vi "TLB Native Dynamic Events ver 0.18b.vi"() -> ()   [LabVIEW 2018]
uses:
  Labview Training Phase 2/Enum Controls/States for Action Engine.ctl
  TLB Type Definitions/State Type Definitions, for 0.26g versions and later 2.ctl
  TLB Type Definitions/Intruction Type Definitions.ctl
  TLB Type Definitions/Encoder cluster.ctl
  TLB Type Definitions/PING CLUSTER.ctl
  <vilib>/Studica/Studica Toolkit/NavX/NavX.lvlib
  <vilib>/Studica/Studica Toolkit/Background/DIO Channel.ctl
  Underlying VI's/NavX VI/navX type def.ctl
  <vilib>/Studica/Studica Toolkit/Background/I2C Channel.ctl
  TLB Type Definitions/Vision cluster.ctl
  <vilib>/NI_Real-Time Target Support.lvlib
  TLB Type Definitions/Stepper cluster.ctl
  Experimental VI's/Archived VI's/MOTOR CONTROL NO PID Type Def.ctl
  Underlying VI's/I2C Master VI/I2C MASTER Type Def.ctl
  Underlying VI's/I2C Master VI/I2C_MASTER_WRITE_NEW Type Def.ctl
  <vilib>/userdefined/High Color/IMAQdx.ctl
  Underlying VI's/I2C Master VI/Arduino_Interfacing.ctl
  TLB Type Definitions/Yaw Cluster.ctl
  TLB Type Definitions/Time cluster.ctl
  TLB Type Definitions/Y Stepper cluster.ctl
  Underlying VI's/Modified webcam FGV/Webcam AE.ctl
  Underlying VI's/Elasped Timer/Elapsed timer control.ctl
  Underlying VI's/Motor Control VI with PID/MOTOR CONTROL WITH PID AE DATA MODE TYPE DEF.ctl
  Underlying VI's/Motor Control VI with PID/MOTOR CONTROL WITH PID AE DIRECTION TYPE DEF.ctl
  TLB Type Definitions/IR Sensor Type Def.ctl
  <vilib>/myRIO/Common/Instrument Driver Framework/myRIO v1.0/AI/typedefs/AI Channels Enum.ctl
  <vilib>/myRIO/Common/Instrument Driver Framework/myRIO v1.0/AI/typedefs/AI Channels List.ctl
  TLB Type Definitions/Motor Speed Cluster.ctl
  Underlying VI's/IMAQ Create Reference AE/IMAQ Reference AE.ctl
  TLB Type Definitions/Line Sensor Cluster.ctl
  Underlying VI's/Line Sensor AE/Line Sensor AE Type Def.ctl
  <vilib>/Utility/RT CPU Load.ctl
panel:
  out "Arm IR Sensor":dbl
  out "Table obstruct":bool
  out "x-y":dbl
  out "Left IR Sensor":dbl
  out "Obstacle detected":bool
  out "Speed & distance":T1
  out "Object Center Coordinates":cluster{"x":sgl, "y":sgl}
  out "Object detection cluster":T2
  out "Time up flag":bool
  out "Task selection":u8
  in  "Object recognition mode":enum16{"Ball", "Soap", "Gel", "Pipe", "None"}(ring)
  out "NavX Readings":T3
  out "Arduino Data":T4
  out "CPU loads":T5[](array[typedef]) {"ISR (%)" format="%#.2f"; "Idle (%)" format="%#.2f"; "Background (%)" format="%#.2f"; "Normal (%)" format="%#.2f"; "Above Normal (%)" format="%#.2f"; "High (%)" format="%#.2g"; "Timed Structures (%)" format="%#.2g"; "Time Critical (%)" format="%#.2g"; "Total (%)" format="%#.2g"}
  out "TASK ENABLE":bool
  out "Rising Edge":bool
  in  "Green LED":bool
  out "I2C Error":errorcluster
  out "State Logic":T6=enum."Startup"
  out "elements":T7[](array[typedef])
  in  "STOP TASK":bool
  in  "OK Button":bool
  in  "STOP":bool
  out "error out":errorcluster
  out "Action Queue Items":i32
  out "State Logic Queue Items":i32
  out "Action Queues items":string[](array[string])=["Hardware reset", "Software reset", ""]
  out "Action State":string
  # "System Health Status Update"
  # "VISION"
  # "TLB FRAMEWORK STATUS"
  # "Test Programme written by Calvin Loke    Dated: 28 Aug 2019\nTest Programme revised by Dr Alex See   Dated 30 Aug 2019\n\nRevision date: 20/03/2020\nProgramme version:   TLB Native Dynamic Events ver 0.14a"
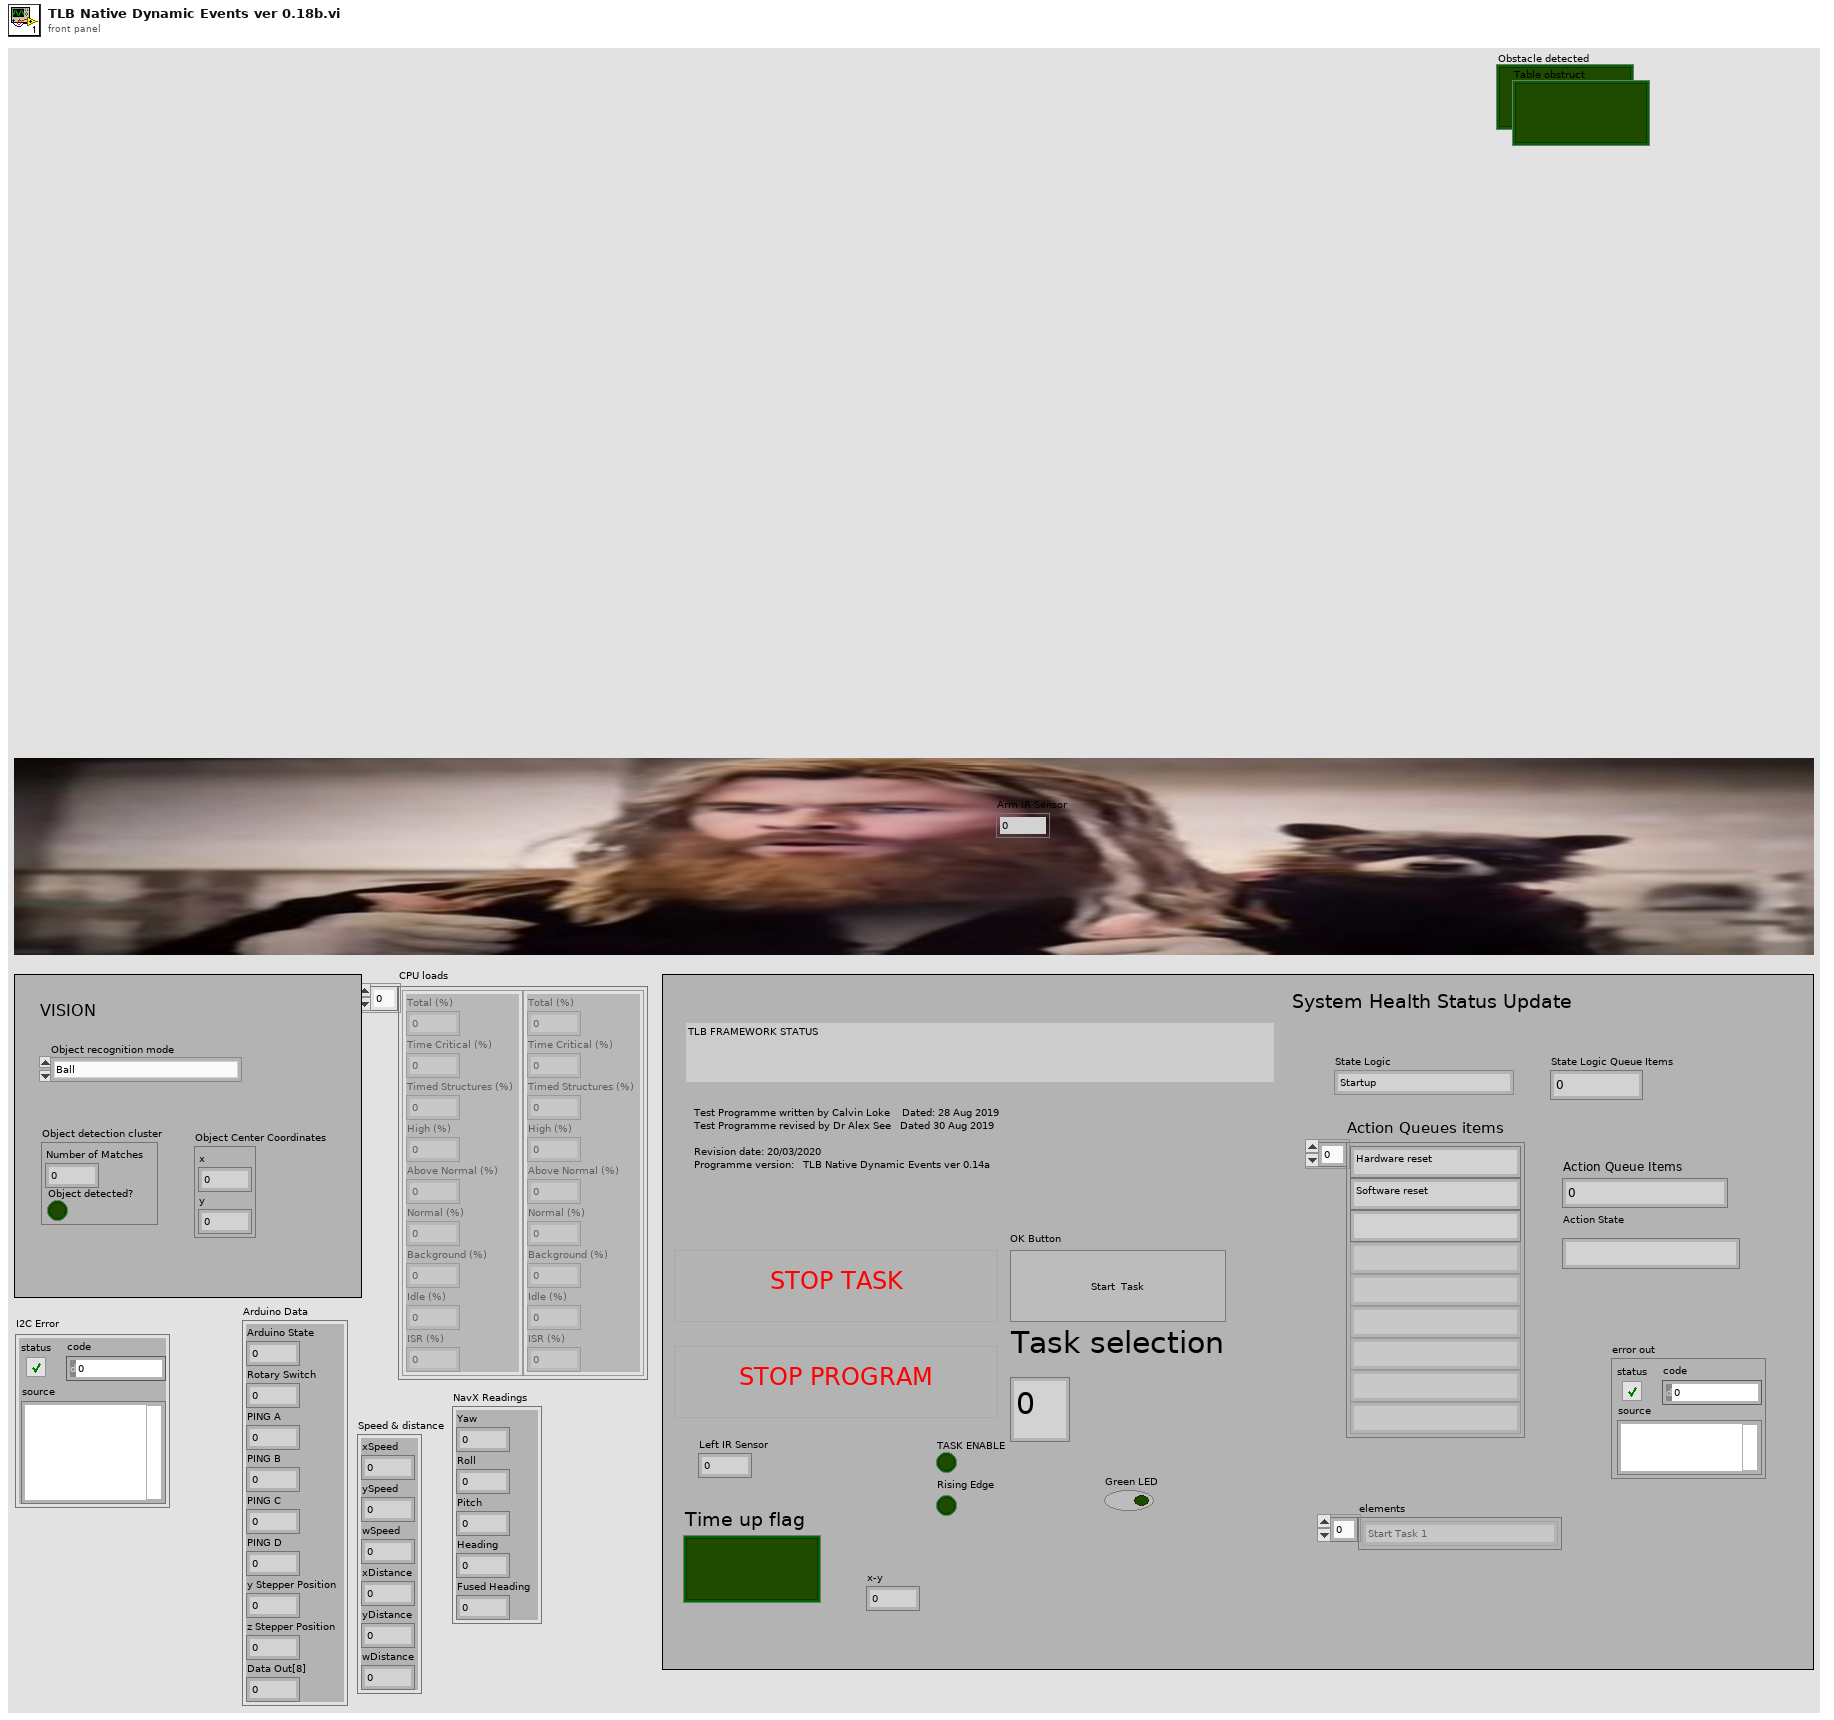
[diagram p1: front panel]
types:
  T1 = cluster{"xSpeed":dbl, "ySpeed":dbl, "wSpeed":dbl, "xDistance":dbl, "yDistance":dbl, "wDistance":dbl}
  T2 = cluster{"Number of Matches":i32, "Object detected?":bool}
  T3 = cluster{"Yaw":dbl, "Roll":dbl, "Pitch":dbl, "Heading":dbl, "Fused Heading":dbl}
  T4 = cluster{"Arduino State":u8, "Rotary Switch":u8, "PING A":u8, "PING B":u8, "PING C":u8, "PING D":u8, "y Stepper Position":u8, "z Stepper Position":u8, "Data Out[8]":u8}
  T5 = typedef "NI_Real-Time Target Support.lvlib/RT CPU Load.ctl" = cluster{"Total (%)":dbl, "Time Critical (%)":dbl, "Timed Structures (%)":dbl, "High (%)":dbl, "Above Normal (%)":dbl, "Normal (%)":dbl, "Background (%)":dbl, "Idle (%)":dbl, "ISR (%)":dbl}
  T6 = typedef "State Type Definitions, for 0.26g versions and later 2.ctl" = enum16{"None", "Startup", "Move to Angle", "True Stop", "Idle", "Shutdown", "Task 1A", "Task 1B", "Task 2:Raise Arm", "Task 2:Sensor Mode", "Task 2:Reverse Mode", "Task 3", "Task 4_A", "Task 4_B", "Task 4_C", "Task 4_D", "Task 5A", "Task 5B", "Task 5C", "Task 5D", "Task 5E: POSITION ARM", "Task 5F: ARM GRAB HEIGHT", "Task 5G: CLOSE CLAW", "Task 5H: RAISE ARM", "Task 6_A", "Task 6_B", "Task 7", "Task 8A: RAISE ARM", "Task 8B: MOVE TO BOX", "Task 8C: CAM BURST", "Task 8D: PROCESS IMAGE", "Task 8E: ROBOT ADJUST", "Task 8F: CAM BURST 2", "Task 8G: PROCESS IMAGE 2", "Task 8H: ARM ADJUST", "Task 8I: ARM GRAB HEIGHT", "Task 8J: CLOSE CLAW", "Task 8K: RAISE MY SWORD", "Task 9A: Raise Arm", "Task 9B: Rotate to Angle", "Task 9C: Detect Box", "Task 9D: MOVE FORWARD", "Task 9E: MOVE LEFT", "Task 9F: SCAN BOX", "Task 9G: MOVE RIGHT", "Task 9H: SCAN BOX 2", "Task 9I: ROTATE 90 CW", "Task 9J: FORWARD", "Task 9K: RAM WALL", "Task 9L: MOVE RIGHT", "Task 9M: SCAN BOX 3", "Task 9M: MOVE RIGHT", "Task 9N: SCAN BOX 4", "PENIS", "PENIS 2", "PENIS 3", "Task 9R: PROCESS COLOUR", "Task A1: Task 9 Open cam", "Task A2: Task 9 Move Arm", "Task A3: Task 9 Set Timer", "Task A4: Tasl 9 Capture images", "Task A5: Task 9 Close camera", "Task A6: Process Colour", "Task A7: Dispose Camera Buffer"}
  T7 = typedef "Intruction Type Definitions.ctl" = enum16{"None", "Start Task 1", "Start Task 2", "Start Task 3", "Start Task 4", "Start Task 5", "Start Task 6", "Start Task 7", "Start Task 8 - BALL", "Start Task 8 - Gel", "Start Task 8 - Pipe", "Start Task 8 - Soap", "Start Task 9", "Start Task A", "Start Task B", "Exit"}
  T8 = typedef "Line Sensor Cluster.ctl" = cluster{"Line Detected?":bool, "S1":dbl, "S2":dbl, "S3":dbl, "S4":dbl}
  T9 = typedef "Motor Speed Cluster.ctl" = cluster{"ySpeed":dbl, "xSpeed":dbl, "wSpeed":dbl}
  T10 = typedef "IR Sensor Type Def.ctl" = cluster{"Left IR Sensor":dbl, "Arm IR Sensor":dbl, "Bottom IR Sensor":dbl}
  T11 = typedef "Y Stepper cluster.ctl" = cluster{"yStepper desired":u8}
  T12 = typedef "Time cluster.ctl" = cluster{"Time up flag":bool, "SET TIME TO CHECK":dbl}
  T13 = typedef "Yaw Cluster.ctl" = cluster{"Yaw":dbl, "Compass":dbl}
  T14 = typedef "Stepper cluster.ctl" = cluster{"y Stepper Position":u8, "z Stepper Position":u8}
  T15 = typedef "DIO Channel.ctl" = enum16{"Not Connected", "A/DIO1", "A/DIO2", "A/DIO3", "A/DIO4", "A/DIO5", "A/DIO6", "A/DIO7", "A/DIO13", "B/DIO1", "B/DIO2", "B/DIO3", "B/DIO4", "B/DIO5", "B/DIO6", "B/DIO7", "B/DIO13", "C/DIO0", "C/DIO1", "C/DIO2", "C/DIO3", "C/DIO4", "C/DIO5", "C/DIO6", "C/DIO7"}
  T16 = typedef "Vision cluster.ctl" = cluster{"Recognized Object":bool, "Object X coordinate":dbl, "Object Y coordinate":dbl}
  T17 = typedef "PING CLUSTER.ctl" = cluster{"PING_A":u8, "PING_B":u8, "PING_C":u8, "PING_D":u8}
  T18 = typedef "Encoder cluster.ctl" = cluster{"xDistance":dbl, "yDistance":dbl, "wDistance":dbl}
  T19 = cluster{"DIO Channel":T15, "FPGA VI Reference Out":refnum<k20>}
  T20 = typedef "navX type def.ctl" = enum16{"Get i2C reference", "Read Values", "Zero Yaw"}
  T21 = typedef "Arduino_Interfacing.ctl" = enum16{"Initialize", "Write to Arduino", "Read From Arduino"}
  T22 = typedef "I2C Channel.ctl" = enum16{"Not Connected", "A", "B"}
  T23 = typedef "States for Action Engine.ctl" = enum16{"Initialize", "Write", "Read"}
  T24 = cluster{"I2C Ref Out":cluster{"I2C Channel":T22, "FPGA VI Reference Out":refnum<k20>}, "Connected":bool, "Slave Address (7-bit)":u8, "Registry":u8[]}
  T25 = typedef "Intruction Type Definitions.ctl" = enum16{"None", "Start Task 1", "Start Task 2", "Start Task 3", "Start Task 4", "Start Task 5", "Start Task 6", "Start Task 7", "Start Task 8", "Start Task 9", "Start Task A", "Start Task B", "Exit"}
  T26 = typedef "State Type Definitions.ctl" = enum16{"None", "Startup", "Move to Angle", "True Stop", "Idle", "Shutdown", "Task 1", "Task 2:Raise Arm", "Task 2:Sensor Mode", "Task 2:Reverse Mode", "Task 3", "Task 4_A", "Task 4_B", "Task 4_C", "Task 4_D", "Task 5A: ARM CAM HEIGHT", "Task 5B: MOVE TO BOX", "Task 5C: CAM BURST", "Task 5D: PROCESS IMAGE", "Task 5E: POSITION ARM", "Task 5F: ARM GRAB HEIGHT", "Task 5G: CLOSE CLAW", "Task 5H: RAISE ARM", "Task 6_A", "Task 6_B", "Task 7", "Task 8A: RAISE ARM", "Task 8B: MOVE TO BOX", "Task 8C: CAM BURST", "Task 8D: PROCESS IMAGE", "Task 8E: ROBOT ADJUST", "Task 8F: CAM BURST 2", "Task 8G: PROCESS IMAGE 2", "Task 8H: ARM ADJUST", "Task 8I: ARM GRAB HEIGHT", "Task 8J: CLOSE CLAW", "Task 8K: RAISE MY SWORD", "Task 9A: Raise Arm", "Task 9B: Rotate to Angle", "Task 9C: Rotation alignmnet", "Task 9D: Move Forward", "Task A: RAISE ARM TO HEIGHT", "Task A: MOVE FORWARD"}
  T27 = typedef "MOTOR CONTROL WITH PID AE DIRECTION TYPE DEF.ctl" = enum16{"y-axis movement", "x-axis movement", "rotation", "stop", "reset encoders"}
  T28 = typedef "MOTOR CONTROL WITH PID AE DATA MODE TYPE DEF.ctl" = enum16{"Init AE", "Write to AE", "Read from AE"}
  T29 = typedef "Line Sensor AE Type Def.ctl" = enum16{"INIT AE", "READ FROM LINE SENSORS"}
  T30 = typedef "IMAQ Reference AE.ctl" = enum16{"Initialize AE", "Get IMAQ Reference", "Dispose Processing Buffer"}
  T31 = typedef "Elapsed timer control.ctl" = enum16{"Start", "Pause", "Initialize"}
  T32 = typedef "I2C_MASTER_WRITE_NEW Type Def.ctl" = enum16{"Ultrasonic sensors", "Stepper origin", "zStepper 13.3k", "zStepper 13k", "zStepper 12k", "zStepper 11k", "zStepper 10k", "zStepper 9k", "zStepper 8k", "zStepper 7k", "zStepper 6k", "zStepper 5k", "zStepper 4k", "zStepper 3k", "zStepper 2k", "zStepper 1k", "zStepper 900", "zStepper 800", "zStepper 700", "zStepper 600", "zStepper 500", "zStepper 400", "zStepper 300", "zStepper 200", "zStepper 100", "zStepper 0", "yStepper control", "Open Claw", "Close Claw", "Soft Reset"}
  T33 = typedef "Webcam AE.ctl" = enum16{"Initialize Camera", "Open Camera", "Continuous Acquisition", "Close Camera", "Retrieve Image", "Dispose Camera Image Buffer"}
  T34 = typedef "IMAQdx.ctl" = refnum<k21>
  T35 = typedef "Webcam AE.ctl" = enum16{"Initialize Camera", "Open Camera", "Continuous Acquisition", "Close Camera", "Retrieve Image", "Dispose Image Buffers"}
  T36 = typedef "IMAQ Reference AE.ctl" = enum16{"Initialize AE", "Get IMAQ Reference", "Destroy ALL IMAQ"}
  T37 = typedef "MOTOR CONTROL NO PID Type Def.ctl" = enum16{"Init", "Front Back", "Left Right", "Rotate", "Stop", "Latch"}
  T38 = typedef "AI Channels List.ctl" = T39[]
  T39 = typedef "AI Channels Enum.ctl" = enum16{"Not Connected", "AudioIn/Left", "AudioIn/Right", "C/AI0", "C/AI1", "A/AI0", "A/AI1", "A/AI2", "A/AI3", "A/AI4", "A/AI5", "A/AI6", "A/AI7", "B/AI0", "B/AI1", "B/AI2", "B/AI3", "B/AI4", "B/AI5", "B/AI6", "B/AI7", "AI/AI0", "AI/AI1", "AI/AI2", "AI/AI3", "A/AI0 (DIFF)", "A/AI1 (DIFF)", "A/AI2 (DIFF)", "A/AI3 (DIFF)", "B/AI0 (DIFF)", "B/AI1 (DIFF)", "B/AI2 (DIFF)", "B/AI3 (DIFF)"}
  T40 = cluster{"S1":dbl, "S2":dbl, "S3":dbl, "S4":dbl, "Array[4]":dbl, "Array[5]":dbl, "Array[6]":dbl, "Array[7]":dbl, "Array[8]":dbl}
  T41 = typedef "I2C MASTER Type Def.ctl" = enum16{"Last State", "Mode 0", "Mode 1", "Mode 2", "Mode 3", "Mode 4", "Mode 5", "Mode 6", "Mode 7", "Mode 8", "Mode 9", "Mode 10"}
  T42 = typedef "IMAQ Image.ctl" = refnum<image>
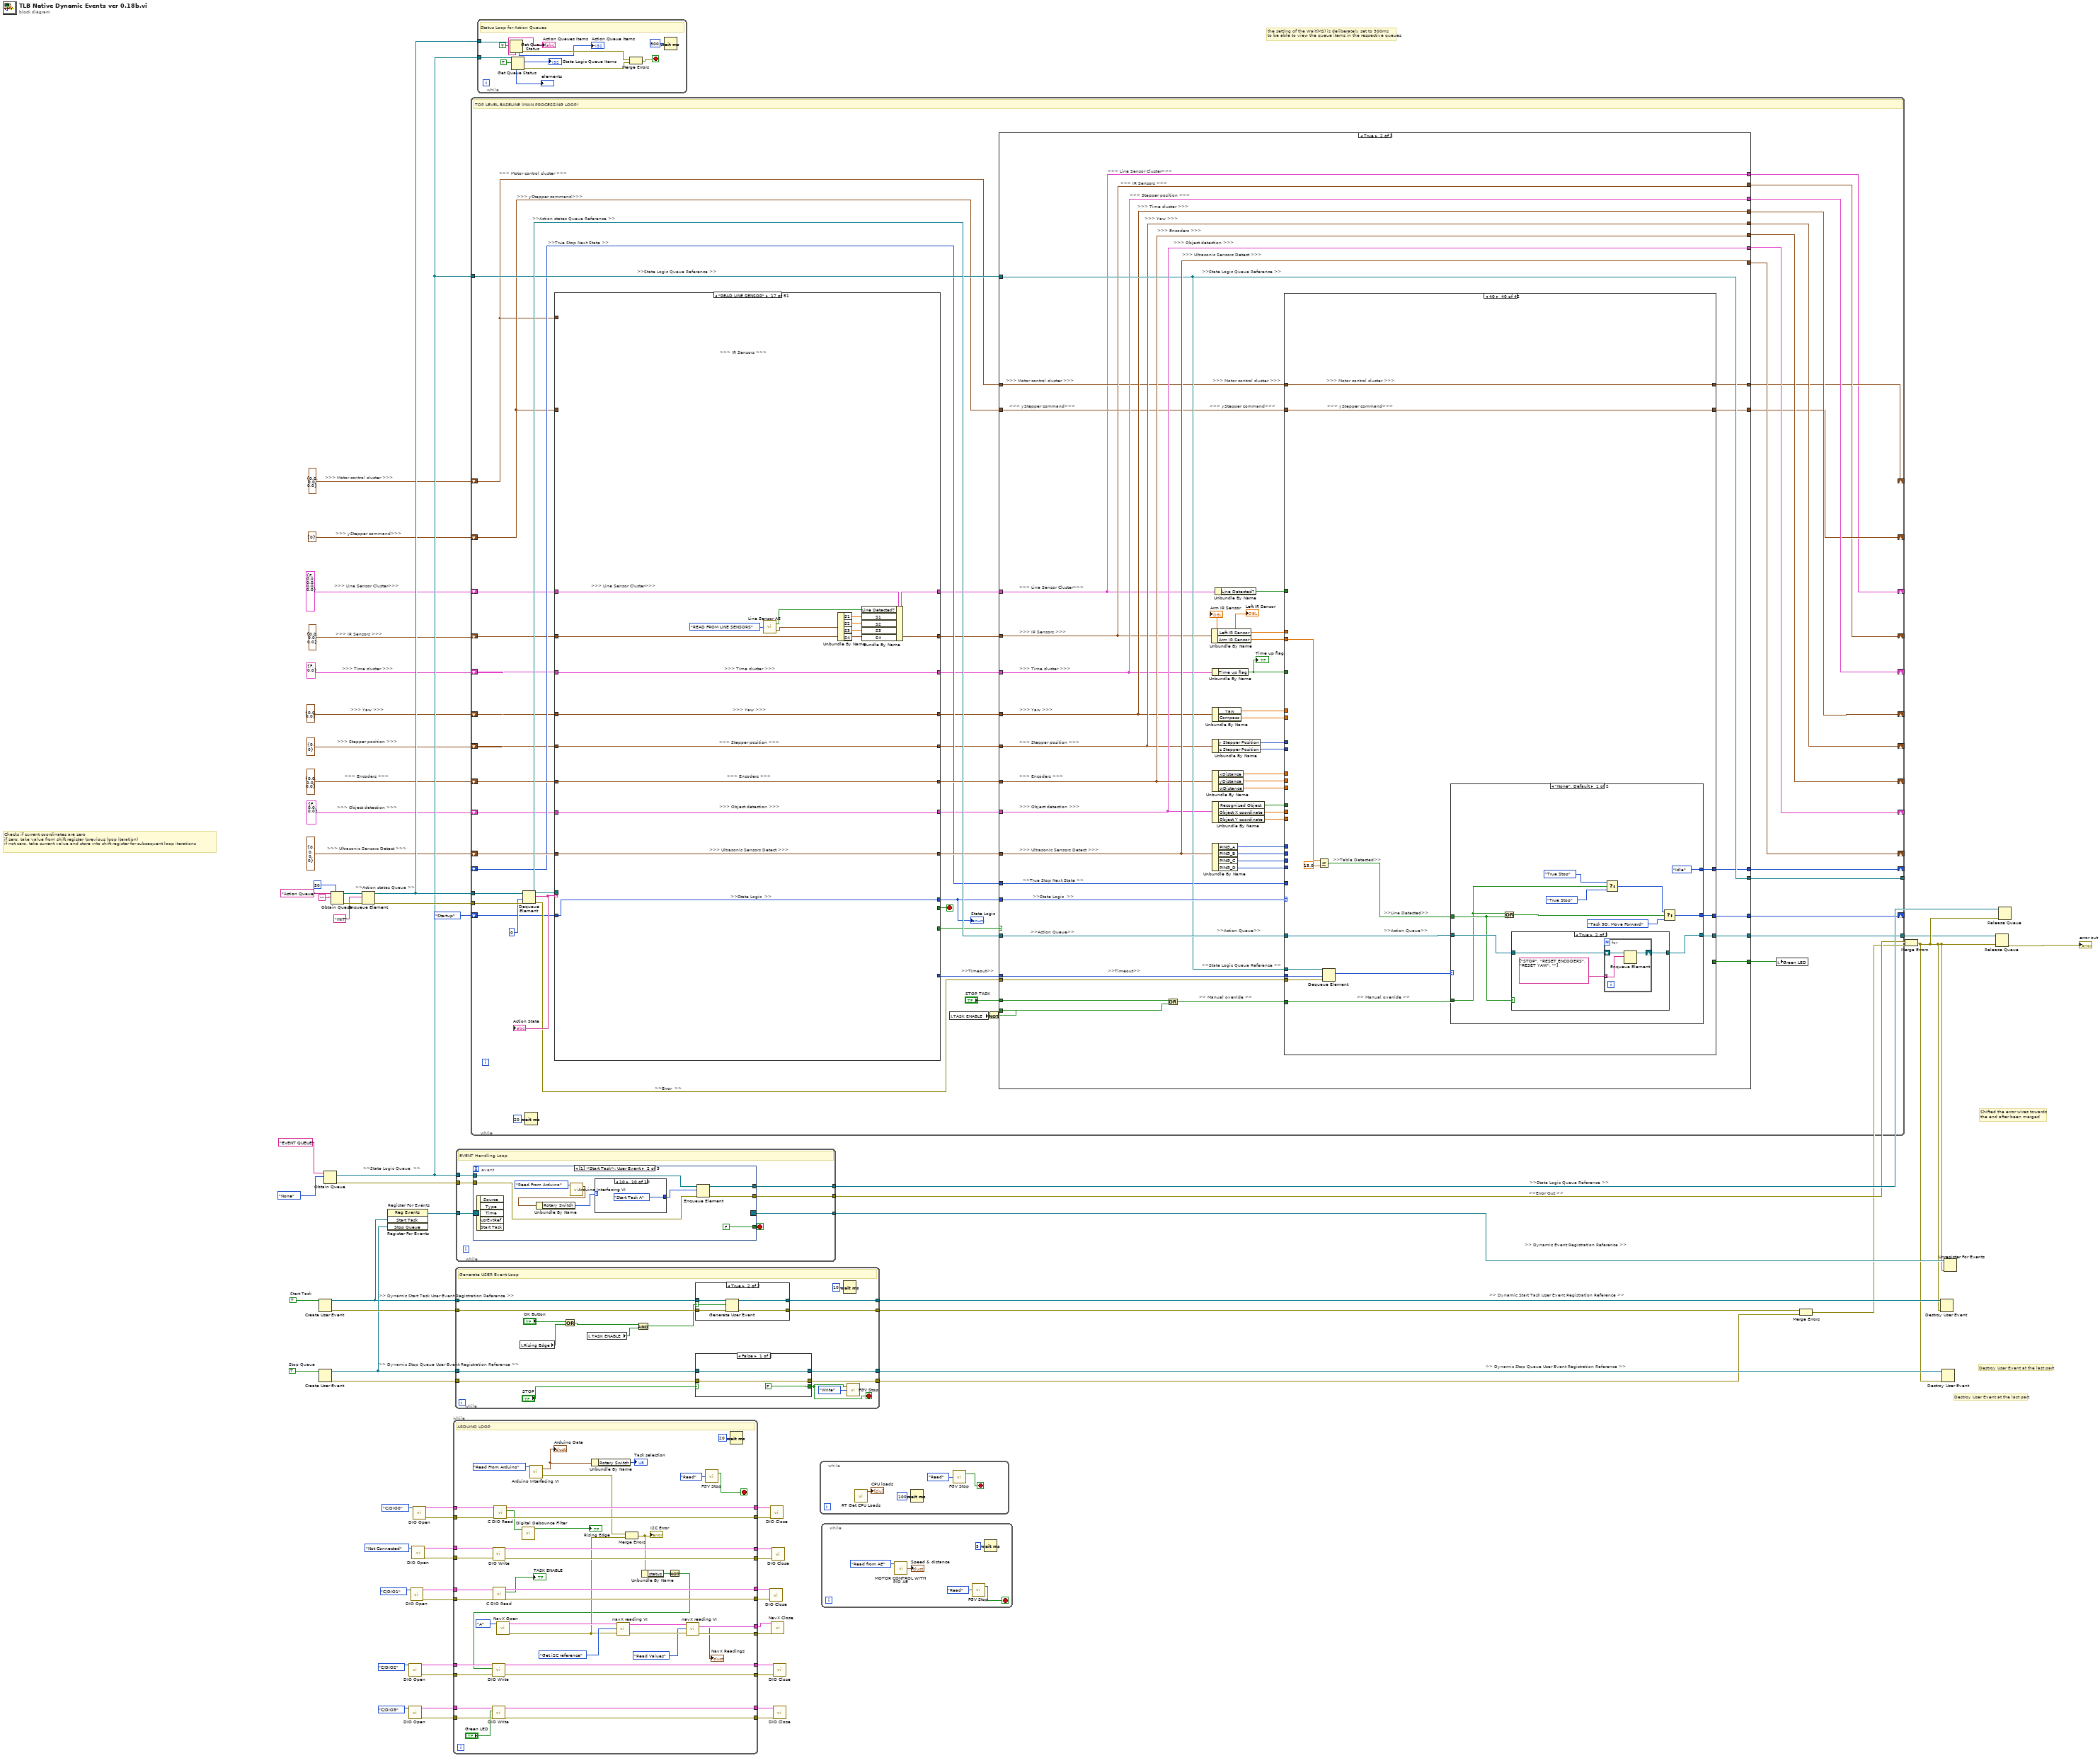
[diagram p0: block diagram]
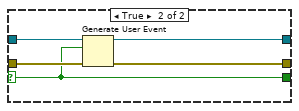
[diagram p2: hidden frame]
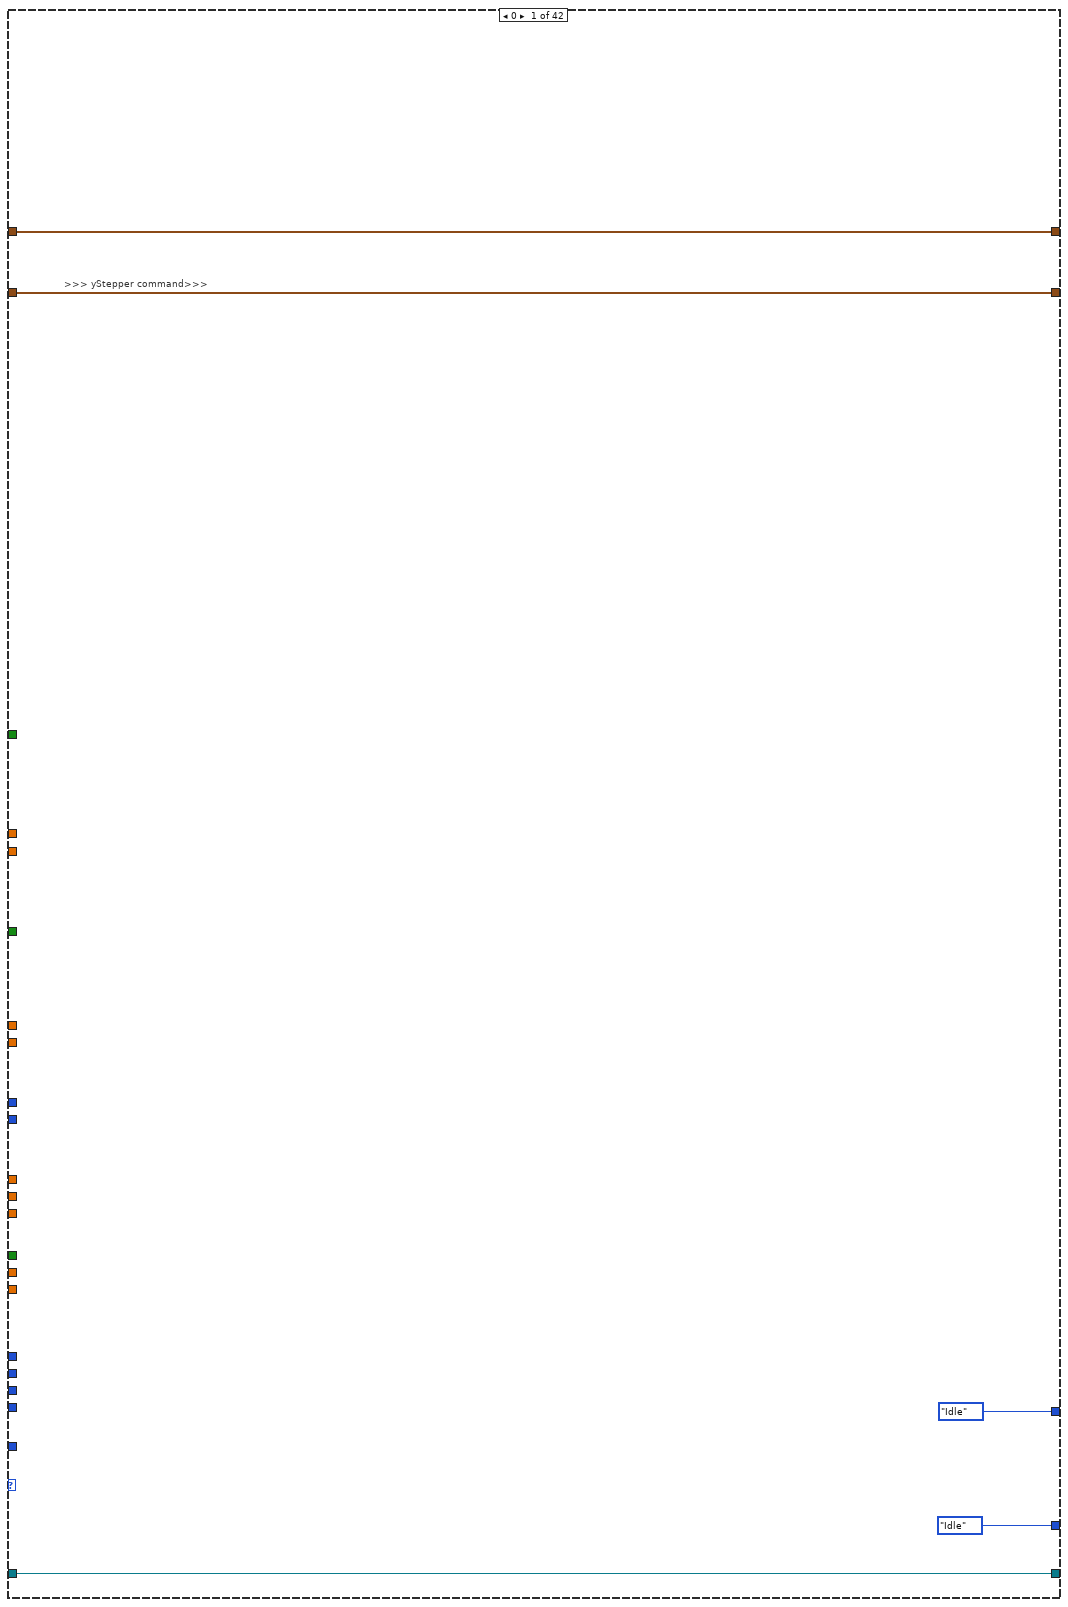
[diagram p5: hidden frame]
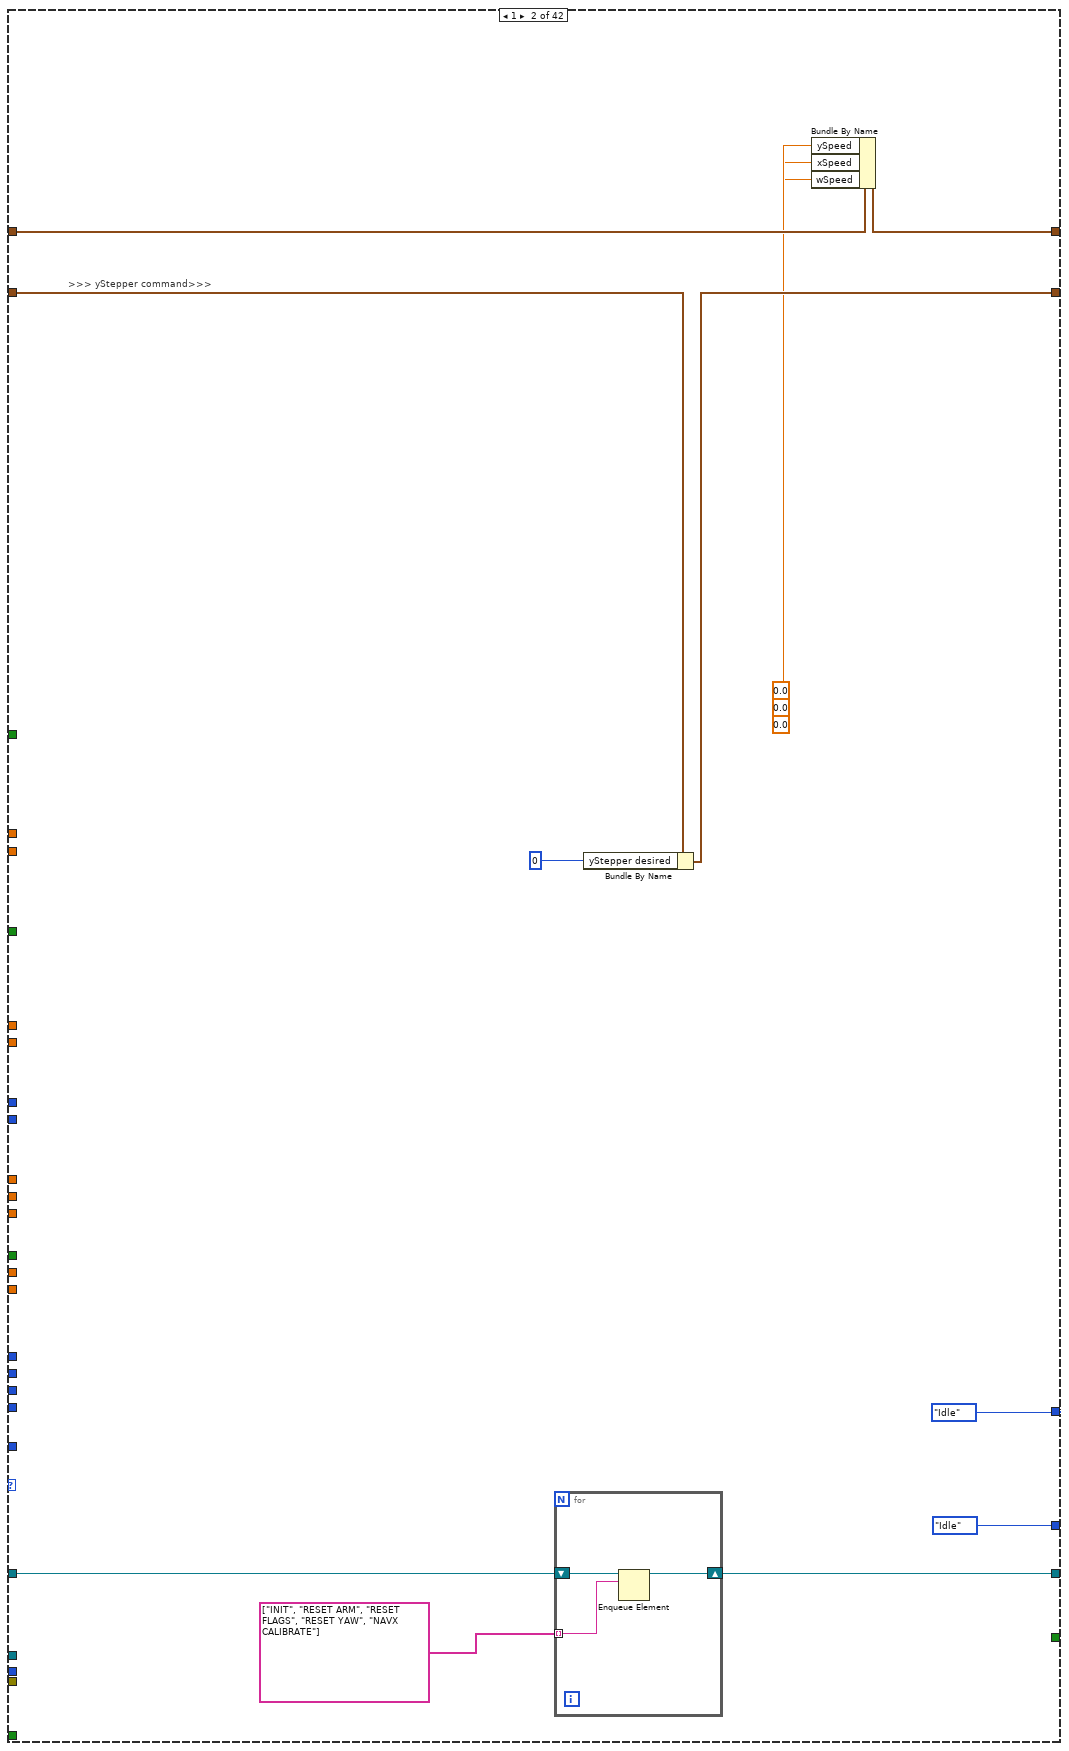
[diagram p6: hidden frame]
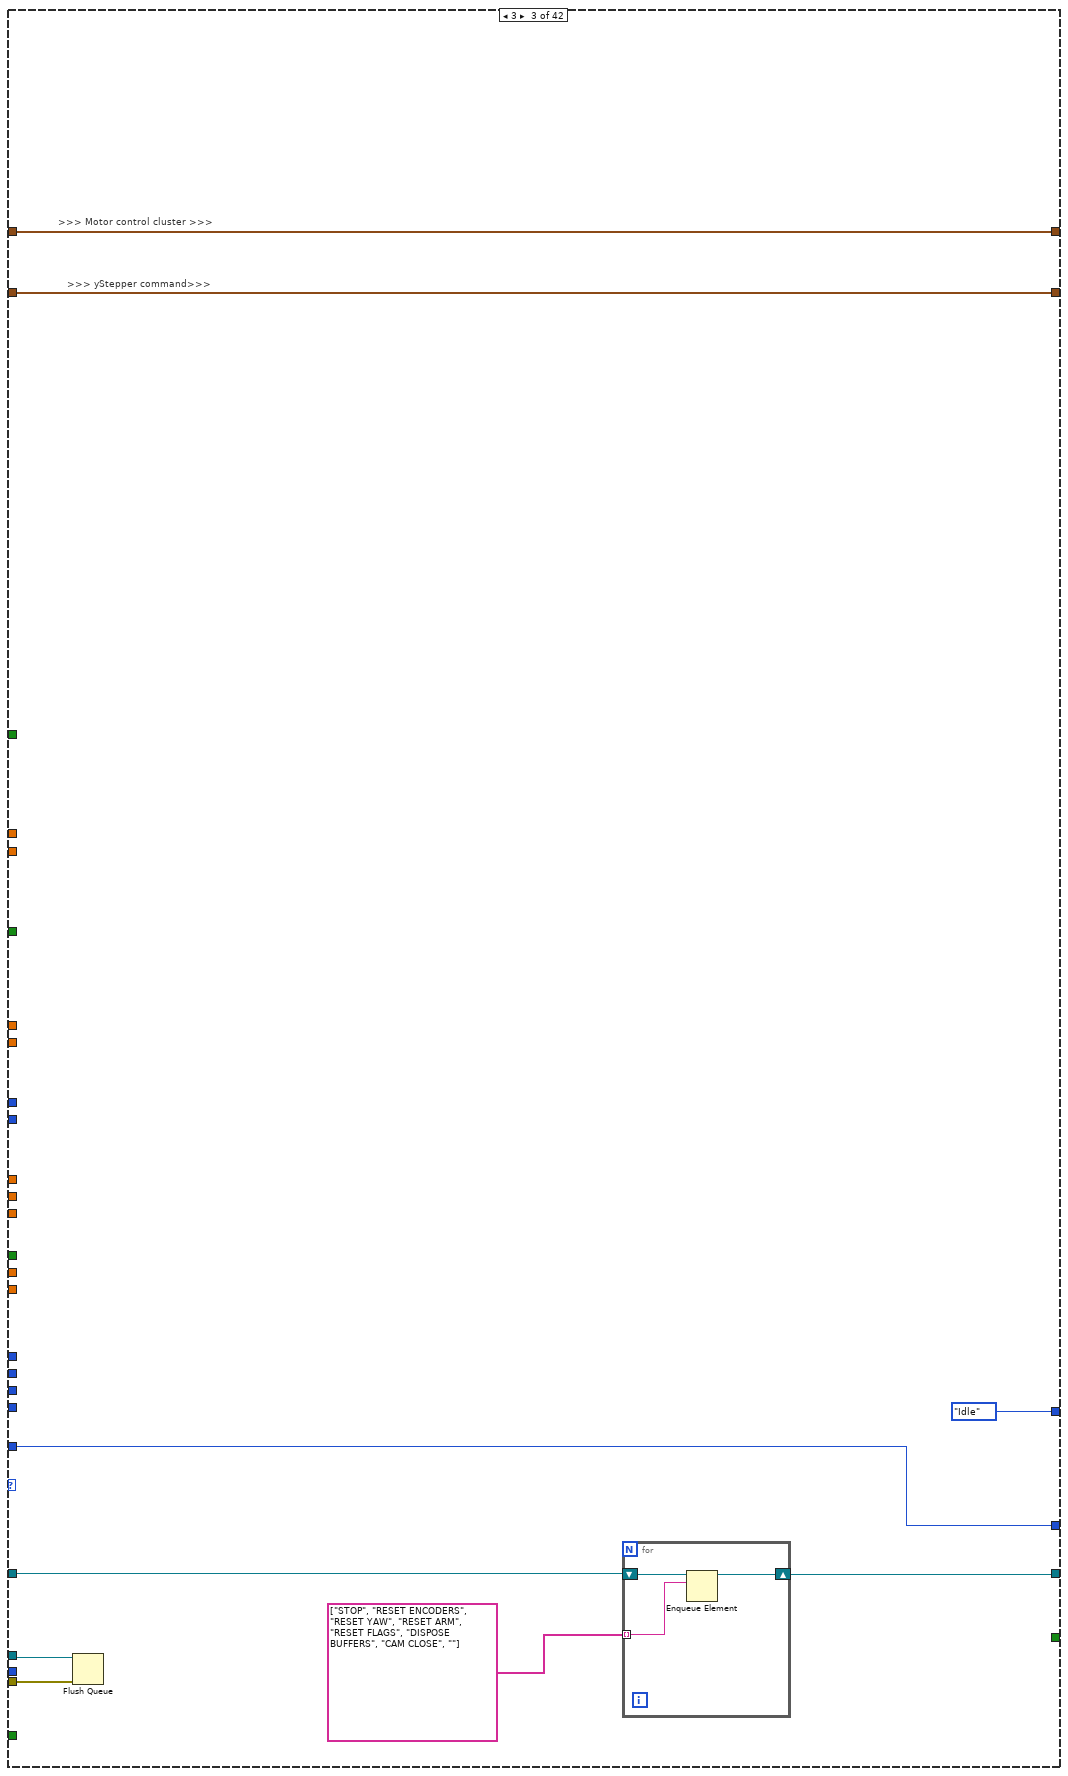
[diagram p7: hidden frame]
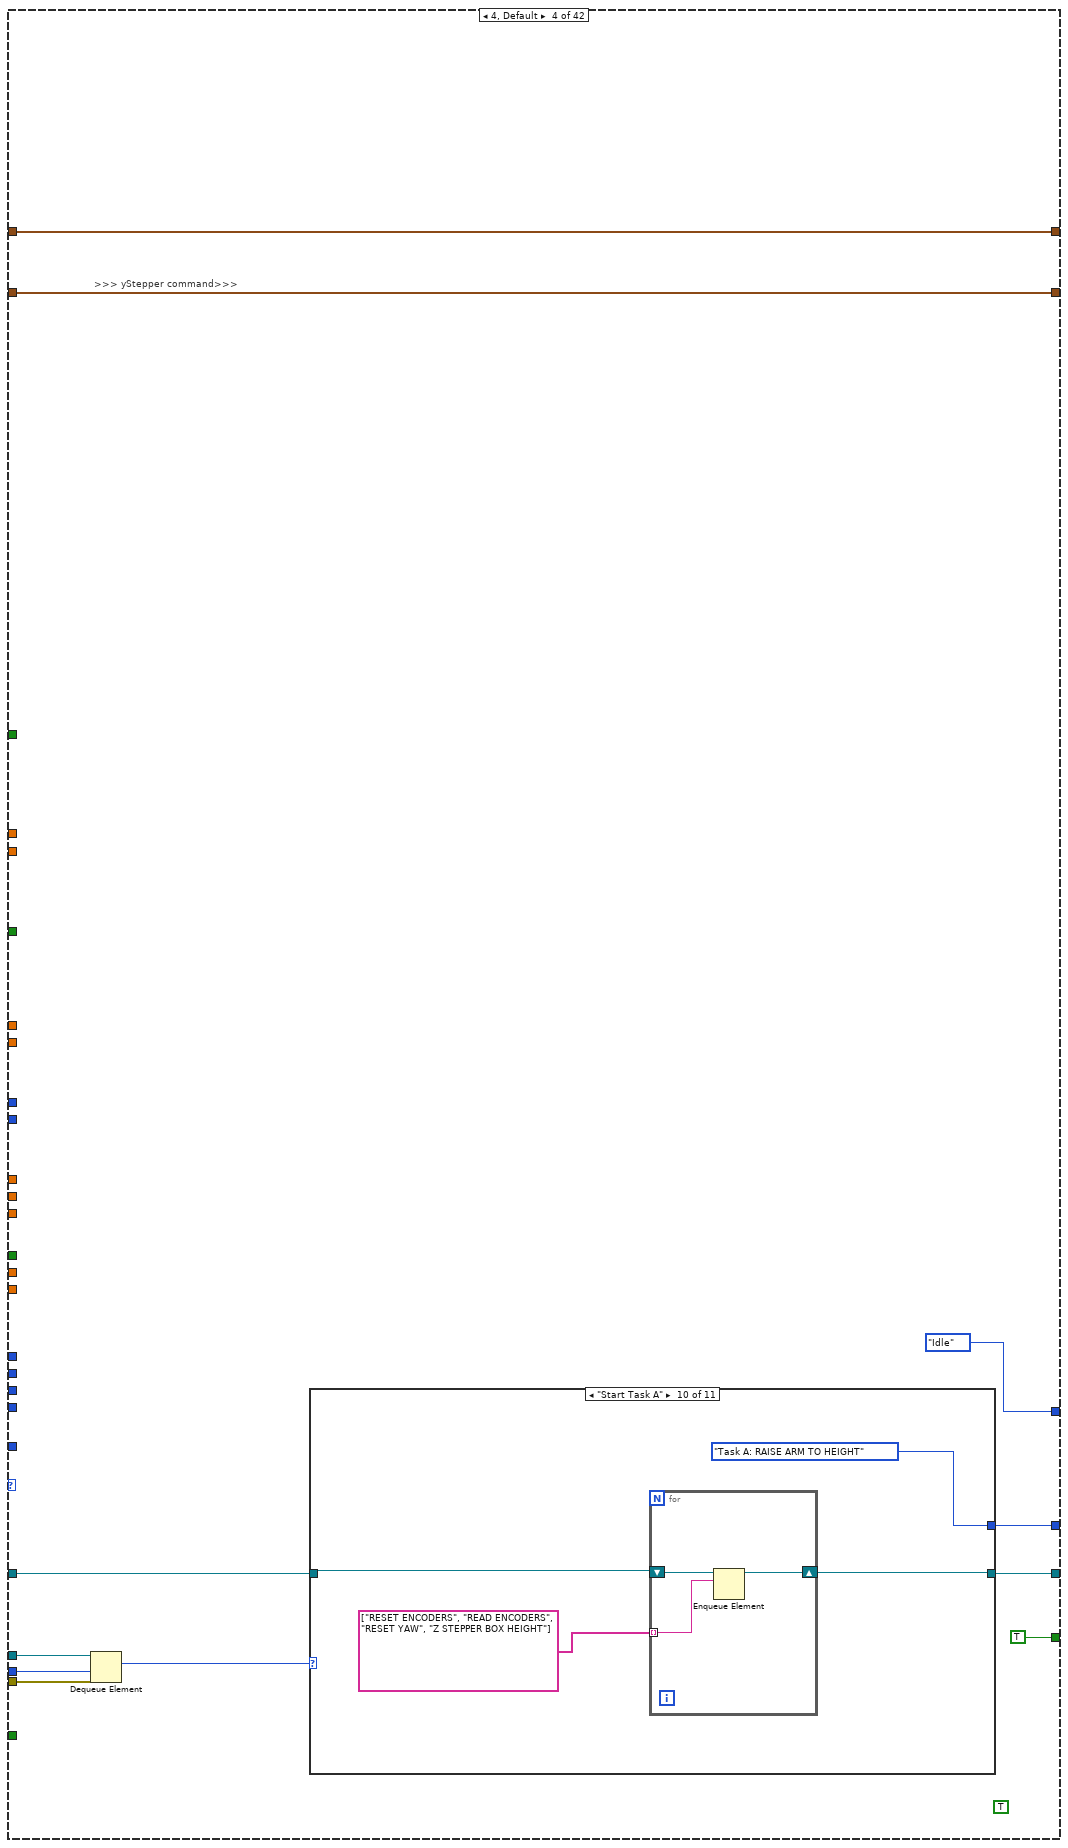
[diagram p8: hidden frame]
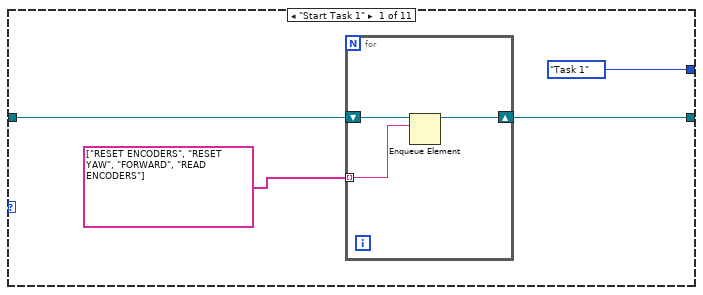
[diagram p9: hidden frame]
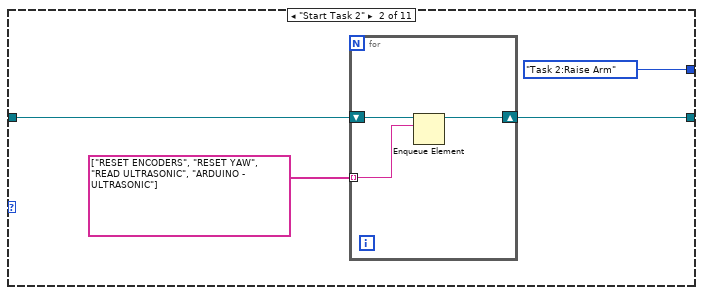
[diagram p10: hidden frame]
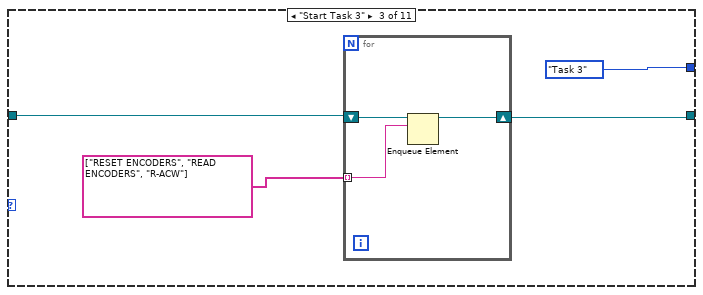
[diagram p11: hidden frame]
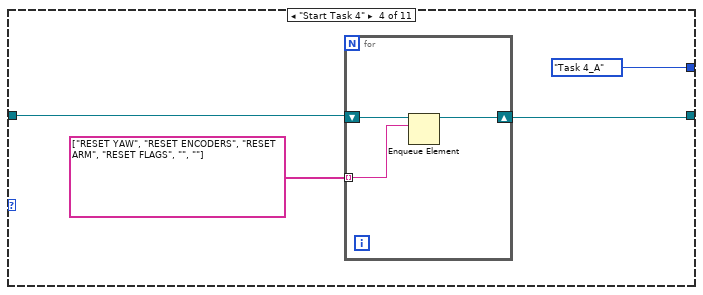
[diagram p12: hidden frame]
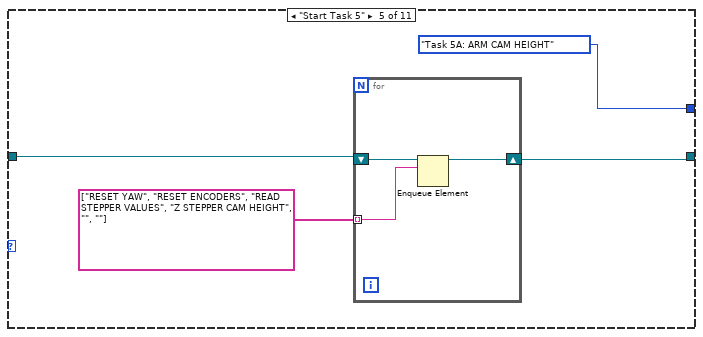
[diagram p13: hidden frame]
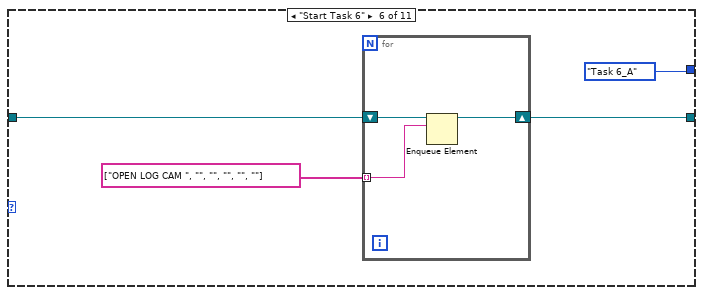
[diagram p14: hidden frame]
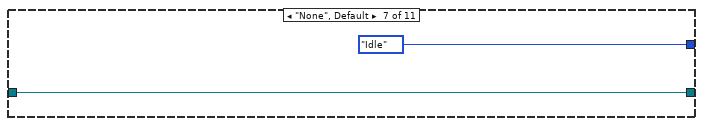
[diagram p15: hidden frame]
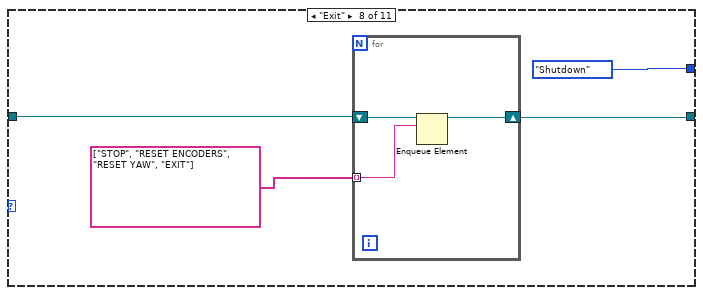
[diagram p16: hidden frame]
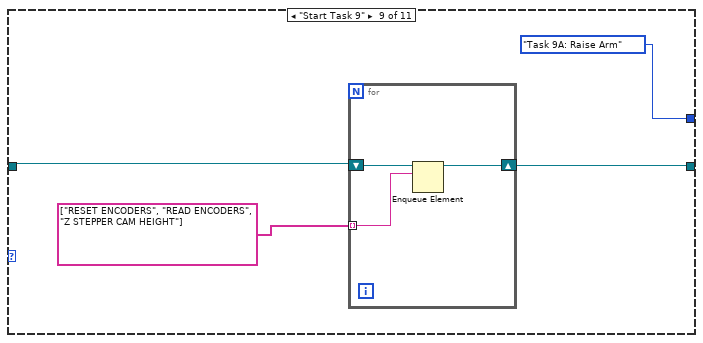
[diagram p17: hidden frame]
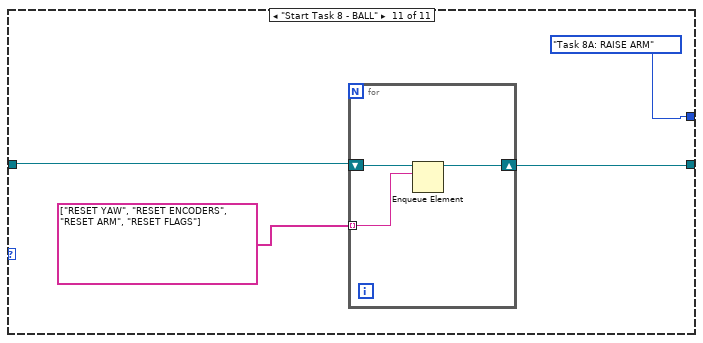
[diagram p18: hidden frame]
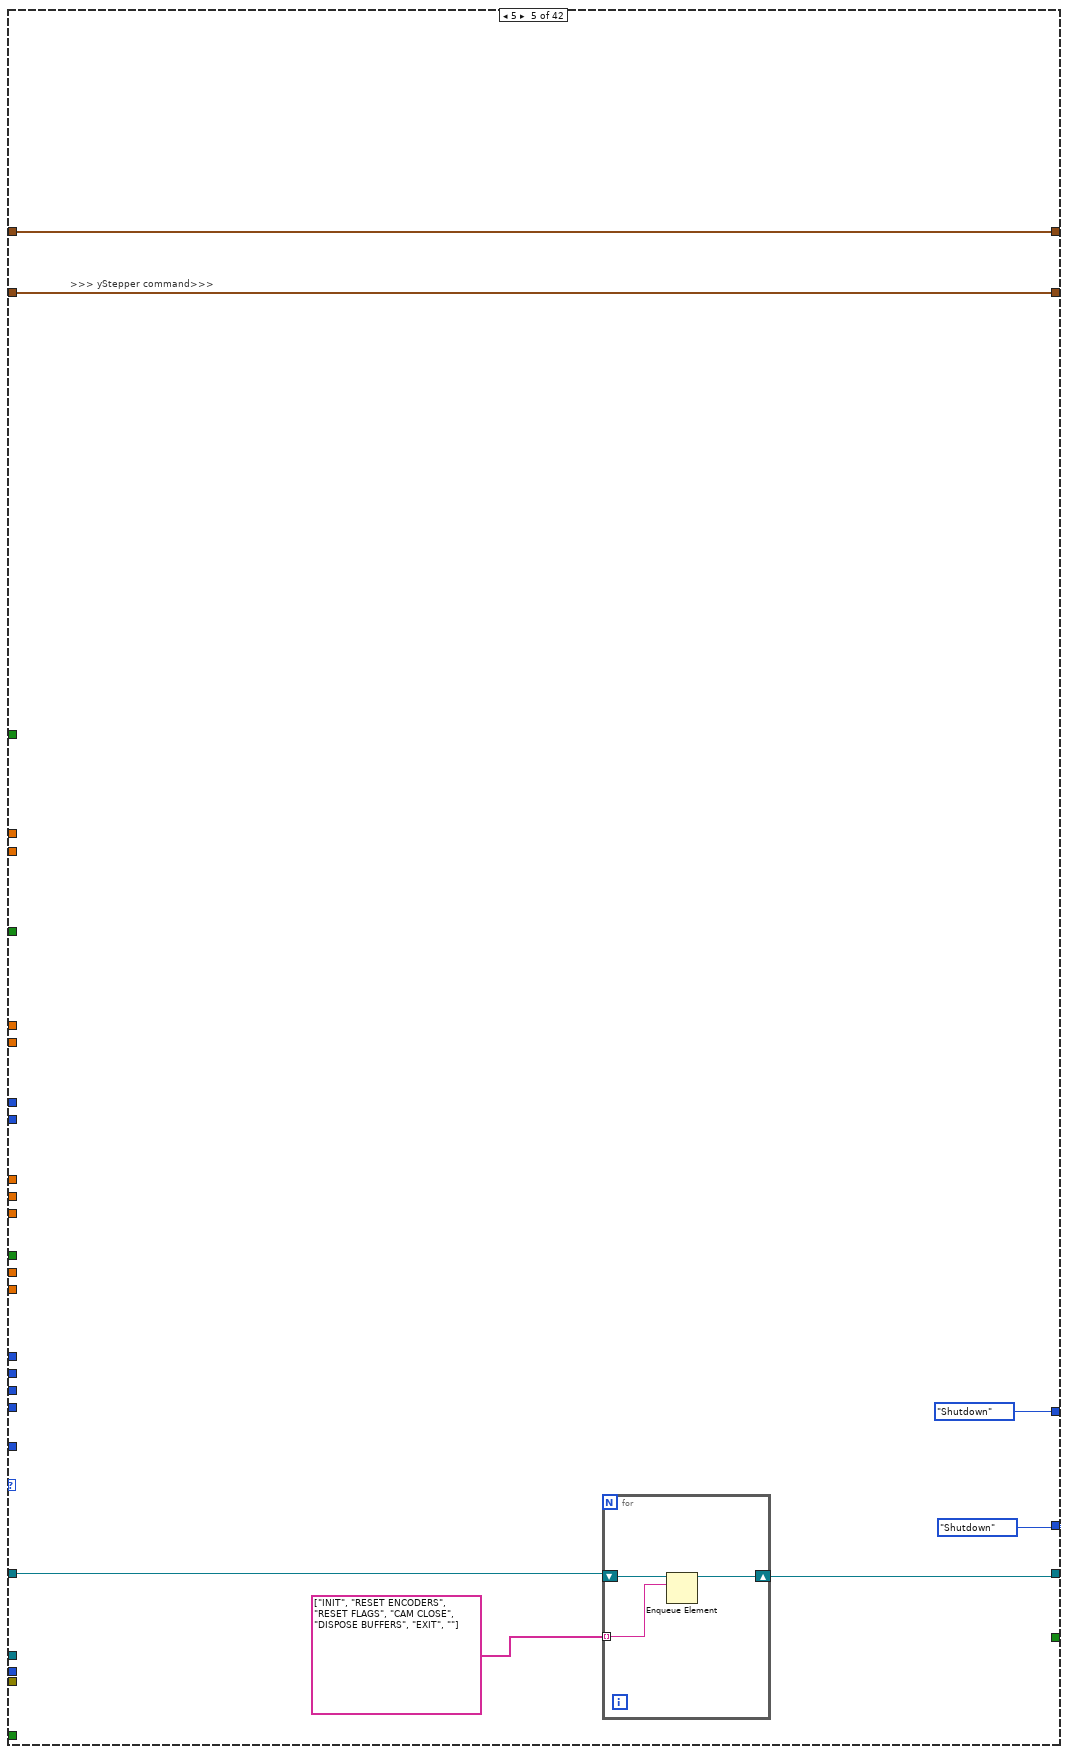
[diagram p19: hidden frame]
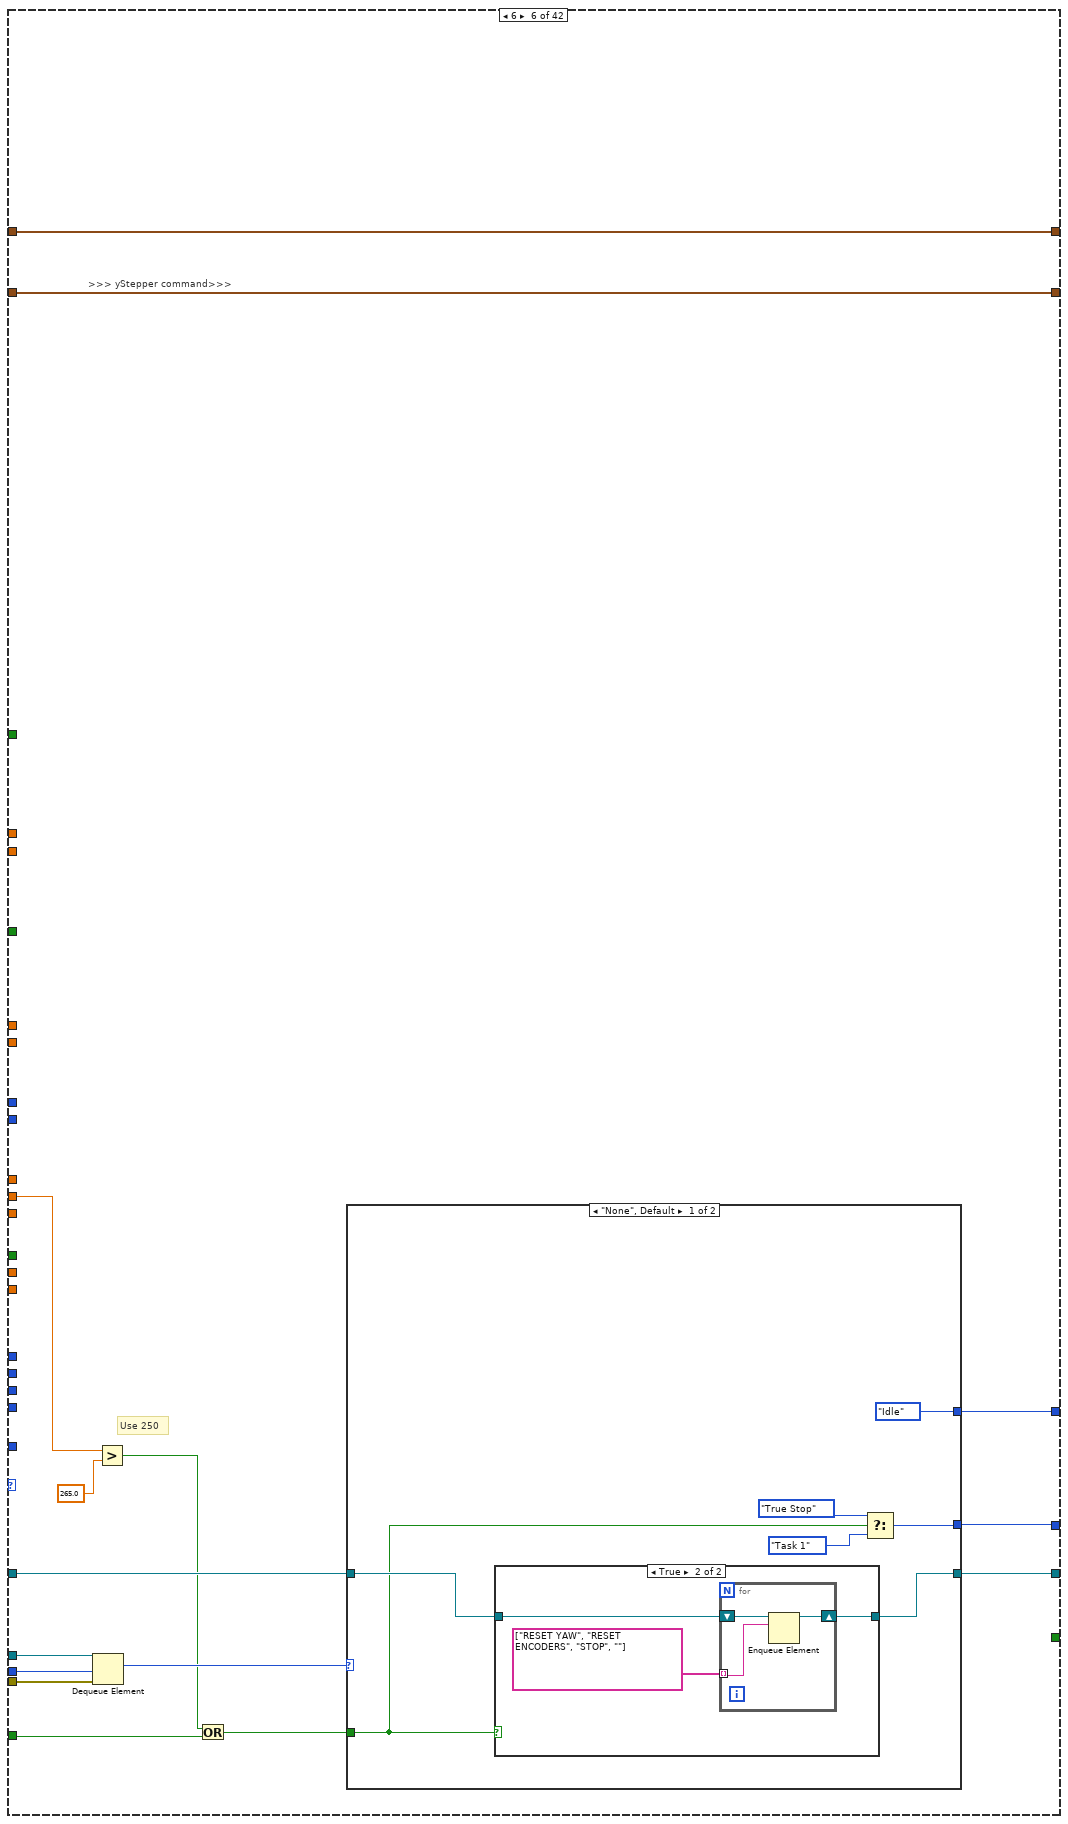
[diagram p20: hidden frame]
diagram:
  w68 = TRUE  # Stop Queue
  w67 = TRUE  # Start Task
  # ">>> Line Sensor Cluster>>>"
  # ">>> Motor control cluster >>>"
  # ">>> IR Sensors >>>"
  # "Checks if current coordinates are zero\nif zero, take value from shift register (previous loop iteration)\nif not zero, take current value and store into shift register for subsequent loop iterations"
  # ">>> yStepper command>>>"
  # ">>> Time cluster >>>"
  # ">>> Yaw >>>"
  # ">>> Stepper position >>>"
  # ">>> Encoders >>>"
  # ">>> Object detection >>>"
  # ">>> Ultrasonic Sensors Detect >>>"
  # "the setting of the Wait(MS) is deliberately set to 500ms\nto be able to view the queue items in the respective queues"
  # ">>Error Out >>"
  # ">> Dynamic Stop Queue User Event Registration Reference >>"
  # ">> Dynamic Start Task User Event Registration Reference >>"
  # ">> Dynamic Stop Queue User Event Registration Reference >>"
  # ">> Dynamic Start Task User Event Registration Reference >>"
  # ">> Dynamic Event Registration Reference >>"
  # ">>Action states Queue >>"
  # ">>State Logic Queue  >>"
  # ">>State Logic Queue Reference >>"
  # "Destroy User Event at the last part"
  # "Destroy User Event at the last part"
  # "Shifted the error wires towards\nthe end after been merged"
  n1 = Create User Event(user event datatype=w67) -> (user event=w59:refnum<user-event>, error out=w64:errorcluster)  [unwired: 1 in]
  n2 = Create User Event(user event datatype=w68) -> (user event=w60:refnum<user-event>, error out=w63:errorcluster)  [unwired: 1 in]
  n3 = Obtain Queue(name (unnamed)="EVENT QUEUE", element data type=Intruction_Type_Definitions."None" ("Enum")) -> (queue out=w45:refnum<queue>, error out=w51:errorcluster)  [unwired: 3 in, 1 out]
  n4 = Obtain Queue(max queue size (-1, unlimited)=50, name (unnamed)="Action Queue", element data type="") -> (queue out=w54:refnum<queue>, error out=w50:errorcluster)  [unwired: 2 in, 1 out]
  n5 = Enqueue Element(queue=w54, element="INIT", error in (no error)=w50) -> (queue out=w46:refnum<queue>, error out=w49:errorcluster)  [unwired: 1 in, 1 out]
  n6 = register-events "Register For Events"(w59, w60) -> (reference out=w58:refnum<event-registration>)  [unwired: 2 in, 1 out]
  n7 = call <vilib>:"DIO Open.vi"("DIO Channel"=DIO_Channel."C/DIO2") -> ("error out"=w18:errorcluster, "DIO Info Out"=w19:T19)  [unwired: 9 in]
  n8 = call <vilib>:"DIO Open.vi"("DIO Channel"=DIO_Channel."C/DIO3") -> ("error out"=w13:errorcluster, "DIO Info Out"=w14:T19)  [unwired: 9 in]
  n9 = call <vilib>:"DIO Open.vi"("DIO Channel"=DIO_Channel."C/DIO1") -> ("error out"=w23:errorcluster, "DIO Info Out"=w24:T19)  [unwired: 9 in]
  n10 = call <vilib>:"DIO Open.vi"("DIO Channel"=DIO_Channel."Not Connected") -> ("error out"=w28:errorcluster, "DIO Info Out"=w30:T19)  [unwired: 9 in]
  n11 = call <vilib>:"DIO Open.vi"("DIO Channel"=DIO_Channel."C/DIO0") -> ("error out"=w33:errorcluster, "DIO Info Out"=w36:T19)  [unwired: 9 in]
  n12 = while {
    tunnel: w36 -> [w109]
    tunnel: [w108] -> w34
    tunnel: w33 -> [w107]
    tunnel: [w106] -> w32
    tunnel: w30 -> [w103]
    tunnel: [w102] -> w29
    tunnel: w28 -> [w101]
    tunnel: [w100] -> w27
    tunnel: [w99] -> w25
    tunnel: w24 -> [w98]
    tunnel: w23 -> [w97]
    tunnel: [w96] -> w22
    tunnel: w19 -> [w90]
    tunnel: w18 -> [w89]
    tunnel: [w88] -> w17
    tunnel: [w87] -> w16
    tunnel: w14 -> [w86]
    tunnel: w13 -> [w85]
    tunnel: [w84] -> w12
    tunnel: [w83] -> w11
    tunnel: [w77] -> w8
    tunnel: [w76] -> w9
    stop <- w111 stop-if-true
    # "ARDUINO LOOP"
    n13 = call <vilib>:"DIO Write.vi"("error in (no error)"=w85, "Input"="Green LED", "DIO Info In"=w86) -> ("error out"=w83:errorcluster, "DIO Info Out"=w84:T19)  [unwired: 7 in]
    n14 = call <vilib>:"DIO Write.vi"("error in (no error)"=w101, "DIO Info In"=w103) -> ("error out"=w100:errorcluster, "DIO Info Out"=w102:T19)  [unwired: 8 in]
    n15 = call <vilib>:"C DIO Read.vi"("error in (no error)"=w97, "DIO Info In in"=w98) -> ("error out"=w96:errorcluster, "IN"=→"TASK ENABLE":bool, "DIO Info In out"=w99:T19)  [unwired: 7 in]
    n16 = call <vilib>:"C DIO Read.vi"("error in (no error)"=w107, "DIO Info In in"=w109) -> ("error out"=w106:errorcluster, "IN"=w105:bool, "DIO Info In out"=w108:T19)  [unwired: 7 in]
    n17 = call <vilib>:"NavX Open.vi"("I2C Channel"=I2C_Channel."A") -> ("error out"=w92:errorcluster, "NavX Info"=w94:T24)  [unwired: 9 in]
    n18 = call "Digital Debounce Filter.vi"("Boolean input"=w105) -> ("Rising Edge"=→"Rising Edge":bool)  [unwired: 1 in, 2 out]
    n19 = call "Arduino Interfacing VI.vi"("AE Mode"=Arduino_Interfacing."Read From Arduino") -> ("error out"=w80:errorcluster, "Arduino Data"=w73:T4)  [unwired: 3 in]
    "Arduino Data" <- w73
    n20 = Unbundle By Name(w73) -> ("Rotary Switch"=→"Task selection":u8)
    n21 = call "navX reading VI.vi"("NavX Info In"=w94, "Mode"=navX_type_def."Get i2C reference", "error in (no error)"=w92) -> ("NavX Info Out"=w79:T24, "Error Out"=w78:errorcluster)  [unwired: 2 out]
    n22 = Merge Errors(w80, w92) -> (w71:errorcluster)
    "I2C Error" <- w71
    n23 = Unbundle By Name(w71) -> ("status"=w70:bool)
    n24 = Not(x=w70) -> (.not. x?=w69:bool)
    n25 = call <vilib>:"DIO Write.vi"("error in (no error)"=w89, "Input"=w69, "DIO Info In"=w90) -> ("error out"=w87:errorcluster, "DIO Info Out"=w88:T19)  [unwired: 7 in]
    n26 = call "navX reading VI.vi"("NavX Info In"=w79, "Mode"=navX_type_def."Read Values", "error in (no error)"=w78) -> ("NavX Info Out"=w77:T24, "NavX Readings"=→"NavX Readings":T3, "Error Out"=w76:errorcluster)  [unwired: 1 out]
    n27 = call "FGV Stop.vi"("Init/Read/Write State"=States_for_Action_Engine."Read") -> ("Output node"=w111:bool)  [unwired: 2 in, 1 out]
    n28 = Wait (ms)(milliseconds to wait=u32 20) -> ()  [unwired: 1 out]
  }
  n29 = while {
    tunnel: w59 -> [w129]
    tunnel: w60 -> [w128]
    tunnel: [w127] -> w66
    tunnel: [w126] -> w65
    tunnel: w64 -> [w125]
    tunnel: [w124] -> w62
    tunnel: w63 -> [w123]
    tunnel: [w122] -> w61
    stop <- w120 stop-if-true
    # "Generate USER Event Loop"
    n30 = local read "Rising Edge"() -> (w117:bool)
    n31 = Or(x="OK Button", y=w117) -> (x .or. y?=w116:bool)
    n32 = local read "TASK ENABLE"() -> (w115:bool)
    n33 = And(x=w116, y=w115) -> (x .and. y?=w114:bool)
    n34 = case shown="True" w114 {
      selector: w114 -> [_ w140]
      tunnel: w129 -> [w139 w144]
      tunnel: [w139 w143] -> w126
      tunnel: w125 -> [w138 w142]
      tunnel: [w138 w141] -> w124
      frame False {
      }
      frame True {
        n35 = Generate User Event(user event=w144, event data cluster=w140, error in=w142) -> (user event out=w143:refnum<user-event>, error out=w141:errorcluster)  [unwired: 1 in]
      }
    }
    n36 = case shown="False" "STOP" {
      selector: "STOP" -> [_ w133]
      tunnel: w128 -> [w132 w137]
      tunnel: [w132 w136] -> w127
      tunnel: w123 -> [w131 w135]
      tunnel: [w131 w134] -> w122
      tunnel: [FALSE w133] -> w120
      frame False {
      }
      frame True {
        n37 = Generate User Event(user event=w137, event data cluster=w133, error in=w135) -> (user event out=w136:refnum<user-event>, error out=w134:errorcluster)  [unwired: 1 in]
      }
    }
    n38 = Wait (ms)(milliseconds to wait=u32 10) -> ()  [unwired: 1 out]
    n39 = call "FGV Stop.vi"("Init/Read/Write State"=States_for_Action_Engine."Write", "Input Node"=w120) -> ()  [unwired: 1 in, 2 out]
  }
  n40 = while {
    tunnel: w58 -> [w151]
    tunnel: [w150] -> w57
    tunnel: w45 -> [w148]
    tunnel: [w147] -> w56
    tunnel: w51 -> [w146]
    tunnel: [w145] -> w48
    stop <- w149 stop-if-true
    # "EVENT Handling Loop"
    n41 = event shown="[1] <Start Task>: User Event" {
      selector: w151 -> [_ _ _]
      dyn-events: [_ _ _] -> w150
      timeout: _ -> [_ _ _]
      tunnel: [FALSE FALSE w182] -> w149
      tunnel: w148 -> [w156 w165 w180]
      tunnel: [w155 w164 w181] -> w147
      tunnel: w146 -> [w154 w163 w179]
      tunnel: [w153 w162 w178] -> w145
      event Timeout {
        n42 = event-data() -> ()  [unwired: 1 in, 3 out]
        n43 = Enqueue Element(queue=w156, element=Intruction_Type_Definitions."None" ("Enum"), error in (no error)=w154) -> (queue out=w155:refnum<queue>, error out=w153:errorcluster)  [unwired: 1 in, 1 out]
      }
      event User Event {
        n44 = event-data() -> ()  [unwired: 1 in, 5 out]
        n45 = call "Arduino Interfacing VI.vi"("AE Mode"=Arduino_Interfacing."Read From Arduino") -> ("Arduino Data"=w159:T4)  [unwired: 3 in, 1 out]
        n46 = Unbundle By Name(w159) -> ("Rotary Switch"=w158:u8)
        n47 = case shown="10" w158 {
          tunnel: [Intruction_Type_Definitions."None" ("Enum") Intruction_Type_Definitions."Start Task 1" ("Enum") Intruction_Type_Definitions."Start Task 2" ("Enum") Intruction_Type_Definitions."Start Task 3" ("Enum") Intruction_Type_Definitions."Start Task 4" ("Enum") Intruction_Type_Definitions."Start Task 5" ("Enum") Intruction_Type_Definitions."Start Task 6" ("Enum") Intruction_Type_Definitions."Start Task 8" ("Enum") Intruction_Type_Definitions."Start Task 9" ("Enum") Intruction_Type_Definitions."Start Task A" ("Enum")] -> w161
          frame 0, Default {
          }
          frame 1 {
          }
          frame 2 {
          }
          frame 3 {
          }
          frame 4 {
          }
          frame 5 {
          }
          frame 6 {
          }
          frame 8 {
          }
          frame 9 {
          }
          frame 10 {
          }
        }
        n48 = Enqueue Element(queue=w165, element=w161, error in (no error)=w163) -> (queue out=w164:refnum<queue>, error out=w162:errorcluster)  [unwired: 1 in, 1 out]
      }
      event User Event {
        n49 = event-data() -> ("Stop Queue"=w182:bool)  [unwired: 1 in, 4 out]
        n50 = Enqueue Element At Opposite End(queue=w180, element=Intruction_Type_Definitions."Exit" ("Enum"), error in (no error)=w179) -> (queue out=w181:refnum<queue>, error out=w178:errorcluster)  [unwired: 1 in, 1 out]
      }
    }
  }
  n51 = while {
    tunnel: w45 -> [w220]
    tunnel: w46 -> [w232]
    tunnel: w49 -> [w230]
    tunnel: [w229] -> _
    tunnel: [w228] -> w39
    shift-right: [w221] -> _
    shift-left: T17 {"PING_A"=0, "PING_B"=0, "PING_C"=0, "PING_D"=0} -> [w223]
    shift-right: [w214] -> _
    shift-left: State_Type_Definitions,_for_0.26g_versions_and_later_2."Startup" ("Enum") -> [w217]
    shift-right: [w210] -> _
    shift-left: T18 {"xDistance"=0.0, "yDistance"=0.0, "wDistance"=0.0} -> [w212]
    shift-right: [w207] -> _
    shift-left: _ -> [w206]
    shift-right: [w203] -> _
    shift-left: T16 {"Recognized Object"=FALSE, "Object X coordinate"=0.0, "Object Y coordinate"=0.0} -> [w205]
    shift-right: [w200] -> _
    shift-left: T14 {"y Stepper Position"=0, "z Stepper Position"=0} -> [w202]
    shift-right: [w197] -> _
    shift-left: T13 {"Yaw"=0.0, "Compass"=0.0} -> [w199]
    shift-right: [w194] -> _
    shift-left: T12 {"Time up flag"=FALSE, "SET TIME TO CHECK"=0.0} -> [w196]
    shift-right: [w192] -> _
    shift-left: T11 {"yStepper desired"=0} -> [w193]
    shift-right: [w188] -> _
    shift-left: T10 {"Left IR Sensor"=0.0, "Arm IR Sensor"=0.0, "Bottom IR Sensor"=0.0} -> [w190]
    shift-right: [w186] -> _
    shift-left: T9 {"ySpeed"=0.0, "xSpeed"=0.0, "wSpeed"=0.0} -> [w187]
    shift-right: [w183] -> _
    shift-left: T8 {"Line Detected?"=FALSE, "S1"=0.0, "S2"=0.0, "S3"=0.0, "S4"=0.0} -> [w185]
    stop <- w219 stop-if-true
    # ">>> Motor control cluster >>>"
    # ">>> yStepper command>>>"
    # ">>True Stop Next State >>"
    # ">>Error  >>"
    # ">>Timeout>>"
    # ">>Action states Queue Reference >>"
    # ">>State Logic Queue Reference >>"
    # "TOP LEVEL BASELINE (MAIN PROCESSING LOOP)"
    n52 = Dequeue Element(queue=w232, timeout in ms (-1)=0, error in (no error)=w230) -> (queue out=w224:refnum<queue>, element=w231:string, error out=w225:errorcluster)  [unwired: 1 out]
    "Action State" <- w231
    n53 = Wait (ms)(milliseconds to wait=u32 20) -> ()  [unwired: 1 out]
    n54 = case shown="\"READ LINE SENSOR\"" w231 {
      tunnel: [_ _ _ _ _ _ _ _ _ _ _ _ _ _ _ _ _ _ _ _ 0 w2339 _ _ _ _ _ _ _ _ _ _ _ _ _ _ _ _ _ _ _ _ _ _ _ _ _ _ _ _ _] -> w227
      tunnel: w224 -> [_ _ _ _ _ _ _ _ _ _ _ _ _ _ _ _ _ _ _ _ _ _ _ _ _ _ _ _ _ _ _ _ _ _ _ _ _ _ _ _ _ _ _ _ _ _ _ _ _ _ _]
      tunnel: w223 -> [w2056 w2066 w2079 w2091 w2109 w2121 w2133 w2146 w2160 w2173 w2185 w2193 w2209 w2224 w2237 w2248 w2270 w2278 w2306 w2317 w2329 w2340 w2350 w2361 w2392 w2404 w2413 w2423 w2434 w2447 w2461 w2471 w2481 w2499 w2508 w2522 w2530 w2541 w2552 w2563 w2571 w2587 w2595 w2612 w2619 w2632 w2645 w2658 w2671 w2684 w2696]
      tunnel: [w2056 w2066 w2079 w2091 w2109 w2121 w2133 w2146 w2160 w2173 w2185 w2193 w2209 w2225 w2237 w2248 w2270 w2278 w2307 w2317 w2329 w2340 w2350 w2361 w2391 w2404 w2413 w2423 w2434 w2447 w2461 w2471 w2481 w2499 w2508 w2522 w2530 w2541 w2552 w2563 w2571 w2587 w2595 w2612 w2619 w2632 w2645 w2658 w2671 w2684 w2696] -> w222
      tunnel: [TRUE TRUE _ _ _ _ _ _ _ _ _ _ _ _ _ _ _ _ _ _ _ _ _ _ _ _ _ _ _ _ _ _ _ _ _ _ _ _ _ _ _ _ _ _ _ _ _ _ _ _ _] -> w219
      tunnel: w217 -> [w2054 w2064 w2078 w2090 w2108 w2120 w2132 w2145 w2159 w2172 w2184 w2192 w2208 w2223 w2236 w2246 w2263 w2277 w2305 w2316 w2326 w2337 w2349 w2360 w2390 w2403 w2412 w2422 w2426 w2446 w2460 w2470 w2480 w2498 w2507 w2516 w2529 w2540 w2551 w2562 w2570 w2578 w2594 w2611 w2618 w2631 w2644 w2657 w2670 w2683 w2695]
      tunnel: [_ _ _ _ _ _ _ _ _ _ _ _ _ _ _ _ _ _ _ _ _ TRUE _ _ _ _ _ _ _ _ _ _ _ _ _ _ _ _ _ _ _ _ _ _ _ _ _ _ _ _ _] -> w216
      tunnel: [w2054 w2064 w2078 w2090 w2108 w2120 w2132 w2145 w2159 w2172 w2184 w2192 w2208 w2223 w2236 w2246 w2263 w2277 w2305 w2316 w2326 w2337 w2349 w2360 w2390 w2403 w2412 w2422 w2426 w2446 w2460 w2470 w2480 w2498 w2507 w2516 w2529 w2540 w2551 w2562 w2570 w2578 w2594 w2611 w2618 w2631 w2644 w2657 w2670 w2683 w2695] -> w215
      tunnel: w212 -> [w2053 w2063 w2077 w2093 w2107 w2119 w2131 w2144 w2158 w2171 w2183 w2194 w2207 w2222 w2238 w2250 w2265 w2279 w2304 w2318 w2325 w2336 w2351 w2362 w2380 w2402 w2415 w2424 w2431 w2448 w2462 w2472 w2482 w2500 w2510 w2520 w2532 w2543 w2554 w2565 w2573 w2582 w2597 w2614 w2621 w2634 w2647 w2660 w2673 w2686 w2698]
      tunnel: [w2053 w2063 w2077 w2093 w2107 w2119 w2131 w2144 w2158 w2171 w2183 w2194 w2206 w2222 w2238 w2250 w2265 w2279 w2303 w2318 w2325 w2336 w2351 w2362 w2379 w2402 w2415 w2424 w2431 w2448 w2462 w2472 w2482 w2500 w2510 w2520 w2532 w2543 w2554 w2565 w2573 w2582 w2597 w2614 w2621 w2634 w2647 w2660 w2673 w2686 w2698] -> w211
      tunnel: w205 -> [w2052 w2062 w2076 w2092 w2106 w2118 w2130 w2143 w2157 w2170 w2181 w2191 w2205 w2221 w2231 w2249 w2264 w2276 w2295 w2315 w2324 w2335 w2348 w2359 w2385 w2400 w2414 w2421 w2432 w2445 w2459 w2466 w2479 w2493 w2509 w2521 w2531 w2542 w2553 w2564 w2572 w2581 w2596 w2613 w2620 w2633 w2646 w2659 w2672 w2685 w2697]
      tunnel: [w2052 w2062 w2076 w2092 w2106 w2118 w2130 w2143 w2157 w2170 w2181 w2191 w2205 w2221 w2231 w2249 w2264 w2276 w2294 w2315 w2324 w2335 w2348 w2359 w2384 w2400 w2414 w2421 w2432 w2445 w2459 w2466 w2479 w2492 w2509 w2521 w2531 w2542 w2553 w2564 w2572 w2581 w2596 w2613 w2620 w2633 w2646 w2659 w2672 w2685 w2697] -> w204
      tunnel: w202 -> [w2051 w2061 w2075 w2094 w2105 w2117 w2129 w2142 w2156 w2169 w2180 w2190 w2204 w2220 w2239 w2251 w2266 w2275 w2300 w2314 w2323 w2334 w2347 w2358 w2375 w2399 w2411 w2420 w2430 w2444 w2458 w2469 w2478 w2501 w2511 w2519 w2528 w2539 w2550 w2561 w2574 w2583 w2598 w2610 w2622 w2635 w2648 w2661 w2674 w2687 w2699]
      tunnel: [w2051 w2061 w2075 w2094 w2105 w2117 w2129 w2142 w2156 w2169 w2180 w2190 w2204 w2220 w2239 w2251 w2266 w2275 w2299 w2314 w2323 w2334 w2347 w2358 w2374 w2399 w2411 w2420 w2430 w2444 w2458 w2469 w2478 w2501 w2511 w2519 w2528 w2539 w2550 w2561 w2574 w2583 w2598 w2609 w2622 w2635 w2648 w2661 w2674 w2687 w2699] -> w201
      tunnel: w199 -> [w2050 w2060 w2073 w2095 w2103 w2115 w2128 w2140 w2154 w2167 w2179 w2189 w2203 w2213 w2234 w2252 w2267 w2274 w2290 w2313 w2322 w2333 w2346 w2357 w2371 w2398 w2408 w2419 w2429 w2443 w2457 w2468 w2477 w2502 w2512 w2518 w2527 w2536 w2547 w2558 w2575 w2584 w2599 w2604 w2623 w2636 w2649 w2662 w2675 w2688 w2700]
      tunnel: [w2050 w2060 w2073 w2095 w2103 w2115 w2128 w2140 w2154 w2167 w2179 w2189 w2203 w2213 w2233 w2252 w2267 w2274 w2289 w2313 w2322 w2333 w2346 w2357 w2370 w2398 w2408 w2419 w2429 w2443 w2457 w2468 w2477 w2502 w2512 w2518 w2527 w2536 w2547 w2558 w2575 w2584 w2599 w2604 w2623 w2636 w2649 w2662 w2675 w2688 w2700] -> w198
      tunnel: w196 -> [w2048 w2059 w2074 w2096 w2104 w2116 w2127 w2141 w2155 w2168 w2178 w2188 w2202 w2212 w2230 w2253 w2268 w2273 w2286 w2310 w2321 w2332 w2345 w2356 w2368 w2396 w2407 w2418 w2428 w2442 w2456 w2467 w2476 w2503 w2513 w2517 w2526 w2535 w2546 w2557 w2576 w2585 w2600 w2603 w2617 w2630 w2643 w2656 w2669 w2682 w2694]
      tunnel: [w2048 w2059 w2074 w2096 w2104 w2116 w2127 w2141 w2155 w2168 w2178 w2188 w2202 w2212 w2230 w2253 w2268 w2273 w2286 w2310 w2321 w2332 w2345 w2356 w2367 w2396 w2407 w2418 w2428 w2442 w2456 w2467 w2476 w2503 w2513 w2517 w2526 w2535 w2546 w2557 w2576 w2585 w2600 w2603 w2617 w2628 w2641 w2654 w2667 w2680 w2693] -> w195
      tunnel: w193 -> [_ _ _ _ _ _ _ _ _ _ _ _ _ _ _ _ _ _ _ _ _ _ _ _ _ _ _ _ _ _ _ _ _ _ _ _ _ _ _ _ _ _ w2591 _ _ _ _ _ _ _ _]
      tunnel: [w2047 w2058 w2068 w2086 w2098 w2111 w2123 w2135 w2150 w2162 w2175 w2187 w2196 w2211 w2227 w2244 w2269 w2272 w2283 w2309 w2320 w2331 w2344 w2353 w2364 w2395 w2406 w2417 w2433 w2436 w2450 w2464 w2474 w2486 w2505 w2523 w2525 w2534 w2545 w2556 w2567 w2586 w2589 w2602 w2616 w2625 w2638 w2651 w2664 w2677 w2690] -> w189
      tunnel: w190 -> [w2047 w2058 w2068 w2086 w2098 w2111 w2123 w2135 w2150 w2162 w2175 w2187 w2196 w2211 w2227 w2245 w2269 w2272 w2283 w2309 w2320 w2331 w2344 w2353 w2364 w2395 w2406 w2417 w2433 w2436 w2450 w2464 w2474 w2486 w2505 w2523 w2525 w2534 w2545 w2556 w2567 w2586 w2589 w2602 w2616 w2625 w2638 w2651 w2664 w2677 w2690]
      tunnel: w187 -> [_ _ _ _ _ _ _ _ w2149 _ _ _ _ _ _ _ _ _ _ _ _ _ _ _ _ _ _ _ _ _ _ _ _ _ _ _ _ _ _ _ _ _ _ _ _ _ _ _ _ _ _]
      tunnel: w185 -> [w2046 w2057 w2067 w2080 w2097 w2110 w2122 w2134 w2147 w2161 w2174 w2186 w2195 w2210 w2226 w2240 w2262 w2271 w2281 w2308 w2319 w2330 w2343 w2352 w2363 w2394 w2405 w2416 w2425 w2435 w2449 w2463 w2473 w2483 w2504 w2514 w2524 w2533 w2544 w2555 w2566 w2577 w2588 w2601 w2615 w2624 w2637 w2650 w2663 w2676 w2689]
      tunnel: [w2046 w2057 w2067 w2080 w2097 w2110 w2122 w2134 w2147 w2161 w2174 w2186 w2195 w2210 w2226 w2240 w2261 w2271 w2281 w2308 w2319 w2330 w2343 w2352 w2363 w2394 w2405 w2416 w2425 w2435 w2449 w2463 w2473 w2483 w2504 w2514 w2524 w2533 w2544 w2555 w2566 w2577 w2588 w2601 w2615 w2624 w2637 w2650 w2663 w2676 w2689] -> w184
      frame "Exit" {
        # ">>State Logic  >>"
        # ">>> Time cluster >>>"
        # ">>> Yaw >>>"
        # ">>> Stepper position >>>"
        # ">>> Encoders >>>"
        # ">>> Object detection >>>"
        # ">>> Ultrasonic Sensors Detect >>>"
        n55 = call "Imaq Dispose"("All Images? (No)"=TRUE) -> ()  [unwired: 5 in, 1 out]
      }
      frame "----Movement States----" {
        # ">>State Logic  >>"
        # ">>> Time cluster >>>"
        # ">>> Yaw >>>"
        # ">>> Stepper position >>>"
        # ">>> Encoders >>>"
        # ">>> Object detection >>>"
        # ">>> Ultrasonic Sensors Detect >>>"
      }
      frame "FORWARD" {
        # ">>State Logic  >>"
        # ">>> Time cluster >>>"
        # ">>> Yaw >>>"
        # ">>> Stepper position >>>"
        # ">>> Encoders >>>"
        # ">>> Object detection >>>"
        # ">>> Ultrasonic Sensors Detect >>>"
        n56 = Unbundle By Name(w2073) -> ("Yaw"=w2069:dbl)
        n57 = call "MOTOR CONTROL WITH PID AE.vi"("Yaw"=w2069, "Speed"=50.0, "Direction"=MOTOR_CONTROL_WITH_PID_AE_DIRECTION_TYPE_DEF."y-axis movement", "AE Mode"=MOTOR_CONTROL_WITH_PID_AE_DATA_MODE_TYPE_DEF."Write to AE") -> ()  [unwired: 1 out]
      }
      frame "FORWARD - IR ASSIST" {
        # ">>State Logic  >>"
        # ">>> Time cluster >>>"
        # ">>> Yaw >>>"
        # ">>> Stepper position >>>"
        # ">>> Encoders >>>"
        # ">>> Object detection >>>"
        # ">>> Ultrasonic Sensors Detect >>>"
        n58 = Unbundle By Name(w2086) -> ("Left IR Sensor"=w2085:dbl)
        n59 = Subtract(x=w2085, y=15.0) -> (x-y=w2083:dbl)
        n60 = Multiply(x=w2083, y=0.5) -> (x*y=w2081:dbl)
        n61 = call "MOTOR CONTROL WITH PID AE.vi"("Yaw"=w2081, "Speed"=30.0, "Direction"=MOTOR_CONTROL_WITH_PID_AE_DIRECTION_TYPE_DEF."y-axis movement", "AE Mode"=MOTOR_CONTROL_WITH_PID_AE_DATA_MODE_TYPE_DEF."Write to AE") -> ()  [unwired: 1 out]
      }
      frame "LEFT" {
        # ">>State Logic  >>"
        # ">>> Time cluster >>>"
        # ">>> Yaw >>>"
        # ">>> Stepper position >>>"
        # ">>> Encoders >>>"
        # ">>> Object detection >>>"
        # ">>> Ultrasonic Sensors Detect >>>"
        n62 = Unbundle By Name(w2103) -> ("Yaw"=w2100:dbl)
        n63 = call "MOTOR CONTROL WITH PID AE.vi"("Yaw"=w2100, "Speed"=-25.0, "Direction"=MOTOR_CONTROL_WITH_PID_AE_DIRECTION_TYPE_DEF."x-axis movement", "AE Mode"=MOTOR_CONTROL_WITH_PID_AE_DATA_MODE_TYPE_DEF."Write to AE") -> ()  [unwired: 1 out]
      }
      frame "R-ACW" {
        # ">>> IR Sensors >>>"
        # ">>> Time cluster >>>"
        # ">>> Yaw >>>"
        # ">>> Stepper position >>>"
        # ">>> Encoders >>>"
        # ">>> Object detection >>>"
        # ">>> Ultrasonic Sensors Detect >>>"
        n64 = call "MOTOR CONTROL WITH PID AE.vi"("Speed"=-10.0, "Direction"=MOTOR_CONTROL_WITH_PID_AE_DIRECTION_TYPE_DEF."rotation", "AE Mode"=MOTOR_CONTROL_WITH_PID_AE_DATA_MODE_TYPE_DEF."Write to AE") -> ()  [unwired: 1 in, 1 out]
      }
      frame "R-CW" {
        (unwired) -0.2 ("Speed")
        # ">>> Time cluster >>>"
        # ">>> Yaw >>>"
        # ">>> Stepper position >>>"
        # ">>> Encoders >>>"
        # ">>> Object detection >>>"
        # ">>> Ultrasonic Sensors Detect >>>"
        n65 = call "MOTOR CONTROL WITH PID AE.vi"("Speed"=10.0, "Direction"=MOTOR_CONTROL_WITH_PID_AE_DIRECTION_TYPE_DEF."rotation", "AE Mode"=MOTOR_CONTROL_WITH_PID_AE_DATA_MODE_TYPE_DEF."Write to AE") -> ()  [unwired: 1 in, 1 out]
      }
      frame "RIGHT" {
        # ">>> Time cluster >>>"
        # ">>> Yaw >>>"
        # ">>> Stepper position >>>"
        # ">>> Encoders >>>"
        # ">>> Object detection >>>"
        # ">>> Ultrasonic Sensors Detect >>>"
        n66 = Unbundle By Name(w2140) -> ("Yaw"=w2136:dbl)
        n67 = call "MOTOR CONTROL WITH PID AE.vi"("Yaw"=w2136, "Speed"=50.0, "Direction"=MOTOR_CONTROL_WITH_PID_AE_DIRECTION_TYPE_DEF."x-axis movement", "AE Mode"=MOTOR_CONTROL_WITH_PID_AE_DATA_MODE_TYPE_DEF."Write to AE") -> ()  [unwired: 1 out]
      }
      frame "X AXIS - SLOW" {
        # ">>> IR Sensors >>>"
        # ">>> Time cluster >>>"
        # ">>> Yaw >>>"
        # ">>> Stepper position >>>"
        # ">>> Encoders >>>"
        # ">>> Object detection >>>"
        # ">>> Ultrasonic Sensors Detect >>>"
        n68 = Unbundle By Name(w2149) -> ("xSpeed"=w2148:dbl)
        n69 = Unbundle By Name(w2154) -> ("Yaw"=w2151:dbl)
        n70 = call "MOTOR CONTROL WITH PID AE.vi"("Yaw"=w2151, "Speed"=w2148, "Direction"=MOTOR_CONTROL_WITH_PID_AE_DIRECTION_TYPE_DEF."x-axis movement", "AE Mode"=MOTOR_CONTROL_WITH_PID_AE_DATA_MODE_TYPE_DEF."Write to AE") -> ()  [unwired: 1 out]
      }
      frame "REVERSE" {
        # ">>> Time cluster >>>"
        # ">>> Yaw >>>"
        # ">>> Stepper position >>>"
        # ">>> Encoders >>>"
        # ">>> Object detection >>>"
        # ">>> Ultrasonic Sensors Detect >>>"
        n71 = Unbundle By Name(w2167) -> ("Yaw"=w2163:dbl)
        n72 = call "MOTOR CONTROL WITH PID AE.vi"("Yaw"=w2163, "Speed"=-50.0, "Direction"=MOTOR_CONTROL_WITH_PID_AE_DIRECTION_TYPE_DEF."y-axis movement", "AE Mode"=MOTOR_CONTROL_WITH_PID_AE_DATA_MODE_TYPE_DEF."Write to AE") -> ()  [unwired: 1 out]
      }
      frame "STOP" {
        n73 = Wait (ms)(milliseconds to wait=u32 100) -> ()  [unwired: 1 out]
        n74 = call "MOTOR CONTROL WITH PID AE.vi"("Direction"=MOTOR_CONTROL_WITH_PID_AE_DIRECTION_TYPE_DEF."stop", "AE Mode"=MOTOR_CONTROL_WITH_PID_AE_DATA_MODE_TYPE_DEF."Write to AE") -> ()  [unwired: 2 in, 1 out]
      }
      frame "----SENSOR READING---- " {
      }
      frame "READ ENCODERS" {
        # ">>> Time cluster >>>"
        # ">>> Yaw >>>"
        # ">>> Stepper position >>>"
        # ">>> Object detection >>>"
        # ">>> Current encoder distance >>>"
        # ">>> Ultrasonic Sensors Detect >>>"
        n75 = call "MOTOR CONTROL WITH PID AE.vi"("AE Mode"=MOTOR_CONTROL_WITH_PID_AE_DATA_MODE_TYPE_DEF."Read from AE") -> ("Speed & distance"=w2200:T1)  [unwired: 3 in]
        n76 = Unbundle By Name(w2200) -> ("xDistance"=w2199:dbl, "yDistance"=w2198:dbl, "wDistance"=w2197:dbl)
        n77 = Bundle By Name(cluster=w2207, "xDistance"=w2199, "yDistance"=w2198, "wDistance"=w2197) -> (w2206:T18)
      }
      frame "READ ULTRASONIC" {
        (unwired) navX_type_def."Read Values" ("Mode")
        (unwired) MOTOR_CONTROL_NO_PID_Type_Def."Latch" ("Direction")
        # ">>State Logic  >>"
        # ">>> Time cluster >>>"
        # ">>> Ultrasonic Sensors Detect >>>"
        # ">>> Object detection >>>"
        # ">>> Encoders >>>"
        # ">>> Stepper position >>>"
        # ">>> Yaw >>>"
        n78 = call "Arduino Interfacing VI.vi"("AE Mode"=Arduino_Interfacing."Read From Arduino") -> ("Arduino Data"=w2218:T4)  [unwired: 3 in, 1 out]
        n79 = Unbundle By Name(w2218) -> ("PING A"=w2217:u8, "PING B"=w2216:u8, "PING C"=w2215:u8, "PING D"=w2214:u8)
        n80 = Bundle By Name(cluster=w2224, "PING_A"=w2217, "PING_B"=w2216, "PING_C"=w2215, "PING_D"=w2214) -> (w2225:T17)
      }
      frame "READ NAVX" {
        # ">>> Time cluster >>>"
        # ">>> Yaw >>>"
        # ">>> Ultrasonic Sensors Detect >>>"
        # ">>> Object detection >>>"
        # ">>> Encoders >>>"
        # ">>> Stepper position >>>"
        n81 = call "navX reading VI.vi"("Mode"=navX_type_def."Read Values") -> ("NavX Readings"=w2229:T3)  [unwired: 2 in, 3 out]
        n82 = Unbundle By Name(w2229) -> ("Heading"=w2228:dbl)
        n83 = Unbundle By Name(w2229) -> ("Yaw"=w2232:dbl)
        n84 = Bundle By Name(cluster=w2234, "Yaw"=w2232, "Compass"=w2228) -> (w2233:T13)
      }
      frame "READ IR" {
        w2242 = T38 [enum."B/AI1"] items=["Not Connected", "AudioIn/Left", "AudioIn/Right", "C/AI0", "C/AI1", "A/AI0", "A/AI1", "A/AI2", "A/AI3", "A/AI4", "A/AI5", "A/AI6", "A/AI7", "B/AI0", "B/AI1", "B/AI2", "B/AI3", "B/AI4", "B/AI5", "B/AI6", "B/AI7", "AI/AI0", "AI/AI1", "AI/AI2", "AI/AI3", "A/AI0 (DIFF)", "A/AI1 (DIFF)", "A/AI2 (DIFF)", "A/AI3 (DIFF)", "B/AI0 (DIFF)", "B/AI1 (DIFF)", "B/AI2 (DIFF)", "B/AI3 (DIFF)"] ("AI Channel")
        w2247 = T38 [enum."B/AI0"] items=["Not Connected", "AudioIn/Left", "AudioIn/Right", "C/AI0", "C/AI1", "A/AI0", "A/AI1", "A/AI2", "A/AI3", "A/AI4", "A/AI5", "A/AI6", "A/AI7", "B/AI0", "B/AI1", "B/AI2", "B/AI3", "B/AI4", "B/AI5", "B/AI6", "B/AI7", "AI/AI0", "AI/AI1", "AI/AI2", "AI/AI3", "A/AI0 (DIFF)", "A/AI1 (DIFF)", "A/AI2 (DIFF)", "A/AI3 (DIFF)", "B/AI0 (DIFF)", "B/AI1 (DIFF)", "B/AI2 (DIFF)", "B/AI3 (DIFF)"] ("AI Channel")
        # ">>State Logic  >>"
        # ">>> Time cluster >>>"
        # ">>> Ultrasonic Sensors Detect >>>"
        # ">>> Object detection >>>"
        # ">>> Encoders >>>"
        # ">>> Stepper position >>>"
        # ">>> Yaw >>>"
        n85 = call <vilib>:"Sharp IR.vi"("AI Channel"=w2247) -> ("Sharp IR Distance"=w2243:dbl)  [unwired: 8 in, 2 out]
        n86 = call <vilib>:"Sharp IR.vi"("AI Channel"=w2242) -> ("Sharp IR Distance"=w2241:dbl)  [unwired: 8 in, 2 out]
        n87 = Bundle By Name(cluster=w2245, "Left IR Sensor"=w2243, "Arm IR Sensor"=w2241) -> (w2244:T10)
      }
      frame "READ LINE SENSOR" {
        # ">>> IR Sensors >>>"
        # ">>> Line Sensor Cluster>>>"
        # ">>State Logic  >>"
        # ">>> Time cluster >>>"
        # ">>> Object detection >>>"
        # ">>> Yaw >>>"
        # ">>> Ultrasonic Sensors Detect >>>"
        # ">>> Encoders >>>"
        # ">>> Stepper position >>>"
        n88 = call "Line Sensor AE.vi"("AE State"=Line_Sensor_AE_Type_Def."READ FROM LINE SENSORS") -> ("Line Detected?"=w2259:bool, "Line Sensor Raw Values"=w2258:T40)
        n89 = Unbundle By Name(w2258) -> ("S1"=w2257:dbl, "S2"=w2256:dbl, "S3"=w2255:dbl, "S4"=w2254:dbl)
        n90 = Bundle By Name(cluster=w2262, "Line Detected?"=w2259, "S1"=w2257, "S2"=w2256, "S3"=w2255, "S4"=w2254) -> (w2261:T8)
      }
      frame "----SYSTEM MODES----" {
        (unwired) I2C_MASTER_Type_Def."Last State" ("Arduino Mode")
        # ">>> Object detection >>>"
        # ">>> Yaw >>>"
        # ">>> Ultrasonic Sensors Detect >>>"
        # ">>> Encoders >>>"
        # ">>> Stepper position >>>"
      }
      frame "INIT" {
        w2301 = u8 0
        w2302 = 0.0
        # ">>> IR Sensors >>>"
        # ">>> IR Sensors >>>"
        # ">>> Line Sensor Cluster>>>"
        # ">>> Time cluster >>>"
        # ">>> Object detection >>>"
        # ">>> Yaw >>>"
        # ">>> Ultrasonic Sensors Detect >>>"
        # ">>> Encoders >>>"
        # ">>> Stepper position >>>"
        # ">>State Logic  >>"
        n91 = call "Arduino Interfacing VI.vi"("AE Mode"=Arduino_Interfacing."Initialize") -> ()  [unwired: 3 in, 2 out]
        n92 = call "FGV Stop.vi"("Init/Read/Write State"=States_for_Action_Engine."Initialize") -> ()  [unwired: 2 in, 2 out]
        n93 = call "Elasped Timer.vi"("Action"=Elapsed_timer_control."Initialize") -> ()  [unwired: 7 in, 4 out]
        n94 = call "MOTOR CONTROL WITH PID AE.vi"("AE Mode"=MOTOR_CONTROL_WITH_PID_AE_DATA_MODE_TYPE_DEF."Init AE") -> ()  [unwired: 3 in, 1 out]
        n95 = call "IMAQ Reference AE.vi"("IMAQ AE States"=IMAQ_Reference_AE."Initialize AE") -> ()  [unwired: 1 in, 2 out]
        n96 = call "Line Sensor AE.vi"("AE State"=Line_Sensor_AE_Type_Def."INIT AE") -> ()  [unwired: 2 out]
        n97 = Bundle By Name(cluster=w2295, "Recognized Object"=FALSE, "Object X coordinate"=0.0, "Object Y coordinate"=0.0) -> (w2294:T16)
        n98 = Bundle By Name(cluster=w2300, "y Stepper Position"=u8 0, "z Stepper Position"=u8 0) -> (w2299:T14)
        n99 = Bundle By Name(cluster=w2304, "xDistance"=w2302, "yDistance"=w2302, "wDistance"=w2302) -> (w2303:T18)
        n100 = Bundle By Name(cluster=w2306, "PING_A"=w2301, "PING_B"=w2301, "PING_C"=w2301, "PING_D"=w2301) -> (w2307:T17)
        n101 = Bundle By Name(cluster=w2290, "Yaw"=0.0) -> (w2289:T13)
      }
      frame "ARDUINO - ULTRASONIC" {
        # ">>> Time cluster >>>"
        # ">>> Line Sensor Cluster>>>"
        # ">>> Object detection >>>"
        # ">>> Yaw >>>"
        # ">>> Ultrasonic Sensors Detect >>>"
        # ">>> Encoders >>>"
        # ">>> Stepper position >>>"
        # ">>State Logic  >>"
        n102 = call "Arduino Interfacing VI.vi"("Data to Write"=I2C_MASTER_WRITE_NEW_Type_Def."Ultrasonic sensors", "AE Mode"=Arduino_Interfacing."Write to Arduino") -> ()  [unwired: 2 in, 2 out]
      }
      frame "NAVX CALIBRATE" {
        # ">>> Object detection >>>"
        # ">>> Yaw >>>"
        # ">>> Ultrasonic Sensors Detect >>>"
        # ">>> Encoders >>>"
        # ">>> Stepper position >>>"
        # ">>State Logic  >>"
        # "Adds a 15 second delay to the startup process \nfor the NavX to calibrate"
        n103 = Wait (ms)(milliseconds to wait=u32 1000) -> ()  [unwired: 1 out]
      }
      frame "NO ACTION", Default {
        (unwired) u8 0 ("y Stepper value")
        (unwired) TRUE ("Latch")
        (unwired) navX_type_def."Read Values" ("Mode")
        (unwired) MOTOR_CONTROL_NO_PID_Type_Def."Latch" ("Direction")
        # ">>> Object detection >>>"
        # ">>> Yaw >>>"
        # ">>> Ultrasonic Sensors Detect >>>"
        # ">>> Encoders >>>"
        # ">>> Stepper position >>>"
        # ">>State Logic  >>"
        n104 = case shown="4" w2337 {
          tunnel: [0 100] -> w2339
          frame 1, Default {
          }
          frame 4 {
          }
        }
      }
      frame "----RESET CASES----" {
        (unwired) I2C_MASTER_Type_Def."Last State" ("Arduino Mode")
        # ">>> Object detection >>>"
        # ">>> Yaw >>>"
        # ">>> Ultrasonic Sensors Detect >>>"
        # ">>> Encoders >>>"
        # ">>> Stepper position >>>"
        # ">>State Logic  >>"
      }
      frame "RESET ENCODERS" {
        # ">>> Object detection >>>"
        # ">>> Yaw >>>"
        # ">>> Ultrasonic Sensors Detect >>>"
        # ">>> Encoders >>>"
        # ">>> Stepper position >>>"
        # ">>State Logic  >>"
        n105 = call "MOTOR CONTROL WITH PID AE.vi"("Direction"=MOTOR_CONTROL_WITH_PID_AE_DIRECTION_TYPE_DEF."reset encoders", "AE Mode"=MOTOR_CONTROL_WITH_PID_AE_DATA_MODE_TYPE_DEF."Write to AE") -> ()  [unwired: 2 in, 1 out]
      }
      frame "RESET FLAGS" {
        (unwired) I2C_MASTER_Type_Def."Last State" ("Arduino Mode")
        # "Resets any software variables\nand/or non-critical states"
        n106 = Wait (ms)(milliseconds to wait=u32 20) -> ()  [unwired: 1 out]
        n107 = Bundle By Name(cluster=w2368, "Time up flag"=FALSE, "SET TIME TO CHECK"=0.0) -> (w2367:T12)
        n108 = Bundle By Name(cluster=w2385, "Recognized Object"=FALSE, "Object X coordinate"=0.0, "Object Y coordinate"=0.0) -> (w2384:T16)
        n109 = Bundle By Name(cluster=w2375, "y Stepper Position"=u8 0, "z Stepper Position"=u8 0) -> (w2374:T14)
        n110 = Bundle By Name(cluster=w2380, "xDistance"=0.0, "yDistance"=0.0, "wDistance"=0.0) -> (w2379:T18)
        n111 = Bundle By Name(cluster=w2392, "PING_A"=u8 0, "PING_B"=u8 0, "PING_C"=u8 0, "PING_D"=u8 0) -> (w2391:T17)
        n112 = Bundle By Name(cluster=w2371, "Yaw"=0.0) -> (w2370:T13)
      }
      frame "RESET YAW" {
        n113 = Wait (ms)(milliseconds to wait=u32 100) -> ()  [unwired: 1 out]
        n114 = call "navX reading VI.vi"("Mode"=navX_type_def."Zero Yaw") -> ()  [unwired: 2 in, 4 out]
      }
      frame "RESET ARM" {
        n115 = call "Arduino Interfacing VI.vi"("Data to Write"=I2C_MASTER_WRITE_NEW_Type_Def."Soft Reset", "AE Mode"=Arduino_Interfacing."Write to Arduino") -> ()  [unwired: 2 in, 2 out]
      }
      frame "--------CAM STATES-------" {
      }
      frame "OPEN IMAQ REF" {
        # ">>State Logic  >>"
        # ">>> Time cluster >>>"
        # ">>> Object detection >>>"
        # ">>> Yaw >>>"
        # ">>> Ultrasonic Sensors Detect >>>"
        # ">>> Encoders >>>"
        # ">>> Stepper position >>>"
        # ">>> IR Sensors >>>"
        n116 = call "IMAQ Reference AE.vi"("IMAQ AE States"=IMAQ_Reference_AE."Initialize AE") -> ()  [unwired: 1 in, 2 out]
      }
      frame "OPEN LOG CAM" {
        n117 = call "Webcam AE.vi"("Session In"=T34 "cam0", "Camera states"=Webcam_AE."Initialize Camera") -> ("error out"=w2439:errorcluster, "Session Out"=w2438:T34)  [unwired: 1 in, 1 out]
        n118 = call "Webcam AE.vi"("error in (no error)"=w2439, "Session In"=w2438, "Camera states"=Webcam_AE."Open Camera") -> ()  [unwired: 3 out]
      }
      frame "OPEN LIFE CAM" {
        n119 = call "Webcam AE.vi"("Session In"=T34 "cam1", "Camera states"=Webcam_AE."Initialize Camera") -> ("error out"=w2453:errorcluster, "Session Out"=w2452:T34)  [unwired: 1 in, 1 out]
        n120 = call "Webcam AE.vi"("error in (no error)"=w2453, "Session In"=w2452, "Camera states"=Webcam_AE."Open Camera") -> ()  [unwired: 3 out]
      }
      frame "CAM ACQ" {
        # ">>State Logic  >>"
        # ">>> Time cluster >>>"
        # ">>> Yaw >>>"
        # ">>> Stepper position >>>"
        # ">>> Encoders >>>"
        # ">>> Object detection >>>"
        # ">>> Ultrasonic Sensors Detect >>>"
        n121 = call "Webcam AE.vi"("Camera states"=Webcam_AE."Continuous Acquisition") -> ()  [unwired: 2 in, 3 out]
      }
      frame "CAM CLOSE" {
        # ">>State Logic  >>"
        # ">>> Time cluster >>>"
        # ">>> Yaw >>>"
        # ">>> Stepper position >>>"
        # ">>> Encoders >>>"
        # ">>> Object detection >>>"
        # ">>> Ultrasonic Sensors Detect >>>"
        n122 = call "Webcam AE.vi"("Camera states"=Webcam_AE."Close Camera") -> ()  [unwired: 2 in, 3 out]
      }
      frame "PROCESS IMAGE" {
        # ">>State Logic  >>"
        # ">>> Time cluster >>>"
        # ">>> Yaw >>>"
        # ">>> Stepper position >>>"
        # ">>> Encoders >>>"
        # ">>> Object detection >>>"
        # ">>> Ultrasonic Sensors Detect >>>"
        n123 = call "Webcam AE.vi"("Camera states"=Webcam_AE."Retrieve Image") -> ("error out"=w2494:errorcluster, "Image Out"=w2496:T42)  [unwired: 2 in, 1 out]
        n124 = call "IMAQ Reference AE.vi"("IMAQ AE States"=IMAQ_Reference_AE."Get IMAQ Reference") -> ("Image Out"=w2484:T42)  [unwired: 1 in, 1 out]
        n125 = call "Object Detection SubVI.vi"("Error In"=w2494, "Mode"="Object recognition mode", "Image Dest"=w2484, "Image in"=w2496) -> ("Object Center Coordinates"=w2491:cluster{"x":sgl, "y":sgl}, "Object detection cluster"=w2487:T2)  [unwired: 2 out]
        "Object detection cluster" <- w2487
        "Object Center Coordinates" <- w2491
        n126 = Unbundle By Name(w2487) -> ("Object detected?"=w2488:bool)
        n127 = Unbundle By Name(w2491) -> ("x"=w2490:sgl, "y"=w2489:sgl)
        n128 = Bundle By Name(cluster=w2493, "Recognized Object"=w2488, "Object X coordinate"=w2490, "Object Y coordinate"=w2489) -> (w2492:T16)
      }
      frame "DISPOSE BUFFERS" {
        # ">>> Line Sensor Cluster>>>"
        # ">>> IR Sensors >>>"
        # ">>State Logic  >>"
        # ">>> Time cluster >>>"
        # ">>> Yaw >>>"
        # ">>> Stepper position >>>"
        # ">>> Encoders >>>"
        # ">>> Object detection >>>"
        # ">>> Ultrasonic Sensors Detect >>>"
        n129 = call "Webcam AE.vi"("Camera states"=Webcam_AE."Dispose Image Buffers") -> ()  [unwired: 2 in, 3 out]
      }
      frame "DISPOSE ALL BUFFERS" {
        # ">>State Logic  >>"
        # ">>> IR Sensors >>>"
        # ">>> Time cluster >>>"
        # ">>> Object detection >>>"
        # ">>> Yaw >>>"
        # ">>> Ultrasonic Sensors Detect >>>"
        # ">>> Encoders >>>"
        # ">>> Stepper position >>>"
        n130 = call "IMAQ Reference AE.vi"("IMAQ AE States"=IMAQ_Reference_AE."Destroy ALL IMAQ") -> ()  [unwired: 1 in, 2 out]
      }
      frame "-----ARM ACTIONS-----" {
      }
      frame "CLOSE CLAW" {
        n131 = call "Arduino Interfacing VI.vi"("Data to Write"=I2C_MASTER_WRITE_NEW_Type_Def."Close Claw", "AE Mode"=Arduino_Interfacing."Write to Arduino") -> ()  [unwired: 2 in, 2 out]
      }
      frame "OPEN CLAW" {
        n132 = call "Arduino Interfacing VI.vi"("Data to Write"=I2C_MASTER_WRITE_NEW_Type_Def."Open Claw", "AE Mode"=Arduino_Interfacing."Write to Arduino") -> ()  [unwired: 2 in, 2 out]
      }
      frame "Z STEPPER CAM HEIGHT" {
        n133 = call "Arduino Interfacing VI.vi"("Data to Write"=I2C_MASTER_WRITE_NEW_Type_Def."zStepper 6k", "AE Mode"=Arduino_Interfacing."Write to Arduino") -> ()  [unwired: 2 in, 2 out]
      }
      frame "Z STEPPER GRAB HEIGHT" {
        # ">>State Logic  >>"
        # ">>> Time cluster >>>"
        # ">>> Yaw >>>"
        # ">>> Stepper position >>>"
        # ">>> Encoders >>>"
        # ">>> Object detection >>>"
        # ">>> Ultrasonic Sensors Detect >>>"
        n134 = call "Arduino Interfacing VI.vi"("Data to Write"=I2C_MASTER_WRITE_NEW_Type_Def."zStepper 100", "AE Mode"=Arduino_Interfacing."Write to Arduino") -> ()  [unwired: 2 in, 2 out]
      }
      frame "Z STEPPER BOX HEIGHT" {
        # ">>> IR Sensors >>>"
        # ">>> Time cluster >>>"
        # ">>> Yaw >>>"
        # ">>> Stepper position >>>"
        # ">>> Encoders >>>"
        # ">>> Object detection >>>"
        # ">>> Ultrasonic Sensors Detect >>>"
        n135 = call "Arduino Interfacing VI.vi"("Data to Write"=I2C_MASTER_WRITE_NEW_Type_Def."zStepper 4k", "AE Mode"=Arduino_Interfacing."Write to Arduino") -> ()  [unwired: 2 in, 2 out]
      }
      frame "Y STEPPER CONTROL" {
        # ">>State Logic  >>"
        # ">>> yStepper command>>>"
        # ">>> Time cluster >>>"
        # ">>> Yaw >>>"
        # ">>> Stepper position >>>"
        # ">>> Encoders >>>"
        # ">>> Object detection >>>"
        # ">>> Ultrasonic Sensors Detect >>>"
        n136 = Unbundle By Name(w2591) -> ("yStepper desired"=w2590:u8)
        n137 = call "Arduino Interfacing VI.vi"("y Stepper value"=w2590, "Data to Write"=I2C_MASTER_WRITE_NEW_Type_Def."yStepper control", "AE Mode"=Arduino_Interfacing."Write to Arduino") -> ()  [unwired: 1 in, 2 out]
      }
      frame "READ STEPPER VALUES" {
        # ">>State Logic  >>"
        # ">>> Time cluster >>>"
        # ">>> Yaw >>>"
        # ">>> Stepper position >>>"
        # ">>> Encoders >>>"
        # ">>> Object detection >>>"
        # ">>> Ultrasonic Sensors Detect >>>"
        n138 = call "Arduino Interfacing VI.vi"("AE Mode"=Arduino_Interfacing."Read From Arduino") -> ("Arduino Data"=w2607:T4)  [unwired: 3 in, 1 out]
        n139 = Unbundle By Name(w2607) -> ("y Stepper Position"=w2606:u8, "z Stepper Position"=w2605:u8)
        n140 = Bundle By Name(cluster=w2610, "y Stepper Position"=w2606, "z Stepper Position"=w2605) -> (w2609:T14)
      }
      frame " -----TIMING-----" {
        # ">>State Logic  >>"
        # ">>> Time cluster >>>"
        # ">>> Yaw >>>"
        # ">>> Stepper position >>>"
        # ">>> Encoders >>>"
        # ">>> Object detection >>>"
        # ">>> Ultrasonic Sensors Detect >>>"
      }
      frame "SET TIMER 1" {
        # ">>State Logic  >>"
        # ">>> Time cluster >>>"
        # ">>> Yaw >>>"
        # ">>> Stepper position >>>"
        # ">>> Encoders >>>"
        # ">>> Object detection >>>"
        # ">>> Ultrasonic Sensors Detect >>>"
        n141 = call "Elasped Timer.vi"("Time Setting"=1.0, "Action"=Elapsed_timer_control."Initialize") -> ()  [unwired: 6 in, 4 out]
        n142 = Bundle By Name(cluster=w2630, "Time up flag"=FALSE) -> (w2628:T12)
      }
      frame "SET TIMER 2" {
        # ">>State Logic  >>"
        # ">>> Time cluster >>>"
        # ">>> Yaw >>>"
        # ">>> Stepper position >>>"
        # ">>> Encoders >>>"
        # ">>> Object detection >>>"
        # ">>> Ultrasonic Sensors Detect >>>"
        n143 = call "Elasped Timer.vi"("Time Setting"=2.0, "Action"=Elapsed_timer_control."Initialize") -> ()  [unwired: 6 in, 4 out]
        n144 = Bundle By Name(cluster=w2643, "Time up flag"=FALSE) -> (w2641:T12)
      }
      frame "SET TIMER 3" {
        # ">>State Logic  >>"
        # ">>> Time cluster >>>"
        # ">>> Yaw >>>"
        # ">>> Stepper position >>>"
        # ">>> Encoders >>>"
        # ">>> Object detection >>>"
        # ">>> Ultrasonic Sensors Detect >>>"
        n145 = call "Elasped Timer.vi"("Time Setting"=3.0, "Action"=Elapsed_timer_control."Initialize") -> ()  [unwired: 6 in, 4 out]
        n146 = Bundle By Name(cluster=w2656, "Time up flag"=FALSE) -> (w2654:T12)
      }
      frame "SET TIMER 4" {
        # ">>State Logic  >>"
        # ">>> Time cluster >>>"
        # ">>> Yaw >>>"
        # ">>> Stepper position >>>"
        # ">>> Encoders >>>"
        # ">>> Object detection >>>"
        # ">>> Ultrasonic Sensors Detect >>>"
        n147 = call "Elasped Timer.vi"("Time Setting"=4.0, "Action"=Elapsed_timer_control."Initialize") -> ()  [unwired: 6 in, 4 out]
        n148 = Bundle By Name(cluster=w2669, "Time up flag"=FALSE) -> (w2667:T12)
      }
      frame "SET TIMER 5" {
        # ">>State Logic  >>"
        # ">>> Time cluster >>>"
        # ">>> Yaw >>>"
        # ">>> Stepper position >>>"
        # ">>> Encoders >>>"
        # ">>> Object detection >>>"
        # ">>> Ultrasonic Sensors Detect >>>"
        n149 = call "Elasped Timer.vi"("Time Setting"=5.0, "Action"=Elapsed_timer_control."Initialize") -> ()  [unwired: 6 in, 4 out]
        n150 = Bundle By Name(cluster=w2682, "Time up flag"=FALSE) -> (w2680:T12)
      }
      frame "START TIMER" {
        # ">>State Logic  >>"
        # ">>> Time cluster >>>"
        # ">>> Yaw >>>"
        # ">>> Stepper position >>>"
        # ">>> Encoders >>>"
        # ">>> Object detection >>>"
        # ">>> Ultrasonic Sensors Detect >>>"
        n151 = call "Elasped Timer.vi"("Action"=Elapsed_timer_control."Start") -> ("Time Out?!"=w2691:bool)  [unwired: 7 in, 3 out]
        n152 = Bundle By Name(cluster=w2694, "Time up flag"=w2691) -> (w2693:T12)
      }
    }
    "State Logic" <- w215
    n153 = local read "TASK ENABLE"() -> (w209:bool)
    n154 = Not(x=w209) -> (.not. x?=w208:bool)
    n155 = case shown="True" w216 {
      tunnel: w220 -> [w246 w284]
      tunnel: w224 -> [w242 w286]
      tunnel: [w246 w284] -> w229
      tunnel: [w242 w287] -> w228
      tunnel: w225 -> [_ w282]
      tunnel: w227 -> [_ w283]
      tunnel: w222 -> [w245 w289]
      tunnel: [w245 w289] -> w221
      tunnel: "STOP TASK" -> [_ w272]
      tunnel: w215 -> [w244 w288]
      tunnel: [w244 w285] -> w214
      tunnel: w211 -> [w243 w278]
      tunnel: [w243 w278] -> w210
      tunnel: w208 -> [_ w273]
      tunnel: [w241 w270] -> w207
      tunnel: w206 -> [w241 w269]
      tunnel: w204 -> [w240 w266]
      tunnel: [w240 w266] -> w203
      tunnel: w201 -> [w239 w262]
      tunnel: [w239 w262] -> w200
      tunnel: w198 -> [w238 w260]
      tunnel: [w238 w260] -> w197
      tunnel: w195 -> [w237 w258]
      tunnel: [w237 w258] -> w194
      tunnel: w193 -> [w236 w257]
      tunnel: [w236 w256] -> w192
      tunnel: [_ w254] -> w191
      tunnel: w189 -> [w235 w252]
      tunnel: [w235 w252] -> w188
      tunnel: w187 -> [w234 w251]
      tunnel: [w234 w250] -> w186
      tunnel: w184 -> [w233 w247]
      tunnel: [w233 w247] -> w183
      frame False {
        # ">>> Line Sensor Cluster>>>"
        # ">>> Line Sensor Cluster>>>"
        # ">>> Motor control cluster >>>"
        # ">>> yStepper command>>>"
        # ">>> Motor control cluster >>>"
        # ">>> yStepper command>>>"
        # ">>> Motor control cluster >>>"
        # ">>> IR Sensors >>>"
        # ">>> IR Sensors >>>"
        # ">>> yStepper command>>>"
        # ">>> Time cluster >>>"
        # ">>> Yaw >>>"
        # ">>> Stepper position >>>"
        # ">>> Encoders >>>"
        # ">>> Object detection >>>"
        # ">>> Ultrasonic Sensors Detect >>>"
        # ">>> Time cluster >>>"
        # ">>> Yaw >>>"
        # ">>> Stepper position >>>"
        # ">>> Encoders >>>"
        # ">>> Object detection >>>"
        # ">>> Ultrasonic Sensors Detect >>>"
      }
      frame True {
        # ">>> IR Sensors >>>"
        # ">>> Line Sensor Cluster>>>"
        # ">>> Line Sensor Cluster>>>"
        # ">>> Motor control cluster >>>"
        # ">>> yStepper command>>>"
        # ">>> IR Sensors >>>"
        # ">>> Motor control cluster >>>"
        # ">>State Logic Queue Reference >>"
        # ">>Timeout>>"
        # ">>> yStepper command>>>"
        # ">>> Time cluster >>>"
        # ">>> Object detection >>>"
        # ">>> Yaw >>>"
        # ">>> Ultrasonic Sensors Detect >>>"
        # ">>> Encoders >>>"
        # ">>> Stepper position >>>"
        # ">>State Logic  >>"
        # ">>True Stop Next State >>"
        # ">>Action Queue>>"
        # ">> Manual override >>"
        # ">>> Time cluster >>>"
        # ">>> Yaw >>>"
        # ">>> Stepper position >>>"
        # ">>> Encoders >>>"
        # ">>> Object detection >>>"
        # ">>> Ultrasonic Sensors Detect >>>"
        # ">>Action Queue>>"
        # ">>State Logic Queue Reference >>"
        n156 = Or(x=w272, y=w273) -> (x .or. y?=w271:bool)
        n157 = Unbundle By Name(w252) -> ("Left IR Sensor"=w253:dbl, "Arm IR Sensor"=w249:dbl)
        "Left IR Sensor" <- w253
        "Arm IR Sensor" <- w249
        n158 = Unbundle By Name(w258) -> ("Time up flag"=w259:bool)
        "Time up flag" <- w259
        n159 = Unbundle By Name(w260) -> ("Yaw"=w261:dbl, "Compass"=w255:dbl)
        n160 = Unbundle By Name(w262) -> ("y Stepper Position"=w264:u8, "z Stepper Position"=w263:u8)
        n161 = Unbundle By Name(w278) -> ("xDistance"=w275:dbl, "yDistance"=w276:dbl, "wDistance"=w277:dbl)
        n162 = Unbundle By Name(w266) -> ("Recognized Object"=w265:bool, "Object X coordinate"=w268:dbl, "Object Y coordinate"=w267:dbl)
        n163 = Unbundle By Name(w289) -> ("PING_A"=w281:u8, "PING_B"=w280:u8, "PING_C"=w279:u8, "PING_D"=w274:u8)
        n164 = Unbundle By Name(w247) -> ("Line Detected?"=w248:bool)
        n165 = case shown="40" w288 {
          tunnel: [w293 w304 w317 w327 w409 w423 w459 w512 w554 w601 w644 w698 w745 w785 w845 w890 w930 w978 w1020 w1072 w1109 w1160 w1203 w1246 w1275 w1292 w1337 w1377 w1425 w1477 w1515 w1563 w1605 w1657 w1694 w1745 w1780 w1828 w1870 w1915 w1958 w2012] -> w287
          tunnel: w286 -> [w293 w307 w318 w330 w411 w424 w468 w510 w558 w602 w650 w691 w748 w792 w835 w893 w936 w977 w1023 w1062 w1115 w1150 w1198 w1237 w1275 w1282 w1340 w1383 w1424 w1476 w1521 w1562 w1608 w1647 w1700 w1735 w1784 w1835 w1875 w1920 w1962 w2010]
          tunnel: [State_Type_Definitions,_for_0.26g_versions_and_later_2."Idle" ("Enum") State_Type_Definitions,_for_0.26g_versions_and_later_2."Idle" ("Enum") w313 w329 State_Type_Definitions,_for_0.26g_versions_and_later_2."Shutdown" ("Enum") w425 w466 w513 w555 w600 w645 w697 w746 w787 w844 w891 w937 w979 w1022 w1071 w1116 w1159 w1204 w1238 State_Type_Definitions,_for_0.26g_versions_and_later_2."Idle" ("Enum") w1291 w1338 w1384 w1426 w1478 w1522 w1564 w1607 w1656 w1701 w1744 w1781 w1829 w1871 w1916 w1959 w2013] -> w285
          tunnel: w284 -> [_ _ w316 w333 _ w430 w462 w509 w559 w609 w649 w695 w749 w791 w842 w888 w935 w975 w1024 w1069 w1114 w1157 w1201 w1245 _ w1289 w1335 w1382 w1422 w1474 w1520 w1560 w1609 w1654 w1699 w1742 w1788 w1834 w1878 w1923 w1966 w2009]
          tunnel: w283 -> [_ _ _ w332 _ w429 w461 w508 w560 w608 w648 w694 w742 w790 w841 w887 w934 w974 w1025 w1068 w1113 w1156 w1200 w1243 _ w1288 w1334 w1381 w1421 w1473 w1519 w1559 w1610 w1653 w1698 w1741 w1783 w1833 w1877 w1922 w1961 w2008]
          tunnel: w282 -> [_ _ w315 w328 _ w428 w460 w507 w561 w607 w647 w693 w741 w789 w843 w889 w933 w973 w1026 w1070 w1112 w1158 w1199 w1244 _ w1290 w1336 w1380 w1420 w1472 w1518 w1558 w1611 w1655 w1697 w1743 w1787 w1832 w1876 w1921 w1965 w2007]
          tunnel: w271 -> [_ _ _ _ _ w422 w467 w506 w562 w604 w643 w696 w747 w793 w836 w894 w931 w976 w1027 w1063 w1110 w1151 w1202 w1241 _ w1283 w1341 w1378 w1423 w1475 w1516 w1561 w1612 w1648 w1695 w1736 w1786 w1827 w1874 w1919 w1964 w2006]
          tunnel: w281 -> [_ _ _ _ _ _ _ _ _ _ _ _ _ _ _ _ _ _ _ _ _ _ _ _ _ _ _ _ _ _ _ _ _ _ _ _ _ _ _ _ _ _]
          tunnel: w280 -> [_ _ _ _ _ _ _ w505 _ _ _ w687 w730 w783 _ w880 _ _ _ _ _ _ _ _ _ _ w1327 _ _ _ _ _ _ _ _ _ _ _ _ _ _ _]
          tunnel: w279 -> [_ _ _ _ _ _ _ w504 _ _ _ w688 w731 w784 _ w881 _ _ _ _ _ _ _ _ _ _ w1328 _ _ _ _ _ _ _ _ _ _ _ _ _ _ _]
          tunnel: w277 -> [_ _ _ _ _ _ _ _ _ w606 _ _ _ _ _ _ _ _ _ _ _ _ _ _ _ _ _ _ _ _ _ _ _ _ _ _ _ _ _ _ _ _]
          tunnel: w276 -> [_ _ _ _ _ w421 _ _ w553 _ _ _ _ w788 _ _ _ _ _ _ _ _ _ _ _ _ _ _ _ _ _ _ _ _ _ _ _ _ _ _ _ _]
          tunnel: w275 -> [_ _ _ _ _ _ _ _ _ _ _ _ w736 _ _ _ _ _ _ _ _ _ _ _ _ _ _ _ _ w1463 _ _ _ _ _ _ _ _ _ _ _ _]
          tunnel: w274 -> [_ _ _ _ _ _ _ _ _ _ _ _ _ _ _ _ _ _ _ _ _ _ _ _ _ _ _ _ _ _ _ _ _ _ _ _ _ _ _ _ _ _]
          tunnel: [State_Type_Definitions,_for_0.26g_versions_and_later_2."Idle" ("Enum") State_Type_Definitions,_for_0.26g_versions_and_later_2."Idle" ("Enum") State_Type_Definitions,_for_0.26g_versions_and_later_2."Idle" ("Enum") State_Type_Definitions,_for_0.26g_versions_and_later_2."Idle" ("Enum") State_Type_Definitions,_for_0.26g_versions_and_later_2."Shutdown" ("Enum") w418 w465 w511 w556 w597 w642 w690 w744 w786 w846 w892 w929 w980 w1021 w1073 w1108 w1161 w1205 w1239 w1277 w1293 w1339 w1376 w1427 w1479 w1514 w1565 w1606 w1658 w1693 w1746 w1782 w1830 w1873 w1918 w1960 w2011] -> w270
          tunnel: w269 -> [_ _ w313 _ _ _ _ _ _ _ _ _ _ _ _ _ _ _ _ _ _ _ _ _ w1277 _ _ _ _ _ _ _ _ _ _ _ _ _ _ _ _ _]
          tunnel: w265 -> [_ _ _ _ _ _ _ _ _ _ _ _ _ _ _ _ _ _ _ _ _ _ _ w1240 _ _ _ _ _ _ _ _ _ _ _ _ _ _ _ _ _ _]
          tunnel: w268 -> [_ _ _ _ _ _ _ _ _ _ _ _ _ _ _ _ _ _ _ _ _ _ _ _ _ _ _ _ _ w1469 _ _ _ _ _ _ _ _ _ _ _ _]
          tunnel: w267 -> [_ _ _ _ _ _ _ _ _ _ _ _ _ _ _ _ _ _ w1016 _ _ _ _ _ _ _ _ _ _ _ _ _ w1601 _ _ _ _ _ _ _ _ _]
          tunnel: w264 -> [_ _ _ _ _ _ _ _ _ _ _ _ _ _ _ _ _ _ w1015 _ _ _ _ _ _ _ _ _ _ _ _ _ w1600 _ _ _ _ _ _ _ _ _]
          tunnel: w263 -> [_ _ _ _ _ _ w464 _ _ _ w640 _ _ _ w839 _ _ _ _ w1066 _ w1154 w1197 _ _ w1286 _ _ _ _ _ _ _ w1651 _ w1739 w1785 _ _ _ w1963 _]
          tunnel: w261 -> [_ _ _ _ _ _ _ _ _ _ _ _ _ _ _ _ _ _ _ _ _ _ _ _ _ _ _ _ _ _ _ _ _ _ _ _ _ _ _ _ _ _]
          tunnel: w259 -> [_ _ _ _ _ _ _ _ _ _ _ _ _ _ _ _ w927 w970 _ _ w1106 _ _ _ _ _ _ w1374 w1417 _ w1512 w1555 _ _ w1691 _ _ _ _ _ _ _]
          tunnel: w257 -> [w291 w302 w312 w325 w407 w417 w463 w503 w557 w596 w641 w689 w740 w782 w834 w885 w928 w971 w1018 w1061 w1107 w1149 w1194 w1236 w1278 w1281 w1332 w1375 w1418 w1470 w1513 w1556 w1603 w1646 w1692 w1734 w1779 w1831 w1872 w1917 w1957 w2005]
          tunnel: [w291 w301 w312 w325 w407 w417 w463 w503 w557 w596 w641 w689 w740 w782 w834 w885 w928 w971 w1017 w1061 w1107 w1149 w1194 w1236 w1278 w1281 w1332 w1375 w1418 w1470 w1513 w1556 w1602 w1646 w1692 w1734 w1779 w1831 w1872 w1917 w1957 w2005] -> w256
          tunnel: w255 -> [_ _ _ _ _ _ _ _ _ _ _ _ _ _ _ _ _ _ _ _ _ _ _ _ _ _ _ _ _ _ _ _ _ _ _ _ _ w1826 _ _ _ _]
          tunnel: [_ _ _ TRUE _ _ _ _ _ _ _ _ _ _ _ _ _ _ _ _ _ _ _ _ _ _ _ _ _ _ _ _ _ _ _ _ _ _ _ _ _ _] -> w254
          tunnel: w253 -> [_ _ _ _ _ _ _ _ _ _ _ _ _ _ _ _ _ _ _ _ _ _ _ _ _ _ _ _ _ _ _ _ _ _ _ _ _ _ _ _ _ _]
          tunnel: w251 -> [w290 w299 w311 w323 w406 w416 w458 w502 w550 w595 w637 w682 w729 w781 w833 w878 w926 w969 w1012 w1060 w1105 w1148 w1193 w1235 w1279 w1280 w1325 w1373 w1416 w1466 w1511 w1554 w1597 w1645 w1690 w1733 w1778 w1822 w1869 w1914 w1956 w2004]
          tunnel: [w290 w298 w311 w323 w406 w416 w458 w502 w550 w595 w637 w682 w729 w781 w833 w878 w926 w969 w1012 w1060 w1105 w1148 w1193 w1235 w1279 w1280 w1325 w1373 w1416 w1465 w1511 w1554 w1597 w1645 w1690 w1733 w1778 w1822 w1869 w1914 w1956 w2004] -> w250
          tunnel: w249 -> [_ _ _ _ _ _ _ _ _ _ _ _ _ _ _ _ _ _ _ _ _ _ _ _ _ _ _ _ _ _ _ _ _ _ _ _ _ _ _ w1912 _ w2003]
          tunnel: w248 -> [_ _ _ _ _ _ _ _ _ _ _ _ _ _ _ _ _ _ _ _ _ _ _ _ _ _ _ _ _ _ _ _ _ _ _ _ _ _ w1868 _ _ _]
          frame 0 {
            # ">>> yStepper command>>>"
          }
          frame 1 {
            # ">>> yStepper command>>>"
            n166 = for {
              shift-right: [w310] -> w304
              shift-left: w307 -> [w309]
              tunnel: string[] ["INIT", "RESET ARM", "RESET FLAGS", "RESET YAW", "NAVX CALIBRATE"] -> [w308] mode=indexing
              n167 = Enqueue Element(queue=w309, element=w308) -> (queue out=w310:refnum<queue>)  [unwired: 2 in, 2 out]
            }
            n168 = Bundle By Name(cluster=w302, "yStepper desired"=u8 0) -> (w301:T11)
            n169 = Bundle By Name(cluster=w299, "ySpeed"=0.0, "xSpeed"=0.0, "wSpeed"=0.0) -> (w298:T9)
          }
          frame 3 {
            # ">>> Motor control cluster >>>"
            # ">>> yStepper command>>>"
            n170 = Flush Queue(queue=w316, error in (no error)=w315) -> ()  [unwired: 3 out]
            n171 = for {
              shift-right: [w322] -> w317
              shift-left: w318 -> [w321]
              tunnel: string[] ["STOP", "RESET ENCODERS", "RESET YAW", "RESET ARM", "RESET FLAGS", "DISPOSE BUFFERS", "CAM CLOSE", ""] -> [w320] mode=indexing
              n172 = Enqueue Element(queue=w321, element=w320) -> (queue out=w322:refnum<queue>)  [unwired: 2 in, 2 out]
            }
          }
          frame 4, Default {
            (unwired) TRUE ("Green LED")
            # ">>> yStepper command>>>"
            n173 = Dequeue Element(queue=w333, timeout in ms (-1)=w332, error in (no error)=w328) -> (element=w331:T7)  [unwired: 3 out]
            n174 = case shown="\"Start Task A\"" w331 {
              tunnel: [w335 w342 w349 w356 w363 w370 w377 w379 w387 w394 w400] -> w327
              tunnel: w330 -> [w336 w343 w350 w357 w364 w371 w377 w380 w386 w393 w401]
              tunnel: [State_Type_Definitions."Task 1" ("Enum") State_Type_Definitions,_for_0.26g_versions_and_later_2."Task 2:Raise Arm" ("Enum") State_Type_Definitions,_for_0.26g_versions_and_later_2."Task 3" ("Enum") State_Type_Definitions,_for_0.26g_versions_and_later_2."Task 4_A" ("Enum") State_Type_Definitions."Task 5A: ARM CAM HEIGHT" ("Enum") State_Type_Definitions,_for_0.26g_versions_and_later_2."Task 6_A" ("Enum") State_Type_Definitions,_for_0.26g_versions_and_later_2."Idle" ("Enum") State_Type_Definitions,_for_0.26g_versions_and_later_2."Shutdown" ("Enum") State_Type_Definitions,_for_0.26g_versions_and_later_2."Task 9A: Raise Arm" ("Enum") State_Type_Definitions."Task A: RAISE ARM TO HEIGHT" ("Enum") State_Type_Definitions,_for_0.26g_versions_and_later_2."Task 8A: RAISE ARM" ("Enum")] -> w329
              frame "Start Task 1" {
                n175 = for {
                  shift-right: [w340] -> w335
                  shift-left: w336 -> [w339]
                  tunnel: string[] ["RESET ENCODERS", "RESET YAW", "FORWARD", "READ ENCODERS"] -> [w338] mode=indexing
                  n176 = Enqueue Element(queue=w339, element=w338) -> (queue out=w340:refnum<queue>)  [unwired: 2 in, 2 out]
                }
              }
              frame "Start Task 2" {
                n177 = for {
                  shift-right: [w347] -> w342
                  shift-left: w343 -> [w346]
                  tunnel: string[] ["RESET ENCODERS", "RESET YAW", "READ ULTRASONIC", "ARDUINO - ULTRASONIC"] -> [w345] mode=indexing
                  n178 = Enqueue Element(queue=w346, element=w345) -> (queue out=w347:refnum<queue>)  [unwired: 2 in, 2 out]
                }
              }
              frame "Start Task 3" {
                n179 = for {
                  shift-right: [w354] -> w349
                  shift-left: w350 -> [w353]
                  tunnel: string[] ["RESET ENCODERS", "READ ENCODERS", "R-ACW"] -> [w352] mode=indexing
                  n180 = Enqueue Element(queue=w353, element=w352) -> (queue out=w354:refnum<queue>)  [unwired: 2 in, 2 out]
                }
              }
              frame "Start Task 4" {
                n181 = for {
                  shift-right: [w361] -> w356
                  shift-left: w357 -> [w360]
                  tunnel: string[] ["RESET YAW", "RESET ENCODERS", "RESET ARM", "RESET FLAGS", "", ""] -> [w359] mode=indexing
                  n182 = Enqueue Element(queue=w360, element=w359) -> (queue out=w361:refnum<queue>)  [unwired: 2 in, 2 out]
                }
              }
              frame "Start Task 5" {
                n183 = for {
                  shift-right: [w368] -> w363
                  shift-left: w364 -> [w367]
                  tunnel: string[] ["RESET YAW", "RESET ENCODERS", "READ STEPPER VALUES", "Z STEPPER CAM HEIGHT", "", ""] -> [w366] mode=indexing
                  n184 = Enqueue Element(queue=w367, element=w366) -> (queue out=w368:refnum<queue>)  [unwired: 2 in, 2 out]
                }
              }
              frame "Start Task 6" {
                n185 = for {
                  shift-right: [w375] -> w370
                  shift-left: w371 -> [w374]
                  tunnel: string[] ["OPEN LOG CAM ", "", "", "", "", ""] -> [w373] mode=indexing
                  n186 = Enqueue Element(queue=w374, element=w373) -> (queue out=w375:refnum<queue>)  [unwired: 2 in, 2 out]
                }
              }
              frame "None", Default {
              }
              frame "Exit" {
                n187 = for {
                  shift-right: [w384] -> w379
                  shift-left: w380 -> [w383]
                  tunnel: string[] ["STOP", "RESET ENCODERS", "RESET YAW", "EXIT"] -> [w382] mode=indexing
                  n188 = Enqueue Element(queue=w383, element=w382) -> (queue out=w384:refnum<queue>)  [unwired: 2 in, 2 out]
                }
              }
              frame "Start Task 9" {
                n189 = for {
                  shift-right: [w391] -> w387
                  shift-left: w386 -> [w390]
                  tunnel: string[] ["RESET ENCODERS", "READ ENCODERS", "Z STEPPER CAM HEIGHT"] -> [w389] mode=indexing
                  n190 = Enqueue Element(queue=w390, element=w389) -> (queue out=w391:refnum<queue>)  [unwired: 2 in, 2 out]
                }
              }
              frame "Start Task A" {
                n191 = for {
                  shift-right: [w398] -> w394
                  shift-left: w393 -> [w397]
                  tunnel: string[] ["RESET ENCODERS", "READ ENCODERS", "RESET YAW", "Z STEPPER BOX HEIGHT"] -> [w396] mode=indexing
                  n192 = Enqueue Element(queue=w397, element=w396) -> (queue out=w398:refnum<queue>)  [unwired: 2 in, 2 out]
                }
              }
              frame "Start Task 8 - BALL" {
                n193 = for {
                  shift-right: [w405] -> w400
                  shift-left: w401 -> [w404]
                  tunnel: string[] ["RESET YAW", "RESET ENCODERS", "RESET ARM", "RESET FLAGS"] -> [w403] mode=indexing
                  n194 = Enqueue Element(queue=w404, element=w403) -> (queue out=w405:refnum<queue>)  [unwired: 2 in, 2 out]
                }
              }
            }
          }
          frame 5 {
            # ">>> yStepper command>>>"
            n195 = for {
              shift-right: [w415] -> w409
              shift-left: w411 -> [w414]
              tunnel: string[] ["INIT", "RESET ENCODERS", "RESET FLAGS", "CAM CLOSE", "DISPOSE BUFFERS", "EXIT", ""] -> [w413] mode=indexing
              n196 = Enqueue Element(queue=w414, element=w413) -> (queue out=w415:refnum<queue>)  [unwired: 2 in, 2 out]
            }
          }
          frame 6 {
            # ">>> yStepper command>>>"
            # "Use 250"
            n197 = Dequeue Element(queue=w430, timeout in ms (-1)=w429, error in (no error)=w428) -> (element=w427:T7)  [unwired: 3 out]
            n198 = Greater?(x=w421, y=265.0) -> (0:w419:bool)
            n199 = Or(x=w419, y=w422) -> (x .or. y?=w426:bool)
            n200 = case shown="\"None\", Default" w427 {
              tunnel: w426 -> [w433 _]
              tunnel: [w437 State_Type_Definitions,_for_0.26g_versions_and_later_2."True Stop" ("Enum")] -> w425
              tunnel: w424 -> [w434 w452]
              tunnel: [w432 w451] -> w423
              tunnel: [State_Type_Definitions,_for_0.26g_versions_and_later_2."Idle" ("Enum") State_Type_Definitions,_for_0.26g_versions_and_later_2."Shutdown" ("Enum")] -> w418
              frame "None", Default {
                n201 = case shown="True" w433 {
                  tunnel: w434 -> [w440 w446]
                  tunnel: [w439 w444] -> w432
                  frame False {
                    n202 = for {
                      shift-right: [w442] -> w439
                      shift-left: w440 -> [w443]
                      tunnel: string[] ["READ ENCODERS", "READ NAVX", "FORWARD"] ("element") -> [w441] mode=indexing
                      n203 = Enqueue Element(queue=w443, element=w441) -> (queue out=w442:refnum<queue>)  [unwired: 2 in, 2 out]
                    }
                  }
                  frame True {
                    n204 = for {
                      shift-right: [w448] -> w444
                      shift-left: w446 -> [w449]
                      tunnel: string[] ["RESET YAW", "RESET ENCODERS", "STOP", ""] -> [w447] mode=indexing
                      n205 = Enqueue Element(queue=w449, element=w447) -> (queue out=w448:refnum<queue>)  [unwired: 2 in, 2 out]
                    }
                  }
                }
                n206 = Select(t=State_Type_Definitions,_for_0.26g_versions_and_later_2."True Stop" ("Enum"), s=w433, f=State_Type_Definitions."Task 1" ("Enum")) -> (s? t:f=w437:u16)
              }
              frame "Exit" {
                n207 = for {
                  shift-right: [w456] -> w451
                  shift-left: w452 -> [w457]
                  tunnel: string[] ["STOP", "RESET ENCODERS", "RESET YAW", ""] -> [w455] mode=indexing
                  n208 = Enqueue Element(queue=w457, element=w455) -> (queue out=w456:refnum<queue>)  [unwired: 2 in, 2 out]
                }
              }
            }
          }
          frame 8 {
            # ">> Stepper height reeached >>"
            # ">>> yStepper command>>>"
            # ">> Manual override >>"
            n209 = Dequeue Element(queue=w462, timeout in ms (-1)=w461, error in (no error)=w460) -> (element=w471:T7)  [unwired: 3 out]
            n210 = Equal?(x=w464, y=u8 60) -> (x = y?=w469:bool)
            n211 = case shown="\"None\", Default" w471 {
              tunnel: [w482 State_Type_Definitions,_for_0.26g_versions_and_later_2."True Stop" ("Enum")] -> w466
              tunnel: [w480 w497] -> w459
              tunnel: w468 -> [w479 _]
              tunnel: w467 -> [w473 _]
              tunnel: [State_Type_Definitions,_for_0.26g_versions_and_later_2."Idle" ("Enum") State_Type_Definitions,_for_0.26g_versions_and_later_2."Shutdown" ("Enum")] -> w465
              tunnel: w469 -> [w472 _]
              frame "None", Default {
                # ">> WIill proceed to part ii if not manual override >>"
                # ">>If ENABLE or Trigger is set to true>>"
                n212 = Or(x=w472, y=w473) -> (x .or. y?=w474:bool)
                n213 = case shown="True" w472 {
                  tunnel: [w485 w491] -> w480
                  tunnel: w479 -> [w484 w490]
                  frame False {
                    n214 = for {
                      shift-right: [w487] -> w485
                      shift-left: w484 -> [w488]
                      tunnel: string[] ["Z STEPPER CAM HEIGHT", "READ STEPPER VALUES"] ("element") -> [w486] mode=indexing
                      n215 = Enqueue Element(queue=w488, element=w486) -> (queue out=w487:refnum<queue>)  [unwired: 2 in, 2 out]
                    }
                  }
                  frame True {
                    n216 = for {
                      shift-right: [w493] -> w491
                      shift-left: w490 -> [w494]
                      tunnel: string[] ["ARDUINO - ULTRASONIC", "READ ULTRASONIC", "", "", "", ""] -> [w492] mode=indexing
                      n217 = Enqueue Element(queue=w494, element=w492) -> (queue out=w493:refnum<queue>)  [unwired: 2 in, 2 out]
                    }
                  }
                }
                n218 = Select(t=State_Type_Definitions,_for_0.26g_versions_and_later_2."True Stop" ("Enum"), s=w473, f=State_Type_Definitions,_for_0.26g_versions_and_later_2."Task 2:Sensor Mode" ("Enum")) -> (s? t:f=w476:T6)
                n219 = Select(t=w476, s=w474, f=State_Type_Definitions,_for_0.26g_versions_and_later_2."Task 2:Raise Arm" ("Enum")) -> (s? t:f=w482:T6)
              }
              frame "Exit" {
                n220 = for {
                  shift-right: [w500] -> w497
                  shift-left: _ -> [w501]
                  tunnel: string[] ["STOP", "RESET ENCODERS", "RESET YAW", ""] -> [w499] mode=indexing
                  n221 = Enqueue Element(queue=w501, element=w499) -> (queue out=w500:refnum<queue>)  [unwired: 2 in, 2 out]
                }
              }
            }
          }
          frame 9 {
            w517 = u8 20 ("y")
            # ">>> yStepper command>>>"
            # ">>Object detected>>"
            n222 = Dequeue Element(queue=w509, timeout in ms (-1)=w508, error in (no error)=w507) -> (element=w518:T7)  [unwired: 3 out]
            n223 = Less?(x=w505, y=w517) -> (x < y?=w516:bool)
            n224 = Less?(x=w504, y=w517) -> (x < y?=w515:bool)
            n225 = Or(x=w516, y=w515) -> (x .or. y?=w514:bool)
            "Obstacle detected" <- w514
            n226 = case shown="\"None\", Default" w518 {
              tunnel: w514 -> [w521 _]
              tunnel: [w528 State_Type_Definitions,_for_0.26g_versions_and_later_2."True Stop" ("Enum")] -> w513
              tunnel: w506 -> [w520 _]
              tunnel: w510 -> [w527 w544]
              tunnel: [w526 w545] -> w512
              tunnel: [State_Type_Definitions,_for_0.26g_versions_and_later_2."Idle" ("Enum") State_Type_Definitions,_for_0.26g_versions_and_later_2."Shutdown" ("Enum")] -> w511
              frame "None", Default {
                n227 = case shown="True" w521 {
                  tunnel: w527 -> [w531 w538]
                  tunnel: [w532 w537] -> w526
                  frame False {
                    n228 = for {
                      tunnel: string[] ["READ ULTRASONIC", "STOP"] ("element") -> [w533] mode=indexing
                      shift-right: [w535] -> w532
                      shift-left: w531 -> [w534]
                      n229 = Enqueue Element(queue=w534, element=w533) -> (queue out=w535:refnum<queue>)  [unwired: 2 in, 2 out]
                    }
                  }
                  frame True {
                    n230 = for {
                      shift-right: [w540] -> w537
                      shift-left: w538 -> [w541]
                      tunnel: string[] ["RESET ENCODERS", "READ NAVX", "READ ENCODERS"] -> [w539] mode=indexing
                      n231 = Enqueue Element(queue=w541, element=w539) -> (queue out=w540:refnum<queue>)  [unwired: 2 in, 2 out]
                    }
                  }
                }
                n232 = Or(x=w521, y=w520) -> (x .or. y?=w519:bool)
                n233 = Select(t=State_Type_Definitions,_for_0.26g_versions_and_later_2."True Stop" ("Enum"), s=w520, f=State_Type_Definitions,_for_0.26g_versions_and_later_2."Task 2:Reverse Mode" ("Enum")) -> (s? t:f=w522:T6)
                n234 = Select(t=w522, s=w519, f=State_Type_Definitions,_for_0.26g_versions_and_later_2."Task 2:Sensor Mode" ("Enum")) -> (s? t:f=w528:T6)
              }
              frame "Exit" {
                n235 = for {
                  shift-right: [w548] -> w545
                  shift-left: w544 -> [w549]
                  tunnel: string[] ["STOP", "RESET ENCODERS", "RESET YAW", "ARDUINO MODE 0"] -> [w547] mode=indexing
                  n236 = Enqueue Element(queue=w549, element=w547) -> (queue out=w548:refnum<queue>)  [unwired: 2 in, 2 out]
                }
              }
            }
          }
          frame 10 {
            # ">>> yStepper command>>>"
            n237 = Dequeue Element(queue=w559, timeout in ms (-1)=w560, error in (no error)=w561) -> (element=w563:T7)  [unwired: 3 out]
            n238 = Less?(x=w553, y=-50.0) -> (x < y?=w551:bool)
            n239 = case shown="\"None\", Default" w563 {
              tunnel: [w573 State_Type_Definitions,_for_0.26g_versions_and_later_2."True Stop" ("Enum")] -> w555
              tunnel: w562 -> [w566 _]
              tunnel: w558 -> [w572 w589]
              tunnel: [w571 w590] -> w554
              tunnel: [State_Type_Definitions,_for_0.26g_versions_and_later_2."Idle" ("Enum") State_Type_Definitions,_for_0.26g_versions_and_later_2."Shutdown" ("Enum")] -> w556
              tunnel: w551 -> [w564 _]
              frame "None", Default {
                n240 = case shown="False" w564 {
                  tunnel: w572 -> [w576 w583]
                  tunnel: [w577 w582] -> w571
                  frame False {
                    n241 = for {
                      tunnel: string[] ["READ ENCODERS", "REVERSE", "READ NAVX"] ("element") -> [w578] mode=indexing
                      shift-right: [w580] -> w577
                      shift-left: w576 -> [w579]
                      n242 = Enqueue Element(queue=w579, element=w578) -> (queue out=w580:refnum<queue>)  [unwired: 2 in, 2 out]
                    }
                  }
                  frame True {
                    n243 = for {
                      shift-right: [w585] -> w582
                      shift-left: w583 -> [w586]
                      tunnel: string[] ["STOP", "ARDUINO - ULTRASONIC", "READ ULTRASONIC", "RESET ENCODERS"] -> [w584] mode=indexing
                      n244 = Enqueue Element(queue=w586, element=w584) -> (queue out=w585:refnum<queue>)  [unwired: 2 in, 2 out]
                    }
                  }
                }
                n245 = Or(x=w564, y=w566) -> (x .or. y?=w565:bool)
                n246 = Select(t=State_Type_Definitions,_for_0.26g_versions_and_later_2."True Stop" ("Enum"), s=w566, f=State_Type_Definitions,_for_0.26g_versions_and_later_2."Task 2:Sensor Mode" ("Enum")) -> (s? t:f=w567:T6)
                n247 = Select(t=w567, s=w565, f=State_Type_Definitions,_for_0.26g_versions_and_later_2."Task 2:Reverse Mode" ("Enum")) -> (s? t:f=w573:T6)
              }
              frame "Exit" {
                n248 = for {
                  shift-right: [w593] -> w590
                  shift-left: w589 -> [w594]
                  tunnel: string[] ["STOP", "RESET ENCODERS", "RESET YAW", "ARDUINO MODE 0"] -> [w592] mode=indexing
                  n249 = Enqueue Element(queue=w594, element=w592) -> (queue out=w593:refnum<queue>)  [unwired: 2 in, 2 out]
                }
              }
            }
          }
          frame 11 {
            # ">>> yStepper command>>>"
            n250 = Dequeue Element(queue=w609, timeout in ms (-1)=w608, error in (no error)=w607) -> (element=w598:T7)  [unwired: 3 out]
            n251 = Greater?(x=w606, y=160.0) -> (0:w603:bool)
            n252 = Or(x=w603, y=w604) -> (x .or. y?=w599:bool)
            n253 = case shown="\"None\", Default" w598 {
              tunnel: w599 -> [w612 _]
              tunnel: [w616 State_Type_Definitions,_for_0.26g_versions_and_later_2."True Stop" ("Enum")] -> w600
              tunnel: w602 -> [w613 w632]
              tunnel: [w611 w631] -> w601
              tunnel: [State_Type_Definitions,_for_0.26g_versions_and_later_2."Idle" ("Enum") State_Type_Definitions,_for_0.26g_versions_and_later_2."Shutdown" ("Enum")] -> w597
              frame "None", Default {
                n254 = case shown="False" w612 {
                  tunnel: w613 -> [w619 w625]
                  tunnel: [w618 w623] -> w611
                  frame False {
                    n255 = for {
                      shift-right: [w621] -> w618
                      shift-left: w619 -> [w622]
                      tunnel: string[] ["READ ENCODERS", "R-CW"] ("element") -> [w620] mode=indexing
                      n256 = Enqueue Element(queue=w622, element=w620) -> (queue out=w621:refnum<queue>)  [unwired: 2 in, 2 out]
                    }
                  }
                  frame True {
                    n257 = for {
                      shift-right: [w627] -> w623
                      shift-left: w625 -> [w628]
                      tunnel: string[] ["RESET YAW", "RESET ENCODERS", "STOP", "ARDUINO MODE 0"] -> [w626] mode=indexing
                      n258 = Enqueue Element(queue=w628, element=w626) -> (queue out=w627:refnum<queue>)  [unwired: 2 in, 2 out]
                    }
                  }
                }
                n259 = Select(t=State_Type_Definitions,_for_0.26g_versions_and_later_2."True Stop" ("Enum"), s=w612, f=State_Type_Definitions,_for_0.26g_versions_and_later_2."Task 3" ("Enum")) -> (s? t:f=w616:T6)
              }
              frame "Exit" {
                n260 = for {
                  shift-right: [w635] -> w631
                  shift-left: w632 -> [w636]
                  tunnel: string[] ["STOP", "RESET ENCODERS", "RESET YAW", ""] -> [w634] mode=indexing
                  n261 = Enqueue Element(queue=w636, element=w634) -> (queue out=w635:refnum<queue>)  [unwired: 2 in, 2 out]
                }
              }
            }
          }
          frame 12 {
            # ">> Stepper height reeached >>"
            # ">>> yStepper command>>>"
            # ">> Manual override >>"
            n262 = Dequeue Element(queue=w649, timeout in ms (-1)=w648, error in (no error)=w647) -> (element=w646:T7)  [unwired: 3 out]
            n263 = Equal?(x=w640, y=u8 60) -> (x = y?=w638:bool)
            n264 = case shown="\"Exit\"" w646 {
              tunnel: [w661 State_Type_Definitions,_for_0.26g_versions_and_later_2."True Stop" ("Enum")] -> w645
              tunnel: [w659 w677] -> w644
              tunnel: w650 -> [w658 w674]
              tunnel: w643 -> [w652 _]
              tunnel: [State_Type_Definitions,_for_0.26g_versions_and_later_2."Idle" ("Enum") State_Type_Definitions,_for_0.26g_versions_and_later_2."Shutdown" ("Enum")] -> w642
              tunnel: w638 -> [w651 _]
              frame "None", Default {
                # ">> WIill proceed to part ii if not manual override >>"
                # ">>If ENABLE or Trigger is set to true>>"
                n265 = Or(x=w651, y=w652) -> (x .or. y?=w653:bool)
                n266 = case shown="False" w651 {
                  tunnel: [w664 w670] -> w659
                  tunnel: w658 -> [w663 w669]
                  frame False {
                    n267 = for {
                      shift-right: [w666] -> w664
                      shift-left: w663 -> [w667]
                      tunnel: string[] ["Z STEPPER CAM HEIGHT", "READ STEPPER VALUES"] ("element") -> [w665] mode=indexing
                      n268 = Enqueue Element(queue=w667, element=w665) -> (queue out=w666:refnum<queue>)  [unwired: 2 in, 2 out]
                    }
                  }
                  frame True {
                    n269 = for {
                      shift-right: [w672] -> w670
                      shift-left: w669 -> [w673]
                      tunnel: string[] ["ARDUINO - ULTRASONIC", "READ ULTRASONIC", "FORWARD", "", "", ""] -> [w671] mode=indexing
                      n270 = Enqueue Element(queue=w673, element=w671) -> (queue out=w672:refnum<queue>)  [unwired: 2 in, 2 out]
                    }
                  }
                }
                n271 = Select(t=State_Type_Definitions,_for_0.26g_versions_and_later_2."True Stop" ("Enum"), s=w652, f=State_Type_Definitions,_for_0.26g_versions_and_later_2."Task 4_B" ("Enum")) -> (s? t:f=w655:T6)
                n272 = Select(t=w655, s=w653, f=State_Type_Definitions,_for_0.26g_versions_and_later_2."Task 4_A" ("Enum")) -> (s? t:f=w661:T6)
              }
              frame "Exit" {
                n273 = for {
                  shift-right: [w680] -> w677
                  shift-left: w674 -> [w681]
                  tunnel: string[] ["STOP", "RESET ENCODERS", "RESET YAW", ""] -> [w679] mode=indexing
                  n274 = Enqueue Element(queue=w681, element=w679) -> (queue out=w680:refnum<queue>)  [unwired: 2 in, 2 out]
                }
              }
            }
          }
          frame 13 {
            w686 = u8 20
            # ">> Path blocked >>"
            # ">>> yStepper command>>>"
            # ">> Manual override >>"
            n275 = Dequeue Element(queue=w695, timeout in ms (-1)=w694, error in (no error)=w693) -> (element=w692:T7)  [unwired: 3 out]
            n276 = Less?(x=w688, y=w686) -> (x < y?=w683:bool)
            n277 = Less?(x=w687, y=w686) -> (x < y?=w684:bool)
            n278 = And(x=w684, y=w683) -> (x .and. y?=w685:bool)
            n279 = case shown="\"None\", Default" w692 {
              tunnel: [w709 State_Type_Definitions,_for_0.26g_versions_and_later_2."True Stop" ("Enum")] -> w697
              tunnel: [w707 w724] -> w698
              tunnel: w691 -> [w706 _]
              tunnel: w696 -> [w700 _]
              tunnel: [State_Type_Definitions,_for_0.26g_versions_and_later_2."Idle" ("Enum") State_Type_Definitions,_for_0.26g_versions_and_later_2."Shutdown" ("Enum")] -> w690
              tunnel: w685 -> [w699 _]
              frame "None", Default {
                # ">> Manual override forces program to true stop >>"
                # ">>If ENABLE or Trigger is set to true>>"
                n280 = Or(x=w699, y=w700) -> (x .or. y?=w705:bool)
                n281 = case shown="True" w699 {
                  tunnel: [w712 w717] -> w707
                  tunnel: w706 -> [w711 w716]
                  frame False {
                    n282 = for {
                      shift-right: [w714] -> w712
                      shift-left: w711 -> [w715]
                      tunnel: string[] ["FORWARD", "READ ULTRASONIC", "READ NAVX"] ("element") -> [w713] mode=indexing
                      n283 = Enqueue Element(queue=w715, element=w713) -> (queue out=w714:refnum<queue>)  [unwired: 2 in, 2 out]
                    }
                  }
                  frame True {
                    n284 = for {
                      shift-right: [w720] -> w717
                      shift-left: w716 -> [w721]
                      tunnel: string[] ["STOP", "RESET YAW", "RESET ENCODERS", "RESET FLAGS"] -> [w719] mode=indexing
                      n285 = Enqueue Element(queue=w721, element=w719) -> (queue out=w720:refnum<queue>)  [unwired: 2 in, 2 out]
                    }
                  }
                }
                n286 = Select(t=State_Type_Definitions,_for_0.26g_versions_and_later_2."True Stop" ("Enum"), s=w700, f=State_Type_Definitions,_for_0.26g_versions_and_later_2."Task 4_C" ("Enum")) -> (s? t:f=w702:T6)
                n287 = Select(t=w702, s=w705, f=State_Type_Definitions,_for_0.26g_versions_and_later_2."Task 4_B" ("Enum")) -> (s? t:f=w709:T6)
              }
              frame "Exit" {
                n288 = for {
                  shift-right: [w727] -> w724
                  shift-left: _ -> [w728]
                  tunnel: string[] ["STOP", "RESET ENCODERS", "RESET YAW", ""] -> [w726] mode=indexing
                  n289 = Enqueue Element(queue=w728, element=w726) -> (queue out=w727:refnum<queue>)  [unwired: 2 in, 2 out]
                }
              }
            }
          }
          frame 14 {
            w739 = u8 20
            # ">> xDistance travelled>>"
            # ">> Path NOT blocked >>"
            # ">>> yStepper command>>>"
            # ">> Manual override >>"
            n290 = Dequeue Element(queue=w749, timeout in ms (-1)=w742, error in (no error)=w741) -> (element=w743:T7)  [unwired: 3 out]
            n291 = Greater?(x=w731, y=w739) -> (0:w737:bool)
            n292 = Greater?(x=w736, y=80.0) -> (0:w734:bool)
            n293 = Greater?(x=w730, y=w739) -> (0:w738:bool)
            n294 = And(x=w738, y=w737) -> (x .and. y?=w733:bool)
            n295 = And(x=w734, y=w733) -> (x .and. y?=w732:bool)
            n296 = case shown="\"Exit\"" w743 {
              tunnel: [w760 State_Type_Definitions,_for_0.26g_versions_and_later_2."True Stop" ("Enum")] -> w746
              tunnel: [w758 w776] -> w745
              tunnel: w748 -> [w757 w773]
              tunnel: w747 -> [w751 _]
              tunnel: [State_Type_Definitions,_for_0.26g_versions_and_later_2."Idle" ("t") State_Type_Definitions,_for_0.26g_versions_and_later_2."Shutdown" ("Enum")] -> w744
              tunnel: w732 -> [w750 _]
              frame "None", Default {
                # ">> Manual override forces program to true stop >>"
                # ">>If ENABLE or Trigger is set to true>>"
                n297 = Or(x=w750, y=w751) -> (x .or. y?=w756:bool)
                n298 = case shown="False" w750 {
                  tunnel: [w763 w768] -> w758
                  tunnel: w757 -> [w761 w767]
                  frame False {
                    n299 = for {
                      shift-right: [w765] -> w763
                      shift-left: w761 -> [w766]
                      tunnel: string[] ["RIGHT", "READ NAVX", "READ ENCODERS", "READ ULTRASONIC"] ("element") -> [w764] mode=indexing
                      n300 = Enqueue Element(queue=w766, element=w764) -> (queue out=w765:refnum<queue>)  [unwired: 2 in, 2 out]
                    }
                  }
                  frame True {
                    n301 = for {
                      shift-right: [w771] -> w768
                      shift-left: w767 -> [w772]
                      tunnel: string[] ["STOP", "RESET YAW", "RESET ENCODERS", "ARDUINO - ULTRASONIC"] -> [w770] mode=indexing
                      n302 = Enqueue Element(queue=w772, element=w770) -> (queue out=w771:refnum<queue>)  [unwired: 2 in, 2 out]
                    }
                  }
                }
                n303 = Select(t=State_Type_Definitions,_for_0.26g_versions_and_later_2."True Stop" ("Enum"), s=w751, f=State_Type_Definitions,_for_0.26g_versions_and_later_2."Task 4_D" ("Enum")) -> (s? t:f=w752:T6)
                n304 = Select(t=w752, s=w756, f=State_Type_Definitions,_for_0.26g_versions_and_later_2."Task 4_C" ("Enum")) -> (s? t:f=w760:T6)
              }
              frame "Exit" {
                n305 = for {
                  shift-right: [w779] -> w776
                  shift-left: w773 -> [w780]
                  tunnel: string[] ["STOP", "RESET ENCODERS", "RESET YAW", ""] -> [w778] mode=indexing
                  n306 = Enqueue Element(queue=w780, element=w778) -> (queue out=w779:refnum<queue>)  [unwired: 2 in, 2 out]
                }
              }
            }
          }
          frame 15 {
            w800 = u8 20
            # ">> yDistance travelled>>"
            # ">> Path blocked >>"
            # ">>> yStepper command>>>"
            # ">> Manual override >>"
            n307 = Dequeue Element(queue=w791, timeout in ms (-1)=w790, error in (no error)=w789) -> (element=w801:T7)  [unwired: 3 out]
            n308 = Less?(x=w784, y=w800) -> (x < y?=w798:bool)
            n309 = Greater?(x=w788, y=200.0) -> (0:w796:bool)
            n310 = Less?(x=w783, y=w800) -> (x < y?=w799:bool)
            n311 = And(x=w799, y=w798) -> (x .and. y?=w795:bool)
            n312 = Or(x=w796, y=w795) -> (x .or. y?=w794:bool)
            n313 = case shown="\"None\", Default" w801 {
              tunnel: [w812 State_Type_Definitions,_for_0.26g_versions_and_later_2."True Stop" ("Enum")] -> w787
              tunnel: [w810 w828] -> w785
              tunnel: w792 -> [w809 w825]
              tunnel: w793 -> [w803 _]
              tunnel: [State_Type_Definitions,_for_0.26g_versions_and_later_2."Idle" ("t") State_Type_Definitions,_for_0.26g_versions_and_later_2."Shutdown" ("Enum")] -> w786
              tunnel: w794 -> [w802 _]
              frame "None", Default {
                # ">> Manual override forces program to true stop >>"
                # ">>If ENABLE or Trigger is set to true>>"
                n314 = Or(x=w802, y=w803) -> (x .or. y?=w808:bool)
                n315 = case shown="True" w802 {
                  tunnel: [w815 w820] -> w810
                  tunnel: w809 -> [w813 w819]
                  frame False {
                    n316 = for {
                      shift-right: [w817] -> w815
                      shift-left: w813 -> [w818]
                      tunnel: string[] ["FORWARD", "READ NAVX", "READ ENCODERS", "READ ULTRASONIC"] ("element") -> [w816] mode=indexing
                      n317 = Enqueue Element(queue=w818, element=w816) -> (queue out=w817:refnum<queue>)  [unwired: 2 in, 2 out]
                    }
                  }
                  frame True {
                    n318 = for {
                      shift-right: [w823] -> w820
                      shift-left: w819 -> [w824]
                      tunnel: string[] ["STOP", "RESET YAW", "RESET ENCODERS", "RESET FLAGS"] -> [w822] mode=indexing
                      n319 = Enqueue Element(queue=w824, element=w822) -> (queue out=w823:refnum<queue>)  [unwired: 2 in, 2 out]
                    }
                  }
                }
                n320 = Select(t=State_Type_Definitions,_for_0.26g_versions_and_later_2."True Stop" ("Enum"), s=w803, f=State_Type_Definitions,_for_0.26g_versions_and_later_2."True Stop" ("Enum")) -> (s? t:f=w804:T6)
                n321 = Select(t=w804, s=w808, f=State_Type_Definitions,_for_0.26g_versions_and_later_2."Task 4_D" ("Enum")) -> (s? t:f=w812:T6)
              }
              frame "Exit" {
                n322 = for {
                  shift-right: [w831] -> w828
                  shift-left: w825 -> [w832]
                  tunnel: string[] ["STOP", "RESET ENCODERS", "RESET YAW", ""] -> [w830] mode=indexing
                  n323 = Enqueue Element(queue=w832, element=w830) -> (queue out=w831:refnum<queue>)  [unwired: 2 in, 2 out]
                }
              }
            }
          }
          frame 15 {
            # ">>> yStepper command>>>"
            # ">> Manual override >>"
            n324 = Dequeue Element(queue=w842, timeout in ms (-1)=w841, error in (no error)=w843) -> (element=w840:T7)  [unwired: 3 out]
            n325 = Equal?(x=w839, y=u8 60) -> (x = y?=w837:bool)
            n326 = case shown="\"None\", Default" w840 {
              tunnel: [w853 State_Type_Definitions,_for_0.26g_versions_and_later_2."True Stop" ("Enum")] -> w844
              tunnel: [w856 w873] -> w845
              tunnel: [State_Type_Definitions,_for_0.26g_versions_and_later_2."Idle" ("Enum") State_Type_Definitions,_for_0.26g_versions_and_later_2."Shutdown" ("Enum")] -> w846
              tunnel: w837 -> [w852 _]
              tunnel: w836 -> [w851 _]
              tunnel: w835 -> [w847 w870]
              frame "None", Default {
                # "Stays in Task 5_A until stepper reaches desired \nheight"
                # "T: Go back to idle, F: Continue with task\""
                # ">> Manual override >>"
                n327 = case shown="True" w852 {
                  tunnel: [w860 w866] -> w856
                  tunnel: w847 -> [w858 w864]
                  frame False {
                    n328 = for {
                      tunnel: string[] ["Z STEPPER CAM HEIGHT", "READ STEPPER VALUES"] ("element") -> [w861] mode=indexing
                      shift-right: [w863] -> w860
                      shift-left: w858 -> [w862]
                      n329 = Enqueue Element(queue=w862, element=w861) -> (queue out=w863:refnum<queue>)  [unwired: 2 in, 2 out]
                    }
                  }
                  frame True {
                    n330 = for {
                      shift-right: [w868] -> w866
                      shift-left: w864 -> [w869]
                      tunnel: string[] ["ARDUINO - ULTRASONIC", "READ ULTRASONIC", ""] -> [w867] mode=indexing
                      n331 = Enqueue Element(queue=w869, element=w867) -> (queue out=w868:refnum<queue>)  [unwired: 2 in, 2 out]
                    }
                  }
                }
                n332 = Or(x=w852, y=w851) -> (x .or. y?=w854:bool)
                n333 = Select(t=State_Type_Definitions,_for_0.26g_versions_and_later_2."True Stop" ("Enum"), s=w851, f=State_Type_Definitions."Task 5B: MOVE TO BOX" ("Enum")) -> (s? t:f=w848:u16)
                n334 = Select(t=w848, s=w854, f=State_Type_Definitions."Task 5A: ARM CAM HEIGHT" ("Enum")) -> (s? t:f=w853:u16)
              }
              frame "Exit" {
                n335 = for {
                  shift-right: [w876] -> w873
                  shift-left: w870 -> [w877]
                  tunnel: string[] ["STOP", "RESET ENCODERS", "RESET YAW", "ARDUINO MODE 0"] -> [w875] mode=indexing
                  n336 = Enqueue Element(queue=w877, element=w875) -> (queue out=w876:refnum<queue>)  [unwired: 2 in, 2 out]
                }
              }
            }
          }
          frame 16 {
            w884 = u8 20 ("y")
            # ">>> yStepper command>>>"
            n337 = Less?(x=w881, y=w884) -> (x < y?=w882:bool)
            n338 = Dequeue Element(queue=w888, timeout in ms (-1)=w887, error in (no error)=w889) -> (element=w886:T7)  [unwired: 3 out]
            n339 = Less?(x=w880, y=w884) -> (x < y?=w883:bool)
            n340 = And(x=w883, y=w882) -> (x .and. y?=w879:bool)
            n341 = case shown="\"None\", Default" w886 {
              tunnel: [w901 State_Type_Definitions,_for_0.26g_versions_and_later_2."True Stop" ("Enum")] -> w891
              tunnel: [w904 w921] -> w890
              tunnel: [State_Type_Definitions,_for_0.26g_versions_and_later_2."Idle" ("Enum") State_Type_Definitions,_for_0.26g_versions_and_later_2."Shutdown" ("Enum")] -> w892
              tunnel: w894 -> [w900 _]
              tunnel: w893 -> [w896 w918]
              tunnel: w879 -> [w895 _]
              frame "None", Default {
                # "Stays in Task 5_B to capture image over 5 seconds"
                # "T: Go back to idle, F: Continue with task\""
                # ">> Manual override >>"
                n342 = case shown="True" w895 {
                  tunnel: [w908 w914] -> w904
                  tunnel: w896 -> [w906 w912]
                  frame False {
                    n343 = for {
                      tunnel: string[] ["FORWARD", "READ ULTRASONIC", "READ NAVX"] ("element") -> [w909] mode=indexing
                      shift-right: [w911] -> w908
                      shift-left: w906 -> [w910]
                      n344 = Enqueue Element(queue=w910, element=w909) -> (queue out=w911:refnum<queue>)  [unwired: 2 in, 2 out]
                    }
                  }
                  frame True {
                    n345 = for {
                      shift-right: [w916] -> w914
                      shift-left: w912 -> [w917]
                      tunnel: string[] ["STOP", "RESET ENCODERS", "OPEN LOG CAM", "SET TIMER 5"] -> [w915] mode=indexing
                      n346 = Enqueue Element(queue=w917, element=w915) -> (queue out=w916:refnum<queue>)  [unwired: 2 in, 2 out]
                    }
                  }
                }
                n347 = Or(x=w895, y=w900) -> (x .or. y?=w902:bool)
                n348 = Select(t=State_Type_Definitions,_for_0.26g_versions_and_later_2."True Stop" ("Enum"), s=w900, f=State_Type_Definitions."Task 5C: CAM BURST" ("Enum")) -> (s? t:f=w897:u16)
                n349 = Select(t=w897, s=w902, f=State_Type_Definitions."Task 5B: MOVE TO BOX" ("Enum")) -> (s? t:f=w901:u16)
              }
              frame "Exit" {
                n350 = for {
                  shift-right: [w924] -> w921
                  shift-left: w918 -> [w925]
                  tunnel: string[] ["STOP", "RESET ENCODERS", "RESET YAW", "ARDUINO MODE 0"] -> [w923] mode=indexing
                  n351 = Enqueue Element(queue=w925, element=w923) -> (queue out=w924:refnum<queue>)  [unwired: 2 in, 2 out]
                }
              }
            }
          }
          frame 17 {
            # ">>> Motor control cluster >>>"
            # ">>> yStepper command>>>"
            # ">> Manual override >>"
            n352 = Dequeue Element(queue=w935, timeout in ms (-1)=w934, error in (no error)=w933) -> (element=w932:T7)  [unwired: 3 out]
            n353 = case shown="\"None\", Default" w932 {
              tunnel: [w944 State_Type_Definitions,_for_0.26g_versions_and_later_2."True Stop" ("Enum")] -> w937
              tunnel: [w947 w964] -> w930
              tunnel: [State_Type_Definitions,_for_0.26g_versions_and_later_2."Idle" ("Enum") State_Type_Definitions,_for_0.26g_versions_and_later_2."Shutdown" ("Enum")] -> w929
              tunnel: w931 -> [w938 _]
              tunnel: w936 -> [w943 w961]
              tunnel: w927 -> [w942 _]
              frame "None", Default {
                # ">> Is time up? >>"
                # "Determines if object is in range to pick up"
                # ">> Manual override >>"
                n354 = case shown="False" w942 {
                  tunnel: [w951 w957] -> w947
                  tunnel: w943 -> [w949 w955]
                  frame False {
                    n355 = for {
                      tunnel: string[] ["CAM ACQ", "START TIMER"] ("element") -> [w952] mode=indexing
                      shift-right: [w954] -> w951
                      shift-left: w949 -> [w953]
                      n356 = Enqueue Element(queue=w953, element=w952) -> (queue out=w954:refnum<queue>)  [unwired: 2 in, 2 out]
                    }
                  }
                  frame True {
                    n357 = for {
                      shift-right: [w959] -> w957
                      shift-left: w955 -> [w960]
                      tunnel: string[] ["CAM CLOSE", "PROCESS IMAGE", "SET TIMER 5"] -> [w958] mode=indexing
                      n358 = Enqueue Element(queue=w960, element=w958) -> (queue out=w959:refnum<queue>)  [unwired: 2 in, 2 out]
                    }
                  }
                }
                n359 = Or(x=w942, y=w938) -> (x .or. y?=w945:bool)
                n360 = Select(t=State_Type_Definitions,_for_0.26g_versions_and_later_2."True Stop" ("Enum"), s=w938, f=State_Type_Definitions."Task 5D: PROCESS IMAGE" ("Enum")) -> (s? t:f=w940:u16)
                n361 = Select(t=w940, s=w945, f=State_Type_Definitions."Task 5C: CAM BURST" ("Enum")) -> (s? t:f=w944:u16)
              }
              frame "Exit" {
                n362 = for {
                  shift-right: [w967] -> w964
                  shift-left: w961 -> [w968]
                  tunnel: string[] ["STOP", "RESET ENCODERS", "RESET YAW", "ARDUINO MODE 0"] -> [w966] mode=indexing
                  n363 = Enqueue Element(queue=w968, element=w966) -> (queue out=w967:refnum<queue>)  [unwired: 2 in, 2 out]
                }
              }
            }
          }
          frame 18 {
            # ">>> yStepper command>>>"
            n364 = Dequeue Element(queue=w975, timeout in ms (-1)=w974, error in (no error)=w973) -> (element=w972:T7)  [unwired: 3 out]
            n365 = case shown="\"None\", Default" w972 {
              tunnel: [w987 State_Type_Definitions,_for_0.26g_versions_and_later_2."True Stop" ("Enum")] -> w979
              tunnel: [w990 w1007] -> w978
              tunnel: [State_Type_Definitions,_for_0.26g_versions_and_later_2."Idle" ("Enum") State_Type_Definitions,_for_0.26g_versions_and_later_2."Shutdown" ("Enum")] -> w980
              tunnel: w976 -> [w986 _]
              tunnel: w977 -> [w982 w1004]
              tunnel: w970 -> [w981 _]
              frame "None", Default {
                # ">> T: Breaks out of state loop; F: Stays in loop>>"
                # ">> Manual override >>"
                # ">> Checks if time is up>>"
                # "Stays in Task 5D until the object is detected"
                # "T: Go back to idle, F: Continue with task\""
                # ">> Manual override >>"
                n366 = case shown="True" w981 {
                  tunnel: [w994 w1000] -> w990
                  tunnel: w982 -> [w992 w998]
                  frame False {
                    n367 = for {
                      tunnel: string[] ["START TIMER", "PROCESS IMAGE", ""] ("element") -> [w995] mode=indexing
                      shift-right: [w997] -> w994
                      shift-left: w992 -> [w996]
                      n368 = Enqueue Element(queue=w996, element=w995) -> (queue out=w997:refnum<queue>)  [unwired: 2 in, 2 out]
                    }
                  }
                  frame True {
                    n369 = for {
                      shift-right: [w1002] -> w1000
                      shift-left: w998 -> [w1003]
                      tunnel: string[] ["CAM CLOSE", "", ""] -> [w1001] mode=indexing
                      n370 = Enqueue Element(queue=w1003, element=w1001) -> (queue out=w1002:refnum<queue>)  [unwired: 2 in, 2 out]
                    }
                  }
                }
                n371 = Or(x=w981, y=w986) -> (x .or. y?=w988:bool)
                n372 = Select(t=State_Type_Definitions,_for_0.26g_versions_and_later_2."True Stop" ("Enum"), s=w986, f=State_Type_Definitions,_for_0.26g_versions_and_later_2."Task 5E: POSITION ARM" ("Enum")) -> (s? t:f=w983:T6)
                n373 = Select(t=w983, s=w988, f=State_Type_Definitions."Task 5D: PROCESS IMAGE" ("Enum")) -> (s? t:f=w987:u16)
              }
              frame "Exit" {
                n374 = for {
                  shift-right: [w1010] -> w1007
                  shift-left: w1004 -> [w1011]
                  tunnel: string[] ["STOP", "RESET ENCODERS", "RESET YAW", "ARDUINO MODE 0"] -> [w1009] mode=indexing
                  n375 = Enqueue Element(queue=w1011, element=w1009) -> (queue out=w1010:refnum<queue>)  [unwired: 2 in, 2 out]
                }
              }
            }
          }
          frame 20 {
            # ">>> yStepper command>>>"
            n376 = Dequeue Element(queue=w1024, timeout in ms (-1)=w1025, error in (no error)=w1026) -> (element=w1028:T7)  [unwired: 3 out]
            n377 = formula code="if (pos < 100)\ny = 41;\n\nelse if (pos >= 100 && pos <= 140)\ny = 30;\n\nelse if (pos >= 141 && pos <= 170)\ny = 25;\n\nelse if (pos >= 171 &&pos <= 180) \ny = 20;\n\nelse if (pos >= 181&& pos <= 200)\ny = 15;\n\nelse if (pos >= 201 && pos <= 230)\ny = 10;\n\nelse if (pos >= 231 && pos <= 320)\ny = 8;\n\nelse if (pos > 320)\ny = 0;"("pos"=w1016) -> ("y"=w1019:dbl)
            n378 = To Unsigned Byte Integer(number=w1019) -> (unsigned 8bit integer=w1014:u8)
            n379 = Equal?(x=w1015, y=w1014) -> (x = y?=w1013:bool)
            n380 = case shown="\"None\", Default" w1028 {
              tunnel: [w1035 State_Type_Definitions,_for_0.26g_versions_and_later_2."True Stop" ("Enum")] -> w1022
              tunnel: [w1038 w1055] -> w1020
              tunnel: [State_Type_Definitions,_for_0.26g_versions_and_later_2."Idle" ("Enum") State_Type_Definitions,_for_0.26g_versions_and_later_2."Shutdown" ("Enum")] -> w1021
              tunnel: w1027 -> [w1034 _]
              tunnel: w1023 -> [w1030 w1052]
              tunnel: w1013 -> [w1029 _]
              frame "None", Default {
                # ">> T: Breaks out of state loop; F: Stays in loop>>"
                # ">> Manual override >>"
                # ">> Checks if time is up>>"
                # "Stays in Task 5D until the object is detected"
                # "T: Go back to idle, F: Continue with task\""
                # ">> Manual override >>"
                n381 = case shown="False" w1029 {
                  tunnel: [w1042 w1048] -> w1038
                  tunnel: w1030 -> [w1040 w1046]
                  frame False {
                    n382 = for {
                      tunnel: string[] ["READ STEPPER VALUES", "Y STEPPER CONTROL", ""] ("element") -> [w1043] mode=indexing
                      shift-right: [w1045] -> w1042
                      shift-left: w1040 -> [w1044]
                      n383 = Enqueue Element(queue=w1044, element=w1043) -> (queue out=w1045:refnum<queue>)  [unwired: 2 in, 2 out]
                    }
                  }
                  frame True {
                    n384 = for {
                      shift-right: [w1050] -> w1048
                      shift-left: w1046 -> [w1051]
                      tunnel: string[] ["CAM CLOSE", "DISPOSE BUFFERS", ""] -> [w1049] mode=indexing
                      n385 = Enqueue Element(queue=w1051, element=w1049) -> (queue out=w1050:refnum<queue>)  [unwired: 2 in, 2 out]
                    }
                  }
                }
                n386 = Or(x=w1029, y=w1034) -> (x .or. y?=w1036:bool)
                n387 = Select(t=State_Type_Definitions,_for_0.26g_versions_and_later_2."True Stop" ("Enum"), s=w1034, f=State_Type_Definitions,_for_0.26g_versions_and_later_2."Task 5F: ARM GRAB HEIGHT" ("Enum")) -> (s? t:f=w1031:T6)
                n388 = Select(t=w1031, s=w1036, f=State_Type_Definitions,_for_0.26g_versions_and_later_2."Task 5E: POSITION ARM" ("Enum")) -> (s? t:f=w1035:T6)
              }
              frame "Exit" {
                n389 = for {
                  shift-right: [w1058] -> w1055
                  shift-left: w1052 -> [w1059]
                  tunnel: string[] ["STOP", "RESET ENCODERS", "RESET YAW", "ARDUINO MODE 0"] -> [w1057] mode=indexing
                  n390 = Enqueue Element(queue=w1059, element=w1057) -> (queue out=w1058:refnum<queue>)  [unwired: 2 in, 2 out]
                }
              }
            }
            n391 = Bundle By Name(cluster=w1018, "yStepper desired"=w1014) -> (w1017:T11)
          }
          frame 21 {
            # ">>> Motor control cluster >>>"
            # ">>> yStepper command>>>"
            # ">> Manual override >>"
            n392 = Dequeue Element(queue=w1069, timeout in ms (-1)=w1068, error in (no error)=w1070) -> (element=w1067:T7)  [unwired: 3 out]
            n393 = Equal?(x=w1066, y=u8 1) -> (x = y?=w1064:bool)
            n394 = case shown="\"None\", Default" w1067 {
              tunnel: [w1080 State_Type_Definitions,_for_0.26g_versions_and_later_2."True Stop" ("Enum")] -> w1071
              tunnel: [w1083 w1100] -> w1072
              tunnel: [State_Type_Definitions,_for_0.26g_versions_and_later_2."Idle" ("Enum") State_Type_Definitions,_for_0.26g_versions_and_later_2."Shutdown" ("Enum")] -> w1073
              tunnel: w1064 -> [w1079 _]
              tunnel: w1063 -> [w1078 _]
              tunnel: w1062 -> [w1074 w1097]
              frame "None", Default {
                # "Stays in Task 5F until stepper reaches desired \nheight"
                # "T: Go back to idle, F: Continue with task\""
                # ">> Manual override >>"
                n395 = case shown="True" w1079 {
                  tunnel: [w1087 w1093] -> w1083
                  tunnel: w1074 -> [w1085 w1091]
                  frame False {
                    n396 = for {
                      tunnel: string[] ["Z STEPPER GRAB HEIGHT", "READ STEPPER VALUES"] ("element") -> [w1088] mode=indexing
                      shift-right: [w1090] -> w1087
                      shift-left: w1085 -> [w1089]
                      n397 = Enqueue Element(queue=w1089, element=w1088) -> (queue out=w1090:refnum<queue>)  [unwired: 2 in, 2 out]
                    }
                  }
                  frame True {
                    n398 = for {
                      shift-right: [w1095] -> w1093
                      shift-left: w1091 -> [w1096]
                      tunnel: string[] ["SET TIMER 5", "CLOSE CLAW", ""] -> [w1094] mode=indexing
                      n399 = Enqueue Element(queue=w1096, element=w1094) -> (queue out=w1095:refnum<queue>)  [unwired: 2 in, 2 out]
                    }
                  }
                }
                n400 = Or(x=w1079, y=w1078) -> (x .or. y?=w1081:bool)
                n401 = Select(t=State_Type_Definitions,_for_0.26g_versions_and_later_2."True Stop" ("Enum"), s=w1078, f=State_Type_Definitions,_for_0.26g_versions_and_later_2."Task 5G: CLOSE CLAW" ("Enum")) -> (s? t:f=w1075:T6)
                n402 = Select(t=w1075, s=w1081, f=State_Type_Definitions,_for_0.26g_versions_and_later_2."Task 5F: ARM GRAB HEIGHT" ("Enum")) -> (s? t:f=w1080:T6)
              }
              frame "Exit" {
                n403 = for {
                  shift-right: [w1103] -> w1100
                  shift-left: w1097 -> [w1104]
                  tunnel: string[] ["STOP", "RESET ENCODERS", "RESET YAW", "ARDUINO MODE 0"] -> [w1102] mode=indexing
                  n404 = Enqueue Element(queue=w1104, element=w1102) -> (queue out=w1103:refnum<queue>)  [unwired: 2 in, 2 out]
                }
              }
            }
          }
          frame 22 {
            # ">>> yStepper command>>>"
            # ">> Manual override >>"
            n405 = Dequeue Element(queue=w1114, timeout in ms (-1)=w1113, error in (no error)=w1112) -> (element=w1111:T7)  [unwired: 3 out]
            n406 = case shown="\"None\", Default" w1111 {
              tunnel: [w1123 State_Type_Definitions,_for_0.26g_versions_and_later_2."True Stop" ("Enum")] -> w1116
              tunnel: [w1126 w1143] -> w1109
              tunnel: [State_Type_Definitions,_for_0.26g_versions_and_later_2."Idle" ("Enum") State_Type_Definitions,_for_0.26g_versions_and_later_2."Shutdown" ("Enum")] -> w1108
              tunnel: w1110 -> [w1117 _]
              tunnel: w1115 -> [w1122 w1140]
              tunnel: w1106 -> [w1121 _]
              frame "None", Default {
                # ">> Is time up? >>"
                # "Determines if object is in range to pick up"
                # ">> Manual override >>"
                n407 = case shown="True" w1121 {
                  tunnel: [w1130 w1136] -> w1126
                  tunnel: w1122 -> [w1128 w1134]
                  frame False {
                    n408 = for {
                      tunnel: string[] ["CLOSE CLAW", "START TIMER"] ("element") -> [w1131] mode=indexing
                      shift-right: [w1133] -> w1130
                      shift-left: w1128 -> [w1132]
                      n409 = Enqueue Element(queue=w1132, element=w1131) -> (queue out=w1133:refnum<queue>)  [unwired: 2 in, 2 out]
                    }
                  }
                  frame True {
                    n410 = for {
                      shift-right: [w1138] -> w1136
                      shift-left: w1134 -> [w1139]
                      tunnel: string[] ["READ STEPPER VALUES", "", ""] -> [w1137] mode=indexing
                      n411 = Enqueue Element(queue=w1139, element=w1137) -> (queue out=w1138:refnum<queue>)  [unwired: 2 in, 2 out]
                    }
                  }
                }
                n412 = Or(x=w1121, y=w1117) -> (x .or. y?=w1124:bool)
                n413 = Select(t=State_Type_Definitions,_for_0.26g_versions_and_later_2."True Stop" ("Enum"), s=w1117, f=State_Type_Definitions,_for_0.26g_versions_and_later_2."Task 5H: RAISE ARM" ("Enum")) -> (s? t:f=w1119:T6)
                n414 = Select(t=w1119, s=w1124, f=State_Type_Definitions,_for_0.26g_versions_and_later_2."Task 5G: CLOSE CLAW" ("Enum")) -> (s? t:f=w1123:T6)
              }
              frame "Exit" {
                n415 = for {
                  shift-right: [w1146] -> w1143
                  shift-left: w1140 -> [w1147]
                  tunnel: string[] ["STOP", "RESET ENCODERS", "RESET YAW", "ARDUINO MODE 0"] -> [w1145] mode=indexing
                  n416 = Enqueue Element(queue=w1147, element=w1145) -> (queue out=w1146:refnum<queue>)  [unwired: 2 in, 2 out]
                }
              }
            }
          }
          frame 23 {
            # ">>> yStepper command>>>"
            # ">> Manual override >>"
            n417 = Dequeue Element(queue=w1157, timeout in ms (-1)=w1156, error in (no error)=w1158) -> (element=w1155:T7)  [unwired: 3 out]
            n418 = Equal?(x=w1154, y=u8 60) -> (x = y?=w1152:bool)
            n419 = case shown="\"None\", Default" w1155 {
              tunnel: [w1168 State_Type_Definitions,_for_0.26g_versions_and_later_2."True Stop" ("Enum")] -> w1159
              tunnel: [w1171 w1188] -> w1160
              tunnel: [State_Type_Definitions,_for_0.26g_versions_and_later_2."Idle" ("Enum") State_Type_Definitions,_for_0.26g_versions_and_later_2."Shutdown" ("Enum")] -> w1161
              tunnel: w1152 -> [w1167 _]
              tunnel: w1151 -> [w1166 _]
              tunnel: w1150 -> [w1162 w1185]
              frame "None", Default {
                # "Stays in Task 5_A until stepper reaches desired \nheight"
                # "T: Go back to idle, F: Continue with task\""
                # ">> Manual override >>"
                n420 = case shown="False" w1167 {
                  tunnel: [w1175 w1181] -> w1171
                  tunnel: w1162 -> [w1173 w1179]
                  frame False {
                    n421 = for {
                      tunnel: string[] ["Z STEPPER CAM HEIGHT", "READ STEPPER VALUES"] ("element") -> [w1176] mode=indexing
                      shift-right: [w1178] -> w1175
                      shift-left: w1173 -> [w1177]
                      n422 = Enqueue Element(queue=w1177, element=w1176) -> (queue out=w1178:refnum<queue>)  [unwired: 2 in, 2 out]
                    }
                  }
                  frame True {
                    n423 = for {
                      shift-right: [w1183] -> w1181
                      shift-left: w1179 -> [w1184]
                      tunnel: string[] ["ARDUINO - ULTRASONIC", "READ ULTRASONIC", ""] -> [w1182] mode=indexing
                      n424 = Enqueue Element(queue=w1184, element=w1182) -> (queue out=w1183:refnum<queue>)  [unwired: 2 in, 2 out]
                    }
                  }
                }
                n425 = Or(x=w1167, y=w1166) -> (x .or. y?=w1169:bool)
                n426 = Select(t=State_Type_Definitions,_for_0.26g_versions_and_later_2."True Stop" ("Enum"), s=w1166, f=State_Type_Definitions,_for_0.26g_versions_and_later_2."True Stop" ("Enum")) -> (s? t:f=w1163:T6)
                n427 = Select(t=w1163, s=w1169, f=State_Type_Definitions,_for_0.26g_versions_and_later_2."Task 5H: RAISE ARM" ("Enum")) -> (s? t:f=w1168:T6)
              }
              frame "Exit" {
                n428 = for {
                  shift-right: [w1191] -> w1188
                  shift-left: w1185 -> [w1192]
                  tunnel: string[] ["STOP", "RESET ENCODERS", "RESET YAW", "ARDUINO MODE 0"] -> [w1190] mode=indexing
                  n429 = Enqueue Element(queue=w1192, element=w1190) -> (queue out=w1191:refnum<queue>)  [unwired: 2 in, 2 out]
                }
              }
            }
          }
          frame 24 {
            # ">>> yStepper command>>>"
            n430 = Dequeue Element(queue=w1201, timeout in ms (-1)=w1200, error in (no error)=w1199) -> (element=w1206:T7)  [unwired: 3 out]
            n431 = Equal?(x=w1197, y=u8 60) -> (x = y?=w1196:bool)
            n432 = case shown="\"None\", Default" w1206 {
              tunnel: [w1213 State_Type_Definitions,_for_0.26g_versions_and_later_2."True Stop" ("Enum")] -> w1204
              tunnel: [w1212 w1230] -> w1203
              tunnel: [State_Type_Definitions,_for_0.26g_versions_and_later_2."Idle" ("Enum") State_Type_Definitions,_for_0.26g_versions_and_later_2."Shutdown" ("Enum")] -> w1205
              tunnel: w1202 -> [w1208 _]
              tunnel: w1198 -> [w1210 _]
              tunnel: w1196 -> [w1207 _]
              frame "None", Default {
                n433 = case shown="False" w1207 {
                  tunnel: [w1218 w1224] -> w1212
                  tunnel: w1210 -> [w1216 w1222]
                  frame False {
                    n434 = for {
                      tunnel: string[] ["Z STEPPER CAM HEIGHT", "READ STEPPER VALUES"] ("element") -> [w1219] mode=indexing
                      shift-right: [w1221] -> w1218
                      shift-left: w1216 -> [w1220]
                      n435 = Enqueue Element(queue=w1220, element=w1219) -> (queue out=w1221:refnum<queue>)  [unwired: 2 in, 2 out]
                    }
                  }
                  frame True {
                    n436 = for {
                      shift-right: [w1226] -> w1224
                      shift-left: w1222 -> [w1227]
                      tunnel: string[] ["CAM ACQ", "OPEN LOG CAM"] -> [w1225] mode=indexing
                      n437 = Enqueue Element(queue=w1227, element=w1225) -> (queue out=w1226:refnum<queue>)  [unwired: 2 in, 2 out]
                    }
                  }
                }
                n438 = Or(x=w1207, y=w1208) -> (x .or. y?=w1209:bool)
                n439 = Select(t=State_Type_Definitions,_for_0.26g_versions_and_later_2."Task 6_B" ("Enum"), s=w1209, f=State_Type_Definitions,_for_0.26g_versions_and_later_2."Task 6_A" ("Enum")) -> (s? t:f=w1213:T6)
              }
              frame "Exit" {
                n440 = for {
                  shift-right: [w1233] -> w1230
                  shift-left: _ -> [w1234]
                  tunnel: string[] ["STOP", "RESET ENCODERS", "RESET YAW", "ARDUINO MODE 0"] -> [w1232] mode=indexing
                  n441 = Enqueue Element(queue=w1234, element=w1232) -> (queue out=w1233:refnum<queue>)  [unwired: 2 in, 2 out]
                }
              }
            }
          }
          frame 25 {
            # ">>> yStepper command>>>"
            n442 = Dequeue Element(queue=w1245, timeout in ms (-1)=w1243, error in (no error)=w1244) -> (element=w1242:T7)  [unwired: 3 out]
            n443 = case shown="\"None\", Default" w1242 {
              tunnel: [w1252 State_Type_Definitions,_for_0.26g_versions_and_later_2."True Stop" ("Enum")] -> w1238
              tunnel: [w1251 w1270] -> w1246
              tunnel: [State_Type_Definitions,_for_0.26g_versions_and_later_2."Idle" ("Enum") State_Type_Definitions,_for_0.26g_versions_and_later_2."Shutdown" ("Enum")] -> w1239
              tunnel: w1241 -> [w1247 _]
              tunnel: w1240 -> [w1249 _]
              tunnel: w1237 -> [w1248 w1267]
              frame "None", Default {
                # ">> Manual override >>"
                n444 = case shown="True" w1249 {
                  tunnel: [w1257 w1263] -> w1251
                  tunnel: w1248 -> [w1256 w1261]
                  frame False {
                    n445 = for {
                      shift-right: [w1260] -> w1257
                      shift-left: w1256 -> [w1259]
                      tunnel: string[] ["CAM ACQ", "PROCESS IMAGE", "OPEN CLAW"] -> [w1258] mode=indexing
                      n446 = Enqueue Element(queue=w1259, element=w1258) -> (queue out=w1260:refnum<queue>)  [unwired: 2 in, 2 out]
                    }
                  }
                  frame True {
                    n447 = for {
                      shift-right: [w1265] -> w1263
                      shift-left: w1261 -> [w1266]
                      tunnel: string[] ["CAM ACQ", "PROCESS IMAGE", "CLOSE CLAW"] -> [w1264] mode=indexing
                      n448 = Enqueue Element(queue=w1266, element=w1264) -> (queue out=w1265:refnum<queue>)  [unwired: 2 in, 2 out]
                    }
                  }
                }
                n449 = Select(t=State_Type_Definitions,_for_0.26g_versions_and_later_2."True Stop" ("Enum"), s=w1247, f=State_Type_Definitions,_for_0.26g_versions_and_later_2."Task 6_B" ("Enum")) -> (s? t:f=w1252:T6)
              }
              frame "Exit" {
                # ">> State after true stop >>"
                # ">> Goes to true stop >>"
                n450 = for {
                  shift-right: [w1273] -> w1270
                  shift-left: w1267 -> [w1274]
                  tunnel: string[] ["STOP", "RESET ENCODERS", "RESET YAW", ""] -> [w1272] mode=indexing
                  n451 = Enqueue Element(queue=w1274, element=w1272) -> (queue out=w1273:refnum<queue>)  [unwired: 2 in, 2 out]
                }
              }
            }
          }
          frame 26 {
          }
          frame 27 {
            # ">>> yStepper command>>>"
            # ">> Manual override >>"
            n452 = Dequeue Element(queue=w1289, timeout in ms (-1)=w1288, error in (no error)=w1290) -> (element=w1287:T7)  [unwired: 3 out]
            n453 = Equal?(x=w1286, y=u8 60) -> (x = y?=w1284:bool)
            n454 = case shown="\"None\", Default" w1287 {
              tunnel: [w1300 State_Type_Definitions,_for_0.26g_versions_and_later_2."True Stop" ("Enum")] -> w1291
              tunnel: [w1303 w1320] -> w1292
              tunnel: [State_Type_Definitions,_for_0.26g_versions_and_later_2."Idle" ("Enum") State_Type_Definitions,_for_0.26g_versions_and_later_2."Shutdown" ("Enum")] -> w1293
              tunnel: w1284 -> [w1299 _]
              tunnel: w1283 -> [w1298 _]
              tunnel: w1282 -> [w1294 w1317]
              frame "None", Default {
                # "Stays in Task 5_A until stepper reaches desired \nheight"
                # "T: Go back to idle, F: Continue with task\""
                # ">> Manual override >>"
                n455 = case shown="True" w1299 {
                  tunnel: [w1307 w1313] -> w1303
                  tunnel: w1294 -> [w1305 w1311]
                  frame False {
                    n456 = for {
                      tunnel: string[] ["Z STEPPER CAM HEIGHT", "READ STEPPER VALUES"] ("element") -> [w1308] mode=indexing
                      shift-right: [w1310] -> w1307
                      shift-left: w1305 -> [w1309]
                      n457 = Enqueue Element(queue=w1309, element=w1308) -> (queue out=w1310:refnum<queue>)  [unwired: 2 in, 2 out]
                    }
                  }
                  frame True {
                    n458 = for {
                      shift-right: [w1315] -> w1313
                      shift-left: w1311 -> [w1316]
                      tunnel: string[] ["ARDUINO - ULTRASONIC", "READ ULTRASONIC", ""] -> [w1314] mode=indexing
                      n459 = Enqueue Element(queue=w1316, element=w1314) -> (queue out=w1315:refnum<queue>)  [unwired: 2 in, 2 out]
                    }
                  }
                }
                n460 = Or(x=w1299, y=w1298) -> (x .or. y?=w1301:bool)
                n461 = Select(t=State_Type_Definitions,_for_0.26g_versions_and_later_2."True Stop" ("Enum"), s=w1298, f=State_Type_Definitions,_for_0.26g_versions_and_later_2."Task 8B: MOVE TO BOX" ("Enum")) -> (s? t:f=w1295:T6)
                n462 = Select(t=w1295, s=w1301, f=State_Type_Definitions,_for_0.26g_versions_and_later_2."Task 8A: RAISE ARM" ("Enum")) -> (s? t:f=w1300:T6)
              }
              frame "Exit" {
                n463 = for {
                  shift-right: [w1323] -> w1320
                  shift-left: w1317 -> [w1324]
                  tunnel: string[] ["STOP", "RESET ENCODERS", "RESET YAW", "ARDUINO MODE 0"] -> [w1322] mode=indexing
                  n464 = Enqueue Element(queue=w1324, element=w1322) -> (queue out=w1323:refnum<queue>)  [unwired: 2 in, 2 out]
                }
              }
            }
          }
          frame 28 {
            w1331 = u8 20 ("y")
            # ">>> yStepper command>>>"
            n465 = Less?(x=w1328, y=w1331) -> (x < y?=w1329:bool)
            n466 = Dequeue Element(queue=w1335, timeout in ms (-1)=w1334, error in (no error)=w1336) -> (element=w1333:T7)  [unwired: 3 out]
            n467 = Less?(x=w1327, y=w1331) -> (x < y?=w1330:bool)
            n468 = And(x=w1330, y=w1329) -> (x .and. y?=w1326:bool)
            n469 = case shown="\"None\", Default" w1333 {
              tunnel: [w1348 State_Type_Definitions,_for_0.26g_versions_and_later_2."True Stop" ("Enum")] -> w1338
              tunnel: [w1351 w1368] -> w1337
              tunnel: [State_Type_Definitions,_for_0.26g_versions_and_later_2."Idle" ("Enum") State_Type_Definitions,_for_0.26g_versions_and_later_2."Shutdown" ("Enum")] -> w1339
              tunnel: w1341 -> [w1347 _]
              tunnel: w1340 -> [w1343 w1365]
              tunnel: w1326 -> [w1342 _]
              frame "None", Default {
                # "Stays in Task 5_B to capture image over 5 seconds"
                # "T: Go back to idle, F: Continue with task\""
                # ">> Manual override >>"
                n470 = case shown="True" w1342 {
                  tunnel: [w1355 w1361] -> w1351
                  tunnel: w1343 -> [w1353 w1359]
                  frame False {
                    n471 = for {
                      tunnel: string[] ["FORWARD", "READ ULTRASONIC", "READ NAVX"] ("element") -> [w1356] mode=indexing
                      shift-right: [w1358] -> w1355
                      shift-left: w1353 -> [w1357]
                      n472 = Enqueue Element(queue=w1357, element=w1356) -> (queue out=w1358:refnum<queue>)  [unwired: 2 in, 2 out]
                    }
                  }
                  frame True {
                    n473 = for {
                      shift-right: [w1363] -> w1361
                      shift-left: w1359 -> [w1364]
                      tunnel: string[] ["STOP", "RESET ENCODERS", "OPEN LOG CAM", "SET TIMER 2", "OPEN IMAQ REF"] -> [w1362] mode=indexing
                      n474 = Enqueue Element(queue=w1364, element=w1362) -> (queue out=w1363:refnum<queue>)  [unwired: 2 in, 2 out]
                    }
                  }
                }
                n475 = Or(x=w1342, y=w1347) -> (x .or. y?=w1349:bool)
                n476 = Select(t=State_Type_Definitions,_for_0.26g_versions_and_later_2."True Stop" ("Enum"), s=w1347, f=State_Type_Definitions,_for_0.26g_versions_and_later_2."Task 8C: CAM BURST" ("Enum")) -> (s? t:f=w1344:T6)
                n477 = Select(t=w1344, s=w1349, f=State_Type_Definitions,_for_0.26g_versions_and_later_2."Task 8B: MOVE TO BOX" ("Enum")) -> (s? t:f=w1348:T6)
              }
              frame "Exit" {
                n478 = for {
                  shift-right: [w1371] -> w1368
                  shift-left: w1365 -> [w1372]
                  tunnel: string[] ["STOP", "RESET ENCODERS", "RESET YAW", "ARDUINO MODE 0"] -> [w1370] mode=indexing
                  n479 = Enqueue Element(queue=w1372, element=w1370) -> (queue out=w1371:refnum<queue>)  [unwired: 2 in, 2 out]
                }
              }
            }
          }
          frame 29 {
            # ">>> Motor control cluster >>>"
            # ">>> yStepper command>>>"
            # ">> Manual override >>"
            n480 = Dequeue Element(queue=w1382, timeout in ms (-1)=w1381, error in (no error)=w1380) -> (element=w1379:T7)  [unwired: 3 out]
            n481 = case shown="\"None\", Default" w1379 {
              tunnel: [w1391 State_Type_Definitions,_for_0.26g_versions_and_later_2."True Stop" ("Enum")] -> w1384
              tunnel: [w1394 w1411] -> w1377
              tunnel: [State_Type_Definitions,_for_0.26g_versions_and_later_2."Idle" ("Enum") State_Type_Definitions,_for_0.26g_versions_and_later_2."Shutdown" ("Enum")] -> w1376
              tunnel: w1378 -> [w1385 _]
              tunnel: w1383 -> [w1390 w1408]
              tunnel: w1374 -> [w1389 _]
              frame "None", Default {
                # ">> Is time up? >>"
                # "Determines if object is in range to pick up"
                # ">> Manual override >>"
                n482 = case shown="True" w1389 {
                  tunnel: [w1398 w1404] -> w1394
                  tunnel: w1390 -> [w1396 w1402]
                  frame False {
                    n483 = for {
                      tunnel: string[] ["CAM ACQ", "START TIMER"] ("element") -> [w1399] mode=indexing
                      shift-right: [w1401] -> w1398
                      shift-left: w1396 -> [w1400]
                      n484 = Enqueue Element(queue=w1400, element=w1399) -> (queue out=w1401:refnum<queue>)  [unwired: 2 in, 2 out]
                    }
                  }
                  frame True {
                    n485 = for {
                      shift-right: [w1406] -> w1404
                      shift-left: w1402 -> [w1407]
                      tunnel: string[] ["CAM CLOSE", "PROCESS IMAGE", "SET TIMER 5"] -> [w1405] mode=indexing
                      n486 = Enqueue Element(queue=w1407, element=w1405) -> (queue out=w1406:refnum<queue>)  [unwired: 2 in, 2 out]
                    }
                  }
                }
                n487 = Or(x=w1389, y=w1385) -> (x .or. y?=w1392:bool)
                n488 = Select(t=State_Type_Definitions,_for_0.26g_versions_and_later_2."True Stop" ("Enum"), s=w1385, f=State_Type_Definitions,_for_0.26g_versions_and_later_2."Task 8D: PROCESS IMAGE" ("Enum")) -> (s? t:f=w1387:T6)
                n489 = Select(t=w1387, s=w1392, f=State_Type_Definitions,_for_0.26g_versions_and_later_2."Task 8C: CAM BURST" ("Enum")) -> (s? t:f=w1391:T6)
              }
              frame "Exit" {
                n490 = for {
                  shift-right: [w1414] -> w1411
                  shift-left: w1408 -> [w1415]
                  tunnel: string[] ["STOP", "RESET ENCODERS", "RESET YAW", "ARDUINO MODE 0"] -> [w1413] mode=indexing
                  n491 = Enqueue Element(queue=w1415, element=w1413) -> (queue out=w1414:refnum<queue>)  [unwired: 2 in, 2 out]
                }
              }
            }
          }
          frame 30 {
            # ">>> yStepper command>>>"
            n492 = Dequeue Element(queue=w1422, timeout in ms (-1)=w1421, error in (no error)=w1420) -> (element=w1419:T7)  [unwired: 3 out]
            n493 = case shown="\"None\", Default" w1419 {
              tunnel: [w1434 State_Type_Definitions,_for_0.26g_versions_and_later_2."True Stop" ("Enum")] -> w1426
              tunnel: [w1437 w1454] -> w1425
              tunnel: [State_Type_Definitions,_for_0.26g_versions_and_later_2."Idle" ("Enum") State_Type_Definitions,_for_0.26g_versions_and_later_2."Shutdown" ("Enum")] -> w1427
              tunnel: w1423 -> [w1433 _]
              tunnel: w1424 -> [w1429 w1451]
              tunnel: w1417 -> [w1428 _]
              frame "None", Default {
                # ">> T: Breaks out of state loop; F: Stays in loop>>"
                # ">> Manual override >>"
                # ">> Checks if time is up>>"
                # "Stays in Task 5D until the object is detected"
                # "T: Go back to idle, F: Continue with task\""
                # ">> Manual override >>"
                n494 = case shown="False" w1428 {
                  tunnel: [w1441 w1447] -> w1437
                  tunnel: w1429 -> [w1439 w1445]
                  frame False {
                    n495 = for {
                      tunnel: string[] ["START TIMER", "PROCESS IMAGE", ""] ("element") -> [w1442] mode=indexing
                      shift-right: [w1444] -> w1441
                      shift-left: w1439 -> [w1443]
                      n496 = Enqueue Element(queue=w1443, element=w1442) -> (queue out=w1444:refnum<queue>)  [unwired: 2 in, 2 out]
                    }
                  }
                  frame True {
                    n497 = for {
                      shift-right: [w1449] -> w1447
                      shift-left: w1445 -> [w1450]
                      tunnel: string[] ["RESET ENCODERS", "", ""] -> [w1448] mode=indexing
                      n498 = Enqueue Element(queue=w1450, element=w1448) -> (queue out=w1449:refnum<queue>)  [unwired: 2 in, 2 out]
                    }
                  }
                }
                n499 = Or(x=w1428, y=w1433) -> (x .or. y?=w1435:bool)
                n500 = Select(t=State_Type_Definitions,_for_0.26g_versions_and_later_2."True Stop" ("Enum"), s=w1433, f=State_Type_Definitions,_for_0.26g_versions_and_later_2."Task 8E: ROBOT ADJUST" ("Enum")) -> (s? t:f=w1430:T6)
                n501 = Select(t=w1430, s=w1435, f=State_Type_Definitions,_for_0.26g_versions_and_later_2."Task 8D: PROCESS IMAGE" ("Enum")) -> (s? t:f=w1434:T6)
              }
              frame "Exit" {
                n502 = for {
                  shift-right: [w1457] -> w1454
                  shift-left: w1451 -> [w1458]
                  tunnel: string[] ["STOP", "RESET ENCODERS", "RESET YAW", "ARDUINO MODE 0"] -> [w1456] mode=indexing
                  n503 = Enqueue Element(queue=w1458, element=w1456) -> (queue out=w1457:refnum<queue>)  [unwired: 2 in, 2 out]
                }
              }
            }
          }
          frame 31 {
            # ">>> Motor control cluster >>>"
            # ">>> yStepper command>>>"
            n504 = Dequeue Element(queue=w1474, timeout in ms (-1)=w1473, error in (no error)=w1472) -> (element=w1471:T7)  [unwired: 3 out]
            n505 = Subtract(x=w1469, y=300.0) -> (x-y=w1467:dbl)
            "x-y" <- w1467
            n506 = formula code="if (error < -80 && error >-300){\ndistance = -20;\nxSpeed = -30;\n}\n\nelse if (error <= 61&&error >= -80){\ndistance = -15;\nxSpeed = -30;\n}\n\nelse if (error <= -26 && error >= -60){\ndistance = -10;\nxSpeed = -30;\n}\n\nelse if (error >= -25 && error <= 25){\ndistance = 0;\nxSpeed = 0;\n}\n\nelse if (error >= 51 && error <= 80){\ndistance = 10;\nxSpeed = 30;\n}\n\nelse if (error >= 81 && error <= 100){\ndistance = 15;\nxSpeed = 30;\n}\n\nelse if (error >= 101 && error <= 120){\ndistance = 20;\nxSpeed = 30;\n}\n\nelse if (error >= 121 && error <= 150){\ndistance = 25;\nxSpeed = 30;\n}\n\nelse if (error < 250){\ndistance = 30;\nxSpeed = 30;\n}\n\nelse{\ndistance = 0;\nxSpeed = 0;\n}"("error"=w1467) -> ("distance"=w1462:dbl, "xSpeed"=w1464:dbl)
            n507 = formula code="if (target > 0){\nif (current  >= target)\noutput = 1;\n}\n\nelse if (target == 0){\nif (current == target)\noutput = 1;\n}\n\nelse if (target < 0){\nif (current <= target)\noutput = 1;\n}\n\nelse\noutput = 0;"("target"=w1462, "current"=w1463) -> ("output"=w1461:dbl)
            n508 = Bundle By Name(cluster=w1466, "xSpeed"=w1464) -> (w1465:T9)
            n509 = Equal?(x=w1461, y=1.0) -> (x = y?=w1459:bool)
            n510 = case shown="\"None\", Default" w1471 {
              tunnel: [w1486 State_Type_Definitions,_for_0.26g_versions_and_later_2."True Stop" ("Enum")] -> w1478
              tunnel: [w1489 w1506] -> w1477
              tunnel: [State_Type_Definitions,_for_0.26g_versions_and_later_2."Idle" ("Enum") State_Type_Definitions,_for_0.26g_versions_and_later_2."Shutdown" ("Enum")] -> w1479
              tunnel: w1475 -> [w1485 _]
              tunnel: w1476 -> [w1481 w1503]
              tunnel: w1459 -> [w1480 _]
              frame "None", Default {
                # ">> T: Breaks out of state loop; F: Stays in loop>>"
                # ">> Manual override >>"
                # ">> Checks if time is up>>"
                # "Stays in Task 5D until the object is detected"
                # "T: Go back to idle, F: Continue with task\""
                # ">> Manual override >>"
                n511 = case shown="False" w1480 {
                  tunnel: [w1493 w1499] -> w1489
                  tunnel: w1481 -> [w1491 w1497]
                  frame False {
                    n512 = for {
                      tunnel: string[] ["X AXIS - SLOW", "READ ENCODERS", "READ NAVX"] ("element") -> [w1494] mode=indexing
                      shift-right: [w1496] -> w1493
                      shift-left: w1491 -> [w1495]
                      n513 = Enqueue Element(queue=w1495, element=w1494) -> (queue out=w1496:refnum<queue>)  [unwired: 2 in, 2 out]
                    }
                  }
                  frame True {
                    n514 = for {
                      shift-right: [w1501] -> w1499
                      shift-left: w1497 -> [w1502]
                      tunnel: string[] ["SET TIMER 2", "STOP", "READ STEPPER VALUES", ""] -> [w1500] mode=indexing
                      n515 = Enqueue Element(queue=w1502, element=w1500) -> (queue out=w1501:refnum<queue>)  [unwired: 2 in, 2 out]
                    }
                  }
                }
                n516 = Or(x=w1480, y=w1485) -> (x .or. y?=w1487:bool)
                n517 = Select(t=State_Type_Definitions,_for_0.26g_versions_and_later_2."True Stop" ("Enum"), s=w1485, f=State_Type_Definitions,_for_0.26g_versions_and_later_2."Task 8H: ARM ADJUST" ("Enum")) -> (s? t:f=w1482:T6)
                n518 = Select(t=w1482, s=w1487, f=State_Type_Definitions,_for_0.26g_versions_and_later_2."Task 8E: ROBOT ADJUST" ("Enum")) -> (s? t:f=w1486:T6)
              }
              frame "Exit" {
                n519 = for {
                  shift-right: [w1509] -> w1506
                  shift-left: w1503 -> [w1510]
                  tunnel: string[] ["STOP", "RESET ENCODERS", "RESET YAW", "ARDUINO MODE 0"] -> [w1508] mode=indexing
                  n520 = Enqueue Element(queue=w1510, element=w1508) -> (queue out=w1509:refnum<queue>)  [unwired: 2 in, 2 out]
                }
              }
            }
          }
          frame 32 {
            # ">>> Motor control cluster >>>"
            # ">>> yStepper command>>>"
            # ">> Manual override >>"
            n521 = Dequeue Element(queue=w1520, timeout in ms (-1)=w1519, error in (no error)=w1518) -> (element=w1517:T7)  [unwired: 3 out]
            n522 = case shown="\"None\", Default" w1517 {
              tunnel: [w1529 State_Type_Definitions,_for_0.26g_versions_and_later_2."True Stop" ("Enum")] -> w1522
              tunnel: [w1532 w1549] -> w1515
              tunnel: [State_Type_Definitions,_for_0.26g_versions_and_later_2."Idle" ("Enum") State_Type_Definitions,_for_0.26g_versions_and_later_2."Shutdown" ("Enum")] -> w1514
              tunnel: w1516 -> [w1523 _]
              tunnel: w1521 -> [w1528 w1546]
              tunnel: w1512 -> [w1527 _]
              frame "None", Default {
                # ">> Is time up? >>"
                # "Determines if object is in range to pick up"
                # ">> Manual override >>"
                n523 = case shown="True" w1527 {
                  tunnel: [w1536 w1542] -> w1532
                  tunnel: w1528 -> [w1534 w1540]
                  frame False {
                    n524 = for {
                      tunnel: string[] ["CAM ACQ", "START TIMER"] ("element") -> [w1537] mode=indexing
                      shift-right: [w1539] -> w1536
                      shift-left: w1534 -> [w1538]
                      n525 = Enqueue Element(queue=w1538, element=w1537) -> (queue out=w1539:refnum<queue>)  [unwired: 2 in, 2 out]
                    }
                  }
                  frame True {
                    n526 = for {
                      shift-right: [w1544] -> w1542
                      shift-left: w1540 -> [w1545]
                      tunnel: string[] ["CAM CLOSE", "PROCESS IMAGE", "SET TIMER 3"] -> [w1543] mode=indexing
                      n527 = Enqueue Element(queue=w1545, element=w1543) -> (queue out=w1544:refnum<queue>)  [unwired: 2 in, 2 out]
                    }
                  }
                }
                n528 = Or(x=w1527, y=w1523) -> (x .or. y?=w1530:bool)
                n529 = Select(t=State_Type_Definitions,_for_0.26g_versions_and_later_2."True Stop" ("Enum"), s=w1523, f=State_Type_Definitions,_for_0.26g_versions_and_later_2."Task 8G: PROCESS IMAGE 2" ("Enum")) -> (s? t:f=w1525:T6)
                n530 = Select(t=w1525, s=w1530, f=State_Type_Definitions,_for_0.26g_versions_and_later_2."Task 8F: CAM BURST 2" ("Enum")) -> (s? t:f=w1529:T6)
              }
              frame "Exit" {
                n531 = for {
                  shift-right: [w1552] -> w1549
                  shift-left: w1546 -> [w1553]
                  tunnel: string[] ["STOP", "RESET ENCODERS", "RESET YAW", "ARDUINO MODE 0"] -> [w1551] mode=indexing
                  n532 = Enqueue Element(queue=w1553, element=w1551) -> (queue out=w1552:refnum<queue>)  [unwired: 2 in, 2 out]
                }
              }
            }
          }
          frame 33 {
            # ">>> yStepper command>>>"
            n533 = Dequeue Element(queue=w1560, timeout in ms (-1)=w1559, error in (no error)=w1558) -> (element=w1557:T7)  [unwired: 3 out]
            n534 = case shown="\"None\", Default" w1557 {
              tunnel: [w1572 State_Type_Definitions,_for_0.26g_versions_and_later_2."True Stop" ("Enum")] -> w1564
              tunnel: [w1575 w1592] -> w1563
              tunnel: [State_Type_Definitions,_for_0.26g_versions_and_later_2."Idle" ("Enum") State_Type_Definitions,_for_0.26g_versions_and_later_2."Shutdown" ("Enum")] -> w1565
              tunnel: w1561 -> [w1571 _]
              tunnel: w1562 -> [w1567 w1589]
              tunnel: w1555 -> [w1566 _]
              frame "None", Default {
                # ">> T: Breaks out of state loop; F: Stays in loop>>"
                # ">> Manual override >>"
                # ">> Checks if time is up>>"
                # "Stays in Task 5D until the object is detected"
                # "T: Go back to idle, F: Continue with task\""
                # ">> Manual override >>"
                n535 = case shown="False" w1566 {
                  tunnel: [w1579 w1585] -> w1575
                  tunnel: w1567 -> [w1577 w1583]
                  frame False {
                    n536 = for {
                      tunnel: string[] ["START TIMER", "PROCESS IMAGE", ""] ("element") -> [w1580] mode=indexing
                      shift-right: [w1582] -> w1579
                      shift-left: w1577 -> [w1581]
                      n537 = Enqueue Element(queue=w1581, element=w1580) -> (queue out=w1582:refnum<queue>)  [unwired: 2 in, 2 out]
                    }
                  }
                  frame True {
                    n538 = for {
                      shift-right: [w1587] -> w1585
                      shift-left: w1583 -> [w1588]
                      tunnel: string[] ["READ STEPPER VALUES", "Y STEPPER CONTROL", ""] -> [w1586] mode=indexing
                      n539 = Enqueue Element(queue=w1588, element=w1586) -> (queue out=w1587:refnum<queue>)  [unwired: 2 in, 2 out]
                    }
                  }
                }
                n540 = Or(x=w1566, y=w1571) -> (x .or. y?=w1573:bool)
                n541 = Select(t=State_Type_Definitions,_for_0.26g_versions_and_later_2."True Stop" ("Enum"), s=w1571, f=State_Type_Definitions,_for_0.26g_versions_and_later_2."Task 8H: ARM ADJUST" ("Enum")) -> (s? t:f=w1568:T6)
                n542 = Select(t=w1568, s=w1573, f=State_Type_Definitions,_for_0.26g_versions_and_later_2."Task 8G: PROCESS IMAGE 2" ("Enum")) -> (s? t:f=w1572:T6)
              }
              frame "Exit" {
                n543 = for {
                  shift-right: [w1595] -> w1592
                  shift-left: w1589 -> [w1596]
                  tunnel: string[] ["STOP", "RESET ENCODERS", "RESET YAW", "ARDUINO MODE 0"] -> [w1594] mode=indexing
                  n544 = Enqueue Element(queue=w1596, element=w1594) -> (queue out=w1595:refnum<queue>)  [unwired: 2 in, 2 out]
                }
              }
            }
          }
          frame 34 {
            # ">>> yStepper command>>>"
            n545 = Dequeue Element(queue=w1609, timeout in ms (-1)=w1610, error in (no error)=w1611) -> (element=w1613:T7)  [unwired: 3 out]
            n546 = formula code="if (pos <= 81)\ny = 40;\n\nelse if (pos >= 81 &&pos <= 120)\ny = 37;\n\nelse if (pos >= 121 && pos <= 140)\ny = 28;\n\nelse if (pos >= 141 && pos <= 170)\ny = 25;\n\nelse if (pos >= 171 &&pos <= 200) \ny = 20;\n\nelse if (pos >= 201&& pos <= 210)\ny = 15;\n\nelse if (pos >= 211 && pos <= 230)\ny = 10;\n\nelse if (pos >= 231 && pos <= 320)\ny = 8;\n\nelse if (pos > 320)\ny = 0;"("pos"=w1601) -> ("y"=w1604:dbl)
            n547 = To Unsigned Byte Integer(number=w1604) -> (unsigned 8bit integer=w1599:u8)
            n548 = Equal?(x=w1600, y=w1599) -> (x = y?=w1598:bool)
            n549 = case shown="\"None\", Default" w1613 {
              tunnel: [w1620 State_Type_Definitions,_for_0.26g_versions_and_later_2."True Stop" ("Enum")] -> w1607
              tunnel: [w1623 w1640] -> w1605
              tunnel: [State_Type_Definitions,_for_0.26g_versions_and_later_2."Idle" ("Enum") State_Type_Definitions,_for_0.26g_versions_and_later_2."Shutdown" ("Enum")] -> w1606
              tunnel: w1612 -> [w1619 _]
              tunnel: w1608 -> [w1615 w1637]
              tunnel: w1598 -> [w1614 _]
              frame "None", Default {
                # ">> T: Breaks out of state loop; F: Stays in loop>>"
                # ">> Manual override >>"
                # ">> Checks if time is up>>"
                # "Stays in Task 5D until the object is detected"
                # "T: Go back to idle, F: Continue with task\""
                # ">> Manual override >>"
                n550 = case shown="False" w1614 {
                  tunnel: [w1627 w1633] -> w1623
                  tunnel: w1615 -> [w1625 w1631]
                  frame False {
                    n551 = for {
                      tunnel: string[] ["READ STEPPER VALUES", "Y STEPPER CONTROL", ""] ("element") -> [w1628] mode=indexing
                      shift-right: [w1630] -> w1627
                      shift-left: w1625 -> [w1629]
                      n552 = Enqueue Element(queue=w1629, element=w1628) -> (queue out=w1630:refnum<queue>)  [unwired: 2 in, 2 out]
                    }
                  }
                  frame True {
                    n553 = for {
                      shift-right: [w1635] -> w1633
                      shift-left: w1631 -> [w1636]
                      tunnel: string[] ["DISPOSE BUFFERS", "READ STEPPER VALUES", ""] -> [w1634] mode=indexing
                      n554 = Enqueue Element(queue=w1636, element=w1634) -> (queue out=w1635:refnum<queue>)  [unwired: 2 in, 2 out]
                    }
                  }
                }
                n555 = Or(x=w1614, y=w1619) -> (x .or. y?=w1621:bool)
                n556 = Select(t=State_Type_Definitions,_for_0.26g_versions_and_later_2."True Stop" ("Enum"), s=w1619, f=State_Type_Definitions,_for_0.26g_versions_and_later_2."Task 8I: ARM GRAB HEIGHT" ("Enum")) -> (s? t:f=w1616:T6)
                n557 = Select(t=w1616, s=w1621, f=State_Type_Definitions,_for_0.26g_versions_and_later_2."Task 8H: ARM ADJUST" ("Enum")) -> (s? t:f=w1620:T6)
              }
              frame "Exit" {
                n558 = for {
                  shift-right: [w1643] -> w1640
                  shift-left: w1637 -> [w1644]
                  tunnel: string[] ["STOP", "RESET ENCODERS", "RESET YAW", "ARDUINO MODE 0"] -> [w1642] mode=indexing
                  n559 = Enqueue Element(queue=w1644, element=w1642) -> (queue out=w1643:refnum<queue>)  [unwired: 2 in, 2 out]
                }
              }
            }
            n560 = Bundle By Name(cluster=w1603, "yStepper desired"=w1599) -> (w1602:T11)
          }
          frame 35 {
            # ">>> Motor control cluster >>>"
            # ">>> yStepper command>>>"
            # ">> Manual override >>"
            n561 = Dequeue Element(queue=w1654, timeout in ms (-1)=w1653, error in (no error)=w1655) -> (element=w1652:T7)  [unwired: 3 out]
            n562 = Equal?(x=w1651, y=u8 1) -> (x = y?=w1649:bool)
            n563 = case shown="\"None\", Default" w1652 {
              tunnel: [w1665 State_Type_Definitions,_for_0.26g_versions_and_later_2."True Stop" ("Enum")] -> w1656
              tunnel: [w1668 w1685] -> w1657
              tunnel: [State_Type_Definitions,_for_0.26g_versions_and_later_2."Idle" ("Enum") State_Type_Definitions,_for_0.26g_versions_and_later_2."Shutdown" ("Enum")] -> w1658
              tunnel: w1649 -> [w1664 _]
              tunnel: w1648 -> [w1663 _]
              tunnel: w1647 -> [w1659 w1682]
              frame "None", Default {
                # "Stays in Task 5F until stepper reaches desired \nheight"
                # "T: Go back to idle, F: Continue with task\""
                # ">> Manual override >>"
                n564 = case shown="True" w1664 {
                  tunnel: [w1672 w1678] -> w1668
                  tunnel: w1659 -> [w1670 w1676]
                  frame False {
                    n565 = for {
                      tunnel: string[] ["Z STEPPER GRAB HEIGHT", "READ STEPPER VALUES"] ("element") -> [w1673] mode=indexing
                      shift-right: [w1675] -> w1672
                      shift-left: w1670 -> [w1674]
                      n566 = Enqueue Element(queue=w1674, element=w1673) -> (queue out=w1675:refnum<queue>)  [unwired: 2 in, 2 out]
                    }
                  }
                  frame True {
                    n567 = for {
                      shift-right: [w1680] -> w1678
                      shift-left: w1676 -> [w1681]
                      tunnel: string[] ["SET TIMER 2", "CLOSE CLAW", ""] -> [w1679] mode=indexing
                      n568 = Enqueue Element(queue=w1681, element=w1679) -> (queue out=w1680:refnum<queue>)  [unwired: 2 in, 2 out]
                    }
                  }
                }
                n569 = Or(x=w1664, y=w1663) -> (x .or. y?=w1666:bool)
                n570 = Select(t=State_Type_Definitions,_for_0.26g_versions_and_later_2."True Stop" ("Enum"), s=w1663, f=State_Type_Definitions,_for_0.26g_versions_and_later_2."Task 8J: CLOSE CLAW" ("Enum")) -> (s? t:f=w1660:T6)
                n571 = Select(t=w1660, s=w1666, f=State_Type_Definitions,_for_0.26g_versions_and_later_2."Task 8I: ARM GRAB HEIGHT" ("Enum")) -> (s? t:f=w1665:T6)
              }
              frame "Exit" {
                n572 = for {
                  shift-right: [w1688] -> w1685
                  shift-left: w1682 -> [w1689]
                  tunnel: string[] ["STOP", "RESET ENCODERS", "RESET YAW", "ARDUINO MODE 0"] -> [w1687] mode=indexing
                  n573 = Enqueue Element(queue=w1689, element=w1687) -> (queue out=w1688:refnum<queue>)  [unwired: 2 in, 2 out]
                }
              }
            }
          }
          frame 36 {
            # ">>> yStepper command>>>"
            # ">> Manual override >>"
            n574 = Dequeue Element(queue=w1699, timeout in ms (-1)=w1698, error in (no error)=w1697) -> (element=w1696:T7)  [unwired: 3 out]
            n575 = case shown="\"None\", Default" w1696 {
              tunnel: [w1708 State_Type_Definitions,_for_0.26g_versions_and_later_2."True Stop" ("Enum")] -> w1701
              tunnel: [w1711 w1728] -> w1694
              tunnel: [State_Type_Definitions,_for_0.26g_versions_and_later_2."Idle" ("Enum") State_Type_Definitions,_for_0.26g_versions_and_later_2."Shutdown" ("Enum")] -> w1693
              tunnel: w1695 -> [w1702 _]
              tunnel: w1700 -> [w1707 w1725]
              tunnel: w1691 -> [w1706 _]
              frame "None", Default {
                # ">> Is time up? >>"
                # "Determines if object is in range to pick up"
                # ">> Manual override >>"
                n576 = case shown="True" w1706 {
                  tunnel: [w1715 w1721] -> w1711
                  tunnel: w1707 -> [w1713 w1719]
                  frame False {
                    n577 = for {
                      tunnel: string[] ["CLOSE CLAW", "START TIMER"] ("element") -> [w1716] mode=indexing
                      shift-right: [w1718] -> w1715
                      shift-left: w1713 -> [w1717]
                      n578 = Enqueue Element(queue=w1717, element=w1716) -> (queue out=w1718:refnum<queue>)  [unwired: 2 in, 2 out]
                    }
                  }
                  frame True {
                    n579 = for {
                      shift-right: [w1723] -> w1721
                      shift-left: w1719 -> [w1724]
                      tunnel: string[] ["READ STEPPER VALUES", "", ""] -> [w1722] mode=indexing
                      n580 = Enqueue Element(queue=w1724, element=w1722) -> (queue out=w1723:refnum<queue>)  [unwired: 2 in, 2 out]
                    }
                  }
                }
                n581 = Or(x=w1706, y=w1702) -> (x .or. y?=w1709:bool)
                n582 = Select(t=State_Type_Definitions,_for_0.26g_versions_and_later_2."True Stop" ("Enum"), s=w1702, f=State_Type_Definitions,_for_0.26g_versions_and_later_2."Task 8K: RAISE MY SWORD" ("Enum")) -> (s? t:f=w1704:T6)
                n583 = Select(t=w1704, s=w1709, f=State_Type_Definitions,_for_0.26g_versions_and_later_2."Task 8J: CLOSE CLAW" ("Enum")) -> (s? t:f=w1708:T6)
              }
              frame "Exit" {
                n584 = for {
                  shift-right: [w1731] -> w1728
                  shift-left: w1725 -> [w1732]
                  tunnel: string[] ["STOP", "RESET ENCODERS", "RESET YAW", "ARDUINO MODE 0"] -> [w1730] mode=indexing
                  n585 = Enqueue Element(queue=w1732, element=w1730) -> (queue out=w1731:refnum<queue>)  [unwired: 2 in, 2 out]
                }
              }
            }
          }
          frame 37 {
            # ">>> yStepper command>>>"
            # ">> Manual override >>"
            n586 = Dequeue Element(queue=w1742, timeout in ms (-1)=w1741, error in (no error)=w1743) -> (element=w1740:T7)  [unwired: 3 out]
            n587 = Equal?(x=w1739, y=u8 60) -> (x = y?=w1737:bool)
            n588 = case shown="\"None\", Default" w1740 {
              tunnel: [w1753 State_Type_Definitions,_for_0.26g_versions_and_later_2."True Stop" ("Enum")] -> w1744
              tunnel: [w1756 w1773] -> w1745
              tunnel: [State_Type_Definitions,_for_0.26g_versions_and_later_2."Idle" ("Enum") State_Type_Definitions,_for_0.26g_versions_and_later_2."Shutdown" ("Enum")] -> w1746
              tunnel: w1737 -> [w1752 _]
              tunnel: w1736 -> [w1751 _]
              tunnel: w1735 -> [w1747 w1770]
              frame "None", Default {
                # "Stays in Task 5_A until stepper reaches desired \nheight"
                # "T: Go back to idle, F: Continue with task\""
                # ">> Manual override >>"
                n589 = case shown="True" w1752 {
                  tunnel: [w1760 w1766] -> w1756
                  tunnel: w1747 -> [w1758 w1764]
                  frame False {
                    n590 = for {
                      tunnel: string[] ["Z STEPPER CAM HEIGHT", "READ STEPPER VALUES"] ("element") -> [w1761] mode=indexing
                      shift-right: [w1763] -> w1760
                      shift-left: w1758 -> [w1762]
                      n591 = Enqueue Element(queue=w1762, element=w1761) -> (queue out=w1763:refnum<queue>)  [unwired: 2 in, 2 out]
                    }
                  }
                  frame True {
                    n592 = for {
                      shift-right: [w1768] -> w1766
                      shift-left: w1764 -> [w1769]
                      tunnel: string[] ["CAM CLOSE", "DISPOSE ALL BUFFERS", ""] -> [w1767] mode=indexing
                      n593 = Enqueue Element(queue=w1769, element=w1767) -> (queue out=w1768:refnum<queue>)  [unwired: 2 in, 2 out]
                    }
                  }
                }
                n594 = Or(x=w1752, y=w1751) -> (x .or. y?=w1754:bool)
                n595 = Select(t=State_Type_Definitions,_for_0.26g_versions_and_later_2."True Stop" ("Enum"), s=w1751, f=State_Type_Definitions,_for_0.26g_versions_and_later_2."True Stop" ("Enum")) -> (s? t:f=w1748:T6)
                n596 = Select(t=w1748, s=w1754, f=State_Type_Definitions,_for_0.26g_versions_and_later_2."Task 8K: RAISE MY SWORD" ("Enum")) -> (s? t:f=w1753:T6)
              }
              frame "Exit" {
                n597 = for {
                  shift-right: [w1776] -> w1773
                  shift-left: w1770 -> [w1777]
                  tunnel: string[] ["STOP", "RESET ENCODERS", "RESET YAW", "ARDUINO MODE 0"] -> [w1775] mode=indexing
                  n598 = Enqueue Element(queue=w1777, element=w1775) -> (queue out=w1776:refnum<queue>)  [unwired: 2 in, 2 out]
                }
              }
            }
          }
          frame 38 {
            # ">> Stepper height reeached >>"
            # ">>> yStepper command>>>"
            # ">> Manual override >>"
            n599 = Dequeue Element(queue=w1788, timeout in ms (-1)=w1783, error in (no error)=w1787) -> (element=w1791:T7)  [unwired: 3 out]
            n600 = Equal?(x=w1785, y=u8 40) -> (x = y?=w1789:bool)
            n601 = case shown="\"None\", Default" w1791 {
              tunnel: [w1802 State_Type_Definitions,_for_0.26g_versions_and_later_2."True Stop" ("Enum")] -> w1781
              tunnel: [w1800 w1817] -> w1780
              tunnel: w1784 -> [w1799 _]
              tunnel: w1786 -> [w1793 _]
              tunnel: [State_Type_Definitions,_for_0.26g_versions_and_later_2."Idle" ("Enum") State_Type_Definitions,_for_0.26g_versions_and_later_2."Shutdown" ("Enum")] -> w1782
              tunnel: w1789 -> [w1792 _]
              frame "None", Default {
                # ">> WIill proceed to part ii if not manual override >>"
                # ">>If ENABLE or Trigger is set to true>>"
                n602 = Or(x=w1792, y=w1793) -> (x .or. y?=w1794:bool)
                n603 = case shown="False" w1792 {
                  tunnel: [w1805 w1811] -> w1800
                  tunnel: w1799 -> [w1804 w1810]
                  frame False {
                    n604 = for {
                      shift-right: [w1807] -> w1805
                      shift-left: w1804 -> [w1808]
                      tunnel: string[] ["Z STEPPER BOX HEIGHT", "READ STEPPER VALUES"] ("element") -> [w1806] mode=indexing
                      n605 = Enqueue Element(queue=w1808, element=w1806) -> (queue out=w1807:refnum<queue>)  [unwired: 2 in, 2 out]
                    }
                  }
                  frame True {
                    n606 = for {
                      shift-right: [w1813] -> w1811
                      shift-left: w1810 -> [w1814]
                      tunnel: string[] ["ARDUINO - ULTRASONIC", "READ ULTRASONIC", "", "", "", ""] -> [w1812] mode=indexing
                      n607 = Enqueue Element(queue=w1814, element=w1812) -> (queue out=w1813:refnum<queue>)  [unwired: 2 in, 2 out]
                    }
                  }
                }
                n608 = Select(t=State_Type_Definitions,_for_0.26g_versions_and_later_2."True Stop" ("Enum"), s=w1793, f=State_Type_Definitions,_for_0.26g_versions_and_later_2."Task 9B: Rotate to Angle" ("Enum")) -> (s? t:f=w1796:T6)
                n609 = Select(t=w1796, s=w1794, f=State_Type_Definitions,_for_0.26g_versions_and_later_2."Task 9A: Raise Arm" ("Enum")) -> (s? t:f=w1802:T6)
              }
              frame "Exit" {
                n610 = for {
                  shift-right: [w1820] -> w1817
                  shift-left: _ -> [w1821]
                  tunnel: string[] ["STOP", "RESET ENCODERS", "RESET YAW", ""] -> [w1819] mode=indexing
                  n611 = Enqueue Element(queue=w1821, element=w1819) -> (queue out=w1820:refnum<queue>)  [unwired: 2 in, 2 out]
                }
              }
            }
          }
          frame 39 {
            # ">>> yStepper command>>>"
            n612 = Dequeue Element(queue=w1834, timeout in ms (-1)=w1833, error in (no error)=w1832) -> (element=w1836:T7)  [unwired: 3 out]
            n613 = In Range and Coerce(upper limit=65.0, x=w1826, lower limit=55.0) -> (In Range?=w1823:bool)  [unwired: 1 out]
            n614 = case shown="\"None\", Default" w1836 {
              tunnel: w1827 -> [w1839 _]
              tunnel: [w1847 State_Type_Definitions,_for_0.26g_versions_and_later_2."True Stop" ("Enum")] -> w1829
              tunnel: w1835 -> [w1845 w1863]
              tunnel: [w1844 w1862] -> w1828
              tunnel: [State_Type_Definitions,_for_0.26g_versions_and_later_2."Idle" ("Enum") State_Type_Definitions,_for_0.26g_versions_and_later_2."Shutdown" ("Enum")] -> w1830
              tunnel: w1823 -> [w1837 _]
              frame "None", Default {
                n615 = Or(x=w1837, y=w1839) -> (x .or. y?=w1838:bool)
                n616 = case shown="True" w1837 {
                  tunnel: w1845 -> [w1850 w1856]
                  tunnel: [w1849 w1854] -> w1844
                  frame False {
                    n617 = for {
                      shift-right: [w1852] -> w1849
                      shift-left: w1850 -> [w1853]
                      tunnel: string[] ["READ NAVX", "R-ACW"] ("element") -> [w1851] mode=indexing
                      n618 = Enqueue Element(queue=w1853, element=w1851) -> (queue out=w1852:refnum<queue>)  [unwired: 2 in, 2 out]
                    }
                  }
                  frame True {
                    n619 = for {
                      shift-right: [w1858] -> w1854
                      shift-left: w1856 -> [w1859]
                      tunnel: string[] ["STOP", "RESET ENCODERS", "RESET YAW", ""] -> [w1857] mode=indexing
                      n620 = Enqueue Element(queue=w1859, element=w1857) -> (queue out=w1858:refnum<queue>)  [unwired: 2 in, 2 out]
                    }
                  }
                }
                n621 = Select(t=State_Type_Definitions,_for_0.26g_versions_and_later_2."True Stop" ("Enum"), s=w1839, f=State_Type_Definitions."Task 9C: Rotation alignmnet") -> (s? t:f=w1841:u16)
                n622 = Select(t=w1841, s=w1838, f=State_Type_Definitions,_for_0.26g_versions_and_later_2."Task 9B: Rotate to Angle" ("Enum")) -> (s? t:f=w1847:u16)
              }
              frame "Exit" {
                n623 = for {
                  shift-right: [w1866] -> w1862
                  shift-left: w1863 -> [w1867]
                  tunnel: string[] ["STOP", "RESET ENCODERS", "RESET YAW", ""] -> [w1865] mode=indexing
                  n624 = Enqueue Element(queue=w1867, element=w1865) -> (queue out=w1866:refnum<queue>)  [unwired: 2 in, 2 out]
                }
              }
            }
          }
          frame 39 {
            # ">>> Motor control cluster >>>"
            # ">>Line Detected>>"
            # ">>Action Queue>>"
            # ">>> yStepper command>>>"
            n625 = Dequeue Element(queue=w1878, timeout in ms (-1)=w1877, error in (no error)=w1876) -> (element=w1879:T7)  [unwired: 3 out]
            n626 = case shown="\"None\", Default" w1879 {
              tunnel: w1874 -> [w1880 _]
              tunnel: [w1890 State_Type_Definitions,_for_0.26g_versions_and_later_2."True Stop" ("Enum")] -> w1871
              tunnel: w1875 -> [w1888 w1906]
              tunnel: [w1887 w1905] -> w1870
              tunnel: [State_Type_Definitions,_for_0.26g_versions_and_later_2."Idle" ("Enum") State_Type_Definitions,_for_0.26g_versions_and_later_2."Shutdown" ("Enum")] -> w1873
              tunnel: w1868 -> [w1881 _]
              frame "None", Default {
                n627 = Or(x=w1880, y=w1881) -> (x .or. y?=w1882:bool)
                n628 = case shown="False" w1881 {
                  tunnel: w1888 -> [w1893 w1899]
                  tunnel: [w1892 w1897] -> w1887
                  frame False {
                    n629 = for {
                      shift-right: [w1895] -> w1892
                      shift-left: w1893 -> [w1896]
                      tunnel: string[] ["READ IR", "READ LINE SENSOR", "FORWARD - IR ASSIST"] ("element") -> [w1894] mode=indexing
                      n630 = Enqueue Element(queue=w1896, element=w1894) -> (queue out=w1895:refnum<queue>)  [unwired: 2 in, 2 out]
                    }
                  }
                  frame True {
                    n631 = for {
                      shift-right: [w1901] -> w1897
                      shift-left: w1899 -> [w1902]
                      tunnel: string[] ["STOP", "RESET ENCODERS", "RESET YAW", ""] -> [w1900] mode=indexing
                      n632 = Enqueue Element(queue=w1902, element=w1900) -> (queue out=w1901:refnum<queue>)  [unwired: 2 in, 2 out]
                    }
                  }
                }
                n633 = Select(t=State_Type_Definitions,_for_0.26g_versions_and_later_2."True Stop" ("Enum"), s=w1880, f=State_Type_Definitions."Task 9D: Move Forward") -> (s? t:f=w1884:u16)
                n634 = Select(t=w1884, s=w1882, f=State_Type_Definitions."Task 9C: Rotation alignmnet" ("Enum")) -> (s? t:f=w1890:u16)
              }
              frame "Exit" {
                n635 = for {
                  shift-right: [w1909] -> w1905
                  shift-left: w1906 -> [w1910]
                  tunnel: string[] ["STOP", "RESET ENCODERS", "RESET YAW", ""] -> [w1908] mode=indexing
                  n636 = Enqueue Element(queue=w1910, element=w1908) -> (queue out=w1909:refnum<queue>)  [unwired: 2 in, 2 out]
                }
              }
            }
          }
          frame 40 {
            # ">> Manual override >>"
            # ">>Table Detected>>"
            # ">>> Motor control cluster >>>"
            # ">>Line Detected>>"
            # ">>Action Queue>>"
            # ">>> yStepper command>>>"
            n637 = Less Or Equal?(x=w1912, y=15.0) -> (x <= y?=w1911:bool)
            n638 = Dequeue Element(queue=w1923, timeout in ms (-1)=w1922, error in (no error)=w1921) -> (element=w1924:T7)  [unwired: 3 out]
            n639 = case shown="\"None\", Default" w1924 {
              tunnel: w1919 -> [w1925 _]
              tunnel: [w1935 State_Type_Definitions,_for_0.26g_versions_and_later_2."True Stop" ("Enum")] -> w1916
              tunnel: w1920 -> [w1933 w1951]
              tunnel: [w1932 w1950] -> w1915
              tunnel: [State_Type_Definitions,_for_0.26g_versions_and_later_2."Idle" ("Enum") State_Type_Definitions,_for_0.26g_versions_and_later_2."Shutdown" ("Enum")] -> w1918
              tunnel: w1911 -> [w1926 _]
              frame "None", Default {
                n640 = Or(x=w1925, y=w1926) -> (x .or. y?=w1927:bool)
                n641 = case shown="True" w1926 {
                  tunnel: w1933 -> [w1938 w1944]
                  tunnel: [w1937 w1942] -> w1932
                  frame False {
                    n642 = for {
                      shift-right: [w1940] -> w1937
                      shift-left: w1938 -> [w1941]
                      tunnel: string[] ["READ IR", "FORWARD - IR ASSIST", ""] ("element") -> [w1939] mode=indexing
                      n643 = Enqueue Element(queue=w1941, element=w1939) -> (queue out=w1940:refnum<queue>)  [unwired: 2 in, 2 out]
                    }
                  }
                  frame True {
                    n644 = for {
                      shift-right: [w1946] -> w1942
                      shift-left: w1944 -> [w1947]
                      tunnel: string[] ["STOP", "RESET ENCODERS", "RESET YAW", ""] -> [w1945] mode=indexing
                      n645 = Enqueue Element(queue=w1947, element=w1945) -> (queue out=w1946:refnum<queue>)  [unwired: 2 in, 2 out]
                    }
                  }
                }
                n646 = Select(t=State_Type_Definitions,_for_0.26g_versions_and_later_2."True Stop" ("Enum"), s=w1925, f=State_Type_Definitions,_for_0.26g_versions_and_later_2."True Stop") -> (s? t:f=w1929:T6)
                n647 = Select(t=w1929, s=w1927, f=State_Type_Definitions."Task 9D: Move Forward" ("Enum")) -> (s? t:f=w1935:u16)
              }
              frame "Exit" {
                n648 = for {
                  shift-right: [w1954] -> w1950
                  shift-left: w1951 -> [w1955]
                  tunnel: string[] ["STOP", "RESET ENCODERS", "RESET YAW", ""] -> [w1953] mode=indexing
                  n649 = Enqueue Element(queue=w1955, element=w1953) -> (queue out=w1954:refnum<queue>)  [unwired: 2 in, 2 out]
                }
              }
            }
          }
          frame 41 {
            # ">> Stepper height reeached >>"
            # ">>> yStepper command>>>"
            # ">> Manual override >>"
            n650 = Dequeue Element(queue=w1966, timeout in ms (-1)=w1961, error in (no error)=w1965) -> (element=w1969:T7)  [unwired: 3 out]
            n651 = Equal?(x=w1963, y=u8 40) -> (x = y?=w1967:bool)
            n652 = case shown="\"None\", Default" w1969 {
              tunnel: [w1980 State_Type_Definitions,_for_0.26g_versions_and_later_2."True Stop" ("Enum")] -> w1959
              tunnel: [w1978 w1996] -> w1958
              tunnel: w1962 -> [w1977 w1993]
              tunnel: w1964 -> [w1971 _]
              tunnel: [State_Type_Definitions,_for_0.26g_versions_and_later_2."Idle" ("Enum") State_Type_Definitions,_for_0.26g_versions_and_later_2."Shutdown" ("Enum")] -> w1960
              tunnel: w1967 -> [w1970 _]
              frame "None", Default {
                # ">> WIill proceed to part ii if not manual override >>"
                # ">>If ENABLE or Trigger is set to true>>"
                n653 = Or(x=w1970, y=w1971) -> (x .or. y?=w1972:bool)
                n654 = case shown="False" w1970 {
                  tunnel: [w1983 w1989] -> w1978
                  tunnel: w1977 -> [w1982 w1988]
                  frame False {
                    n655 = for {
                      shift-right: [w1985] -> w1983
                      shift-left: w1982 -> [w1986]
                      tunnel: string[] ["Z STEPPER BOX HEIGHT", "READ STEPPER VALUES"] ("element") -> [w1984] mode=indexing
                      n656 = Enqueue Element(queue=w1986, element=w1984) -> (queue out=w1985:refnum<queue>)  [unwired: 2 in, 2 out]
                    }
                  }
                  frame True {
                    n657 = for {
                      shift-right: [w1991] -> w1989
                      shift-left: w1988 -> [w1992]
                      tunnel: string[] ["READ IR", "", "", "", "", ""] -> [w1990] mode=indexing
                      n658 = Enqueue Element(queue=w1992, element=w1990) -> (queue out=w1991:refnum<queue>)  [unwired: 2 in, 2 out]
                    }
                  }
                }
                n659 = Select(t=State_Type_Definitions,_for_0.26g_versions_and_later_2."True Stop" ("Enum"), s=w1971, f=State_Type_Definitions."Task A: MOVE FORWARD" ("Enum")) -> (s? t:f=w1974:u16)
                n660 = Select(t=w1974, s=w1972, f=State_Type_Definitions."Task A: RAISE ARM TO HEIGHT" ("Enum")) -> (s? t:f=w1980:u16)
              }
              frame "Exit" {
                n661 = for {
                  shift-right: [w1999] -> w1996
                  shift-left: w1993 -> [w2000]
                  tunnel: string[] ["STOP", "RESET ENCODERS", "RESET YAW", ""] -> [w1998] mode=indexing
                  n662 = Enqueue Element(queue=w2000, element=w1998) -> (queue out=w1999:refnum<queue>)  [unwired: 2 in, 2 out]
                }
              }
            }
          }
          frame 42 {
            # ">>> Motor control cluster >>>"
            # ">>> yStepper command>>>"
            # ">>Object detected>>"
            n663 = Dequeue Element(queue=w2009, timeout in ms (-1)=w2008, error in (no error)=w2007) -> (element=w2014:T7)  [unwired: 3 out]
            n664 = Less Or Equal?(x=w2003, y=30.0) -> (x <= y?=w2001:bool)
            "Table obstruct" <- w2001
            n665 = case shown="\"None\", Default" w2014 {
              tunnel: w2001 -> [w2017 _]
              tunnel: [w2024 State_Type_Definitions,_for_0.26g_versions_and_later_2."True Stop" ("Enum")] -> w2013
              tunnel: w2006 -> [w2016 _]
              tunnel: w2010 -> [w2023 w2040]
              tunnel: [w2022 w2041] -> w2012
              tunnel: [State_Type_Definitions,_for_0.26g_versions_and_later_2."Idle" ("Enum") State_Type_Definitions,_for_0.26g_versions_and_later_2."Shutdown" ("Enum")] -> w2011
              frame "None", Default {
                n666 = case shown="False" w2017 {
                  tunnel: w2023 -> [w2027 w2034]
                  tunnel: [w2028 w2033] -> w2022
                  frame False {
                    n667 = for {
                      tunnel: string[] ["READ IR", "FORWARD", "READ NAVX"] ("element") -> [w2029] mode=indexing
                      shift-right: [w2031] -> w2028
                      shift-left: w2027 -> [w2030]
                      n668 = Enqueue Element(queue=w2030, element=w2029) -> (queue out=w2031:refnum<queue>)  [unwired: 2 in, 2 out]
                    }
                  }
                  frame True {
                    n669 = for {
                      shift-right: [w2036] -> w2033
                      shift-left: w2034 -> [w2037]
                      tunnel: string[] ["RESET ENCODERS", "READ NAVX", "READ ENCODERS"] -> [w2035] mode=indexing
                      n670 = Enqueue Element(queue=w2037, element=w2035) -> (queue out=w2036:refnum<queue>)  [unwired: 2 in, 2 out]
                    }
                  }
                }
                n671 = Or(x=w2017, y=w2016) -> (x .or. y?=w2015:bool)
                n672 = Select(t=State_Type_Definitions,_for_0.26g_versions_and_later_2."True Stop" ("Enum"), s=w2016, f=State_Type_Definitions,_for_0.26g_versions_and_later_2."True Stop" ("Enum")) -> (s? t:f=w2018:T6)
                n673 = Select(t=w2018, s=w2015, f=State_Type_Definitions."Task A: MOVE FORWARD" ("Enum")) -> (s? t:f=w2024:u16)
              }
              frame "Exit" {
                n674 = for {
                  shift-right: [w2044] -> w2041
                  shift-left: w2040 -> [w2045]
                  tunnel: string[] ["STOP", "RESET ENCODERS", "RESET YAW", "ARDUINO MODE 0"] -> [w2043] mode=indexing
                  n675 = Enqueue Element(queue=w2045, element=w2043) -> (queue out=w2044:refnum<queue>)  [unwired: 2 in, 2 out]
                }
              }
            }
          }
        }
      }
    }
    n676 = local write "Green LED"(w191) -> ()
  }
  n677 = while {
    tunnel: w46 -> [w2710]
    tunnel: w45 -> [w2707]
    stop <- w2704 stop-if-true
    # "Status Loop for Action Queues"
    n678 = Get Queue Status(queue=w2710, return elements? (F)=TRUE) -> (error out=w2706:errorcluster, # elements in queue=→"Action Queue Items":i32, elements=→"Action Queues items":string[])  [unwired: 1 in, 5 out]
    n679 = Get Queue Status(queue=w2707, return elements? (F)=TRUE) -> (# pending remove=→"State Logic Queue Items":i32, error out=w2705:errorcluster, elements=→"elements":T7[])  [unwired: 1 in, 5 out]
    n680 = Merge Errors(w2706, w2705) -> (w2704:errorcluster)
    n681 = Wait (ms)(milliseconds to wait=u32 500) -> ()  [unwired: 1 out]
  }
  n682 = call <vilib>:"DIO Close.vi"("error in (no error)"=w22, "DIO Info In"=w25) -> ()  [unwired: 9 in, 1 out]
  n683 = call <vilib>:"DIO Close.vi"("error in (no error)"=w32, "DIO Info In"=w34) -> ()  [unwired: 9 in, 1 out]
  n684 = call <vilib>:"NavX Close.vi"("error in (no error)"=w9, "NavX Info In"=w8) -> ()  [unwired: 9 in, 1 out]
  n685 = call <vilib>:"DIO Close.vi"("error in (no error)"=w27, "DIO Info In"=w29) -> ()  [unwired: 9 in, 1 out]
  n686 = call <vilib>:"DIO Close.vi"("error in (no error)"=w16, "DIO Info In"=w17) -> ()  [unwired: 9 in, 1 out]
  n687 = call <vilib>:"DIO Close.vi"("error in (no error)"=w11, "DIO Info In"=w12) -> ()  [unwired: 9 in, 1 out]
  n688 = while {
    stop <- w2714 stop-if-true
    n689 = call <vilib>:"RT Get CPU Loads.vi"() -> ("CPU loads"=→"CPU loads":T5[])  [unwired: 10 in, 1 out]
    n690 = Wait (ms)(milliseconds to wait=u32 100) -> ()  [unwired: 1 out]
    n691 = call "FGV Stop.vi"("Init/Read/Write State"=States_for_Action_Engine."Read") -> ("Output node"=w2714:bool)  [unwired: 2 in, 1 out]
  }
  n692 = while {
    stop <- w2718 stop-if-true
    n693 = call "MOTOR CONTROL WITH PID AE.vi"("AE Mode"=MOTOR_CONTROL_WITH_PID_AE_DATA_MODE_TYPE_DEF."Read from AE") -> ("Speed & distance"=→"Speed & distance":T1)  [unwired: 3 in]
    n694 = call "FGV Stop.vi"("Init/Read/Write State"=States_for_Action_Engine."Read") -> ("Output node"=w2718:bool)  [unwired: 2 in, 1 out]
    n695 = Wait (ms)(milliseconds to wait=u32 5) -> ()  [unwired: 1 out]
  }
  n696 = Merge Errors "Merge Errors"(w62, w61) -> (w44:errorcluster)
  n697 = Merge Errors(w48, w44) -> (w43:errorcluster)
  n698 = Destroy User Event(user event=w65, error in=w43) -> ()  [unwired: 1 out]
  n699 = Destroy User Event(user event=w66, error in=w43) -> ()  [unwired: 1 out]
  n700 = Unregister For Events(event registration refnum=w57, error in=w43) -> ()  [unwired: 1 out]
  n701 = Release Queue(queue=w39, error in (no error)=w43) -> (error out=→"error out":errorcluster)  [unwired: 1 in, 2 out]
  n702 = Release Queue(queue=w56, error in (no error)=w43) -> ()  [unwired: 1 in, 3 out]
